vi "ControlProgram5.1.vi"() -> ()   [LabVIEW 2016]
uses:
  <vilib>/Utility/error.llb/DialogType.ctl
  <vilib>/Utility/miscctls.llb/LVPoint32TypeDef.ctl
  <vilib>/DAQmx/write.llb/DAQmx Write (Digital Bool 1Line 1Point).vi
  <vilib>/DAQmx/create/channels.llb/DAQmx Create Channel (DO-Digital Output).vi
  <vilib>/platform/TimedLoop/XDataNode/XDataNode.xnode
  <vilib>/Platform/TimedLoop/XDataNode/nitl_modes.ctl
  <vilib>/Platform/TimedLoop/XDataNode/XDNodeRunTimeDep.lvlib
  <vilib>/Platform/TimedLoop/XDataNode/wakeup.ctl
  <vilib>/Platform/TimedLoop/XDataNode/timing_clust.ctl
  <vilib>/DAQmx/create/channels.llb/DAQmx Create Channel (AI-Voltage-Basic).vi
  <vilib>/DAQmx/create/channels.llb/DAQmx Create Channel (AO-Voltage-Basic).vi
  <vilib>/DAQmx/write.llb/DAQmx Write (Analog 1D DBL NChan 1Samp).vi
  <resource>/objmgr/daqmx.rc
  <vilib>/Analysis/NI_AALBase.lvlib
  <vilib>/Analysis/baseanly.llb/Mean (DBL).vi
  <vilib>/Instr/_visa.llb/VISA Configure Serial Port (Instr).vi
  <vilib>/DAQmx/read.llb/DAQmx Read (Analog 2D DBL NChan NSamp).vi
  <vilib>/Utility/inputDevices.llb/closeMouse.vi
  <vilib>/Utility/inputDevices.llb/mouseAcquire.vi
  <vilib>/DAQmx/configure/timing.llb/DAQmx Timing (Sample Clock).vi
panel:
  out "Flush Sample Start Time":u32
  out "Sample flush time (s)":dbl=100.0
  in  "Inject Sample":bool
  out "Chart Freq (Hz)":dbl
  out "Waveform Chart 3":dbl[][](graph)
  out "Cal values":T1={"AX alpha"=672.9952101249002, "BX alpha"=822.8320399167465, "AX kappa"=0.3432739170419873, "BX kappa"=0.22087046979741862, "AX offset"=-0.002065833400375715, "BX offset"=0.010483360643544744, "AY alpha"=702.0654168010462, "BY alpha"=773.6701766674906, "AY kappa"=0.33643150106915, "BY kappa"=0.2444549177225145, "AY offset"=-0.1177594339643395, "BY offset"=0.06470506082263472}
  in  "Inject Pump 1":bool
  in  "Inject Pump 2":bool
  in  "Tab Control 2":T2(tab)
  in  "Force FB script":bool
  in  "Got ADig bead":bool
  in  "Move Cap. 2 (ADig Top)":bool
  in  "Dump beads":bool
  in  "Got DNA bead":bool
  in  "Delta after tether":dbl=3.1
  in  "TA Cancel Save?":bool
  in  "Min fish\ndelta (V)":dbl=2.8 min=0.0 max=10.0 step=0.1
  in  "Max fish\ndelta (V)":dbl=3.8 min=0.0 max=10.0 step=0.1
  in  "Fish Speed (ms)":i32=3000
  in  "Wait (ms)":i32=1500
  in  "# attempts":dbl=10.0
  in  "Cutoff force (pN)":dbl=5.0
  in  "Raster after\n tether?":bool=TRUE
  out "Tether":bool
  out "Attempt #":i32
  in  "Cal @ Delta (V)":dbl=5.0
  in  "Cal stage position":i32=3
  in  "Conv Y (nm/V)":dbl=505.0
  in  "Conv X (nm/V)":dbl=892.0
  out "Cal Final Sampling Rate":dbl
  in  "Cal Averaging":i32=1
  in  "Wait before dip (s)":dbl=3.0
  in  "Start dipping after?":bool
  in  "Start trap delta (V)":dbl=3.85
  in  "Cancel dwell":bool
  in  "Pause dwell":bool
  in  "Return position":dbl=3.0
  in  "Dip duration":dbl=15.0
  in  "Dip position":dbl=4.0
  in  "Dip":bool
  out "Dip time":i32
  in  "Stop":bool=TRUE
  in  "?":T3(tab)=enum."Mouse control"
  in  "Save N sets":bool
  in  "N sets":i32=200
  in  "Cal sets to save":i32=500
  in  "Reset data stream":bool
  out "Buffer Overflow":bool
  out "Stage moving":bool
  in  "Comment":string="wtUvrD 0.5 uM ATP"
  in  "Raster scan":bool
  out "Saving":bool
  in  "Save cal":bool
  in  "Save Data":bool
  in  "Stop saving":bool
  out "Calibrating":bool
  out "Progress":dbl(slide) scale=0.0..100.0
  in  "Read Cal":bool
  in  "Fish":bool
  in  "Averaging Number":i32=1250
  out "Final Sampling Rate":dbl=100.0
  in  "Trap position":cluster{"X":dbl, "Y":dbl}={"X"=1.6, "Y"=4.95}
  in  "Trap delta":dbl=5.1 min=0.0 max=10.0 step=0.1
  in  "Fixed X":dbl=1.6
  in  "Fixed Y":dbl=0.7
  in  "Shutter 1 (B)":bool
  in  "Shutter 2 (A)":bool
  in  "Pulling direction":bool=TRUE
  out "Raster scanning...":bool
  out "Current file name":path
  in  "AX alpha":dbl format="%#_3p"
  in  "BX alpha":dbl format="%#_3g"
  in  "AX kappa":dbl format="%#_3g"
  in  "BX kappa":dbl format="%#_3g"
  in  "AX offset":dbl format="%#_3g"
  in  "BX offset":dbl format="%#_3g"
  in  "AY alpha":dbl format="%#_3g"
  in  "BY alpha":dbl format="%#_3g"
  in  "AY kappa":dbl format="%#_3g"
  in  "BY kappa":dbl format="%#_3g"
  in  "AY offset":dbl format="%#_3g"
  in  "BY offset":dbl format="%#_3g"
  out "Buffer status":u8(slide) scale=0.0..100.0
  in  "dump spot":string="Dump beads spot"
  in  "up flow spot":string="Upper flow spot"
  in  "low flow spot":string="Lower flow spot"
  in  "up cap":string="Upper capillary (ADig beads)"
  in  "bottom cap":string="Lower capillary (DNA beads)"
  in  "Move to Position 5":bool
  in  "Set Position 5":bool
  in  "Saved stage positions":dbl[][](array[numeric])=[[1.0, 0.0, 0.0, 0.0], [2.0, 0.28481, -2.63158, -0.02256], [3.0, 1.27978, -0.73974, 0.0], [4.0, 1.27978, -2.1978, 0.0], [5.0, 0.03306, -2.63158, -0.02256]]
  in  "Set Position 2":bool
  in  "Move to Position 2":bool
  in  "Set Position 1":bool
  in  "Move to Position 1":bool
  in  "Set Position 4":bool
  in  "Move to Position 4":bool
  in  "Set Position 3":bool
  in  "Move to Position 3":bool
  out "Stage error":errorcluster
  in  "Clear Volume":bool
  out "Sample Flush Meter":u8(slide) scale=0.0..100.0
  out "Flushing Sample":bool
  in  "Flush Sample":bool
  in  "Normal \nRate (ul/hr)  3":dbl=100.0
  in  "Normal \nVolume (ul) 3":dbl=300.0
  in  "Normal \nVolume (ul) 2":dbl
  in  "Normal \nRate (ul/hr)":dbl
  in  "Normal \nVolume (ul)":dbl
  in  "Flush\nRate (ul/min)":dbl
  in  "Flush\nVolume (ul)":dbl
  in  "Flush \nRate (ul/min)  2":dbl
  in  "Flush Pump 2":bool
  in  "Flush\nVolume (ul)  2":dbl
  in  "Flush Pump 1":bool
  in  "Normal \nRate (ul/hr)  2":dbl
  in  "Write Wait":i32=1000
  in  "Flush \nRate (ul/min)  3":dbl=100.0
  in  "Flush\nVolume (ul)  3":dbl=100.0
  out "error out":errorcluster
  in  "Use Mouse to Move Trap?":bool
  in  "Pause Mouse/Mirror Connection":bool
  out "Reference Voltage":cluster{dbl, dbl}={0.0, -0.0}
  out "Saved voltage":cluster{dbl, dbl}
  out "Real Coordinates":cluster{"Horizontal":i32, "Vertical":i32}={"Horizontal"=145, "Vertical"=-1746}
  out "CoordinatesMousePressed":T4
  out "Sum error":dbl(knob) scale=-0.2..0.2
  out "Trap sep":waveform(dbl)[](graph)
  in  "Set reading to\nsetpoint":bool
  in  "Offset Y (nm)":dbl format="%0.2f"
  in  "Offset X (nm)":dbl format="%0.2f"
  in  "Remove offsets":bool
  in  "Force Feedback":bool
  out "Feedback Output Voltage 2":cluster{dbl, dbl} {"?" format="%#_4g"; "?" format="%#_4g"}
  in  "Max value X":dbl=10.0 format="%.1f"
  in  "Min value X":dbl format="%0.1f"
  in  "Max value Y":dbl=10.0 format="%.1f"
  in  "Min value Y":dbl format="%.1g"
  in  "Offset":cluster{"Off Y":dbl, "Off X":dbl}={"Off Y"=1.5, "Off X"=0.17}
  in  "Setpoint voltage":cluster{"SP Y":dbl, "SP X":dbl}={"SP Y"=0.6, "SP X"=0.0}
  in  "Feedback const":T5={"Ki_B_Y"=0.5, "Ki_B_X"=0.0, "Kp Y"=1.0, "Kp X"=0.0}
  out "Mean Trap Pos X 2 (nm)":dbl format="%0.2f"
  out "Mean Trp Pos Y 2 (nm)":dbl format="%0.2f"
  out "T2 X RMS (A)":dbl format="%0.2f"
  out "T2 Y RMS (A)":dbl format="%0.2f"
  in  "Save scans":bool=TRUE
  in  "# scans":i32=1
  in  "Speed (ms)":i32=10000
  in  "Min delta":dbl=3.2
  in  "Load param":bool
  in  "Max delta":dbl=4.1
  in  "Scan Parameters":T6(array[cluster])=[{"Label"="Offset", "Max delta 2"=3.8, "Min delta 2"=2.4, "Speed (ms) 2"=10000, "# scans 2"=1}]
  in  "Trap delta\nafter":dbl=3.6
  in  "Stop raster":bool
  out "Scan Range (nm)":dbl
  out "Scan Speed (nm/s)":dbl
  out "Continue to display?":bool
  out "Video Error":errorcluster
  in  "# Samples/channel (in)":i32=40000 format="%.2f"
  out "Buffer size\n(Samples/channel)":u32
  out "DAQ rate\n(Samples/s)":dbl format="%#_6p"
  out "# Samples/channel":i32=1250
  out "# Samples/channel/s":dbl
  out "AvailSampPerChan":u32
  out "Data update period (s/set)":dbl format="%#_6p"
  out "AvailSampPerChan 2":u32
  in  "PC samp per channel":i32=1000
  in  "Sampling Rate":dbl=125000.0 format="%0.0p"
  in  "DAQ Rate2":dbl=1000000.0 format="%#_6p"
  out "Data period (s)":dbl format="%#_6p"
  in  "Tether break\nforce (pN)":dbl=1.0
  in  "Path":path=path "D:/data"
  in  "Save file index":dbl
  out "Mirror task":refnum<k21>
  in  "HWP1":string="Half waveplate 1: differential trap power"
  in  "HWP0":string="Half waveplate 0: total trap power"
  in  "Move 1":bool
  in  "\"Degrees\" 1":dbl
  in  "Move 0":bool
  in  "\"Degrees\" 0":dbl
  out "Chamber":T7(plugin-control)
  out "Deflection":T4
  in  "Sampling Rate":dbl=125000.0 format="%0.2f"
  in  "Averaging Number":i32=12500
  in  "DAQ Rate":dbl=1000000.0
  out "Final Sampling Rate":dbl
  in  "Tab Control":T8(tab)
  in  "Downsamp\nfact":dbl=250.0
  out "Bead sep":waveform(dbl)[](graph)
  out "Force (pN)":waveform(dbl)[](graph)
  out "Mean force (pN)":dbl format="%0.2f"
  out "Force noise (pN)":dbl format="%0.2f"
  out "Mean Bead Sep\n(nm)":dbl format="%0.2f"
  out "Bead Sep Noise\n(A)":dbl format="%0.2f"
  out "PSD 2":cluster{dbl[], dbl[]}(graph)
  out "PSD 1":cluster{dbl[], dbl[]}(graph)
  out "PSD 1 Sum":dbl(slide) scale=0.0..10.0
  out "PSD 2 Sum":dbl(slide) scale=0.0..10.0
  in  "Start":bool
  out "All signals":waveform(dbl)[](graph)
  # "Bead Calibration"
  # "X"
  # "Y"
  # "Pump #1 Controls"
  # "Pump #2 Controls"
  # "Sample Pump Controls"
  # "Retract the pumps manually. Change it back to INFUSE when you're done. Suck it up, don't whine."
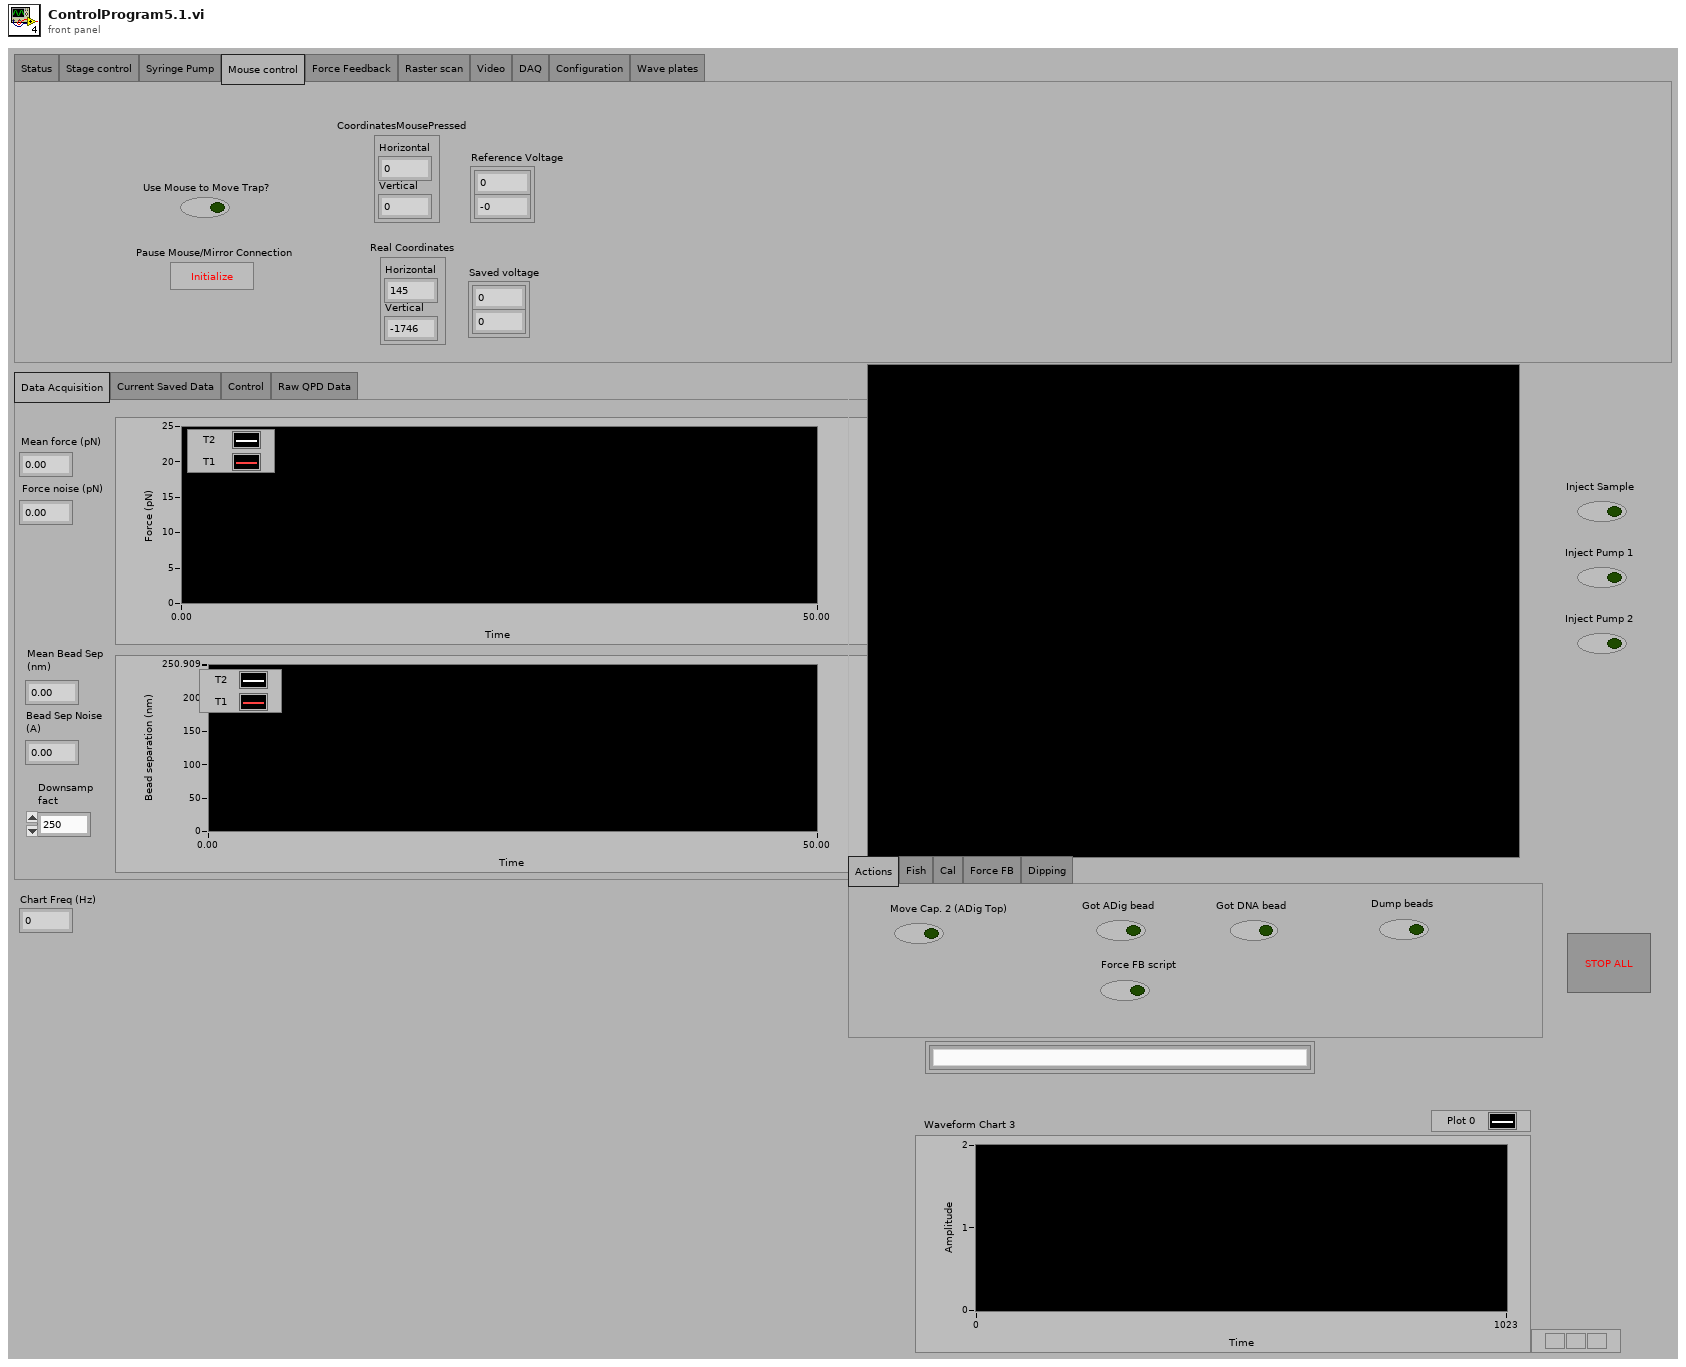
[diagram p1: front panel]
types:
  T1 = cluster{"AX alpha":dbl, "BX alpha":dbl, "AX kappa":dbl, "BX kappa":dbl, "AX offset":dbl, "BX offset":dbl, "AY alpha":dbl, "BY alpha":dbl, "AY kappa":dbl, "BY kappa":dbl, "AY offset":dbl, "BY offset":dbl}
  T2 = enum32{"Actions", "Fish", "Cal", "Force FB", "Dipping"}
  T3 = enum32{"Status", "Stage control", "Syringe Pump", "Mouse control", "Force Feedback", "Raster scan", "Video", "DAQ", "Configuration", "Wave plates"}
  T4 = typedef "LVPoint32TypeDef.ctl" = cluster{"Horizontal":i32, "Vertical":i32}
  T5 = cluster{"Ki_B_Y":dbl, "Ki_B_X":dbl, "Kp Y":dbl, "Kp X":dbl}
  T6 = cluster{"Label":string, "Max delta 2":dbl, "Min delta 2":dbl, "Speed (ms) 2":i32, "# scans 2":i32}[]
  T7 = typedef "IMAQ Image.ctl" = refnum<image>
  T8 = enum32{"Data Acquisition", "Current Saved Data", "Control", "Raw QPD Data"}
  T9 = enum16{"open", "replace", "create", "open or create", "replace or create", "replace or create with confirmation"}
  T10 = enum16{"big-endian, network order", "native, host order", "little-endian"}
  T11 = cluster{string, string, string, string, string, string, string, string}
  T12 = typedef "XDNodeRunTimeDep.lvlib/timing_clust.ctl" = cluster{"Expected End [f-1]":u64, "Actual End [f-1]":u64, "Finished Late? [f-1]":bool, "Expected End [i-1]":u64, "Actual End [i-1]":u64, "Finished Late? [i-1]":bool, "Expected Start [i]":u64, "Actual Start [i]":u64, "Expected Start [f]":u64, "Actual Start [f]":u64, "Source Name":string, "Structure Name":string, "Period":i64, "Deadline":i64, "Offset":i64, "Start":i64, "Priority":i32, "Timeout":i32, "Mode":T13, "Wakeup Reason":T14, "Error":errorcluster, "Source Type":string, "Secondary Source Type":string, "Global End Time":u64, "Global Start Time":u64, "Frame Duration":u64, "Iteration Duration":u64, "Assigned CPU":i32, "I/O Scan Engine Mode":u32}
  T13 = typedef "XDNodeRunTimeDep.lvlib/nitl_modes.ctl" = enum32{"No Change", "Process missed periods, maintain original phase", "Discard missed periods, maintain original phase", "Process missed periods, ignore original phase", "Discard missed periods, ignore original phase"}
  T14 = typedef "XDNodeRunTimeDep.lvlib/wakeup.ctl" = enum32{"Normal", "Aborted", "Asynchronous wakeup", "Timing source error", "Timed loop error", "Timeout"}
  T15 = typedef "DialogType.ctl" = u16
  T16 = cluster{"button 1":bool, "button 2":bool, "button 3":bool, "button 4":bool}
  T17 = cluster{"[0]":dbl, "[1]":dbl, "[2]":dbl, "[3]":dbl, "[4]":dbl, "[5]":dbl, "[6]":dbl, "[7]":dbl, "[8]":dbl, "[9]":dbl, "[10]":dbl, "[11]":dbl}
  T18 = cluster{"Label":string, "Max delta 2":dbl, "Min delta 2":dbl, "Speed (ms) 2":i32, "# scans 2":i32}
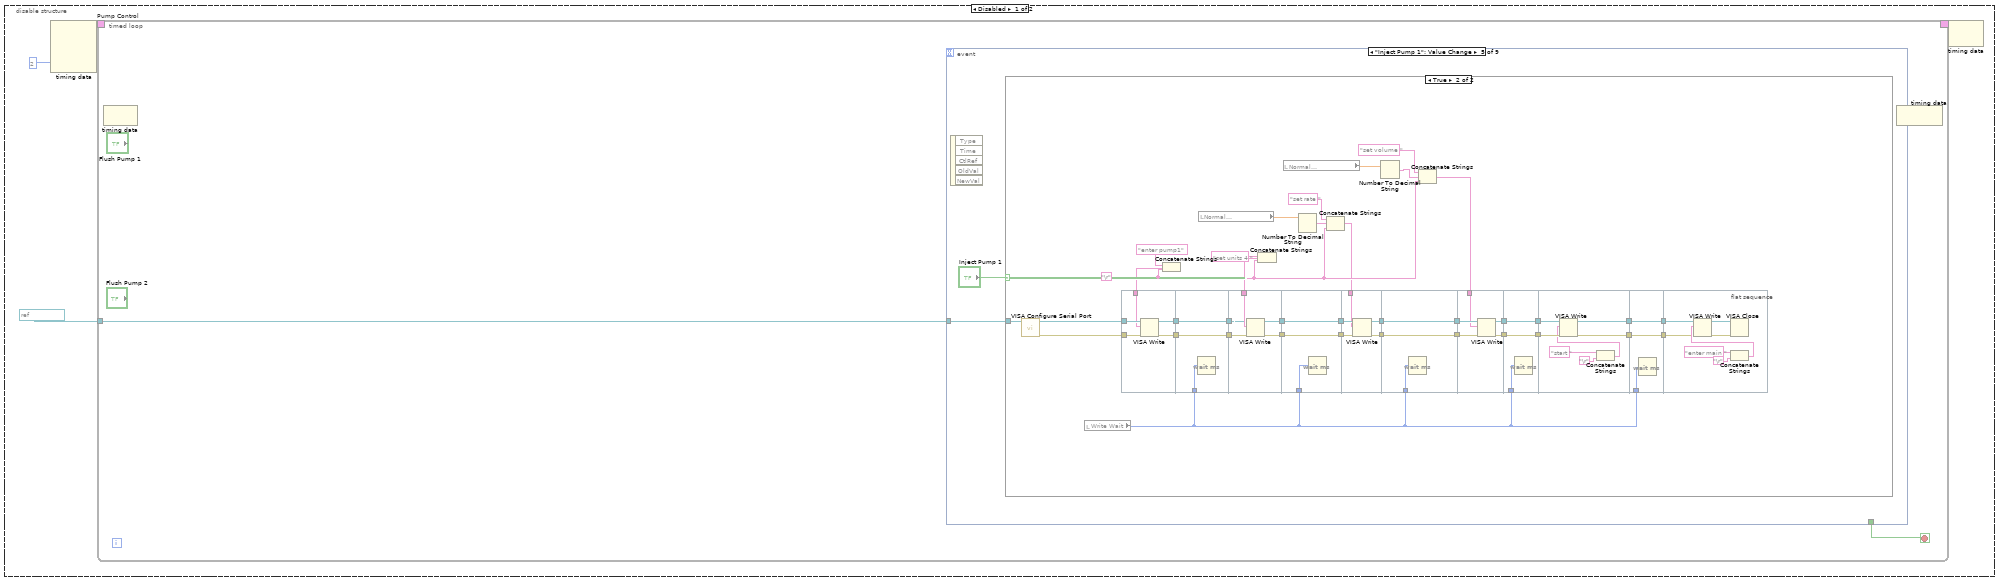
[diagram p2: hidden frame]
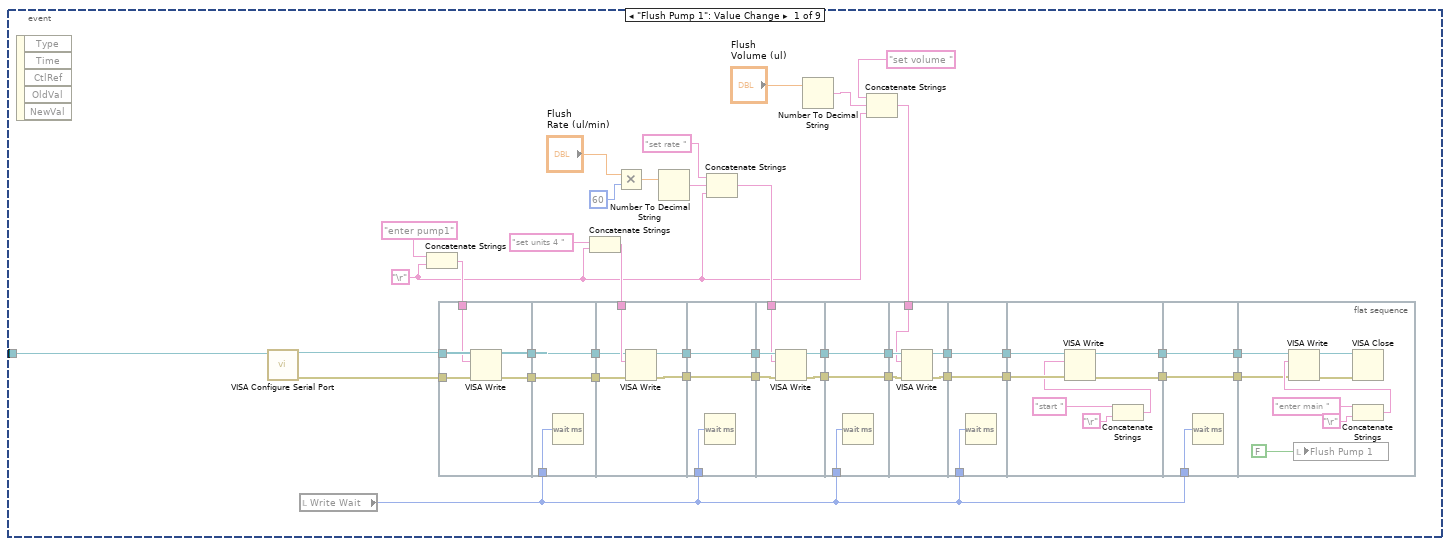
[diagram p3: hidden frame]
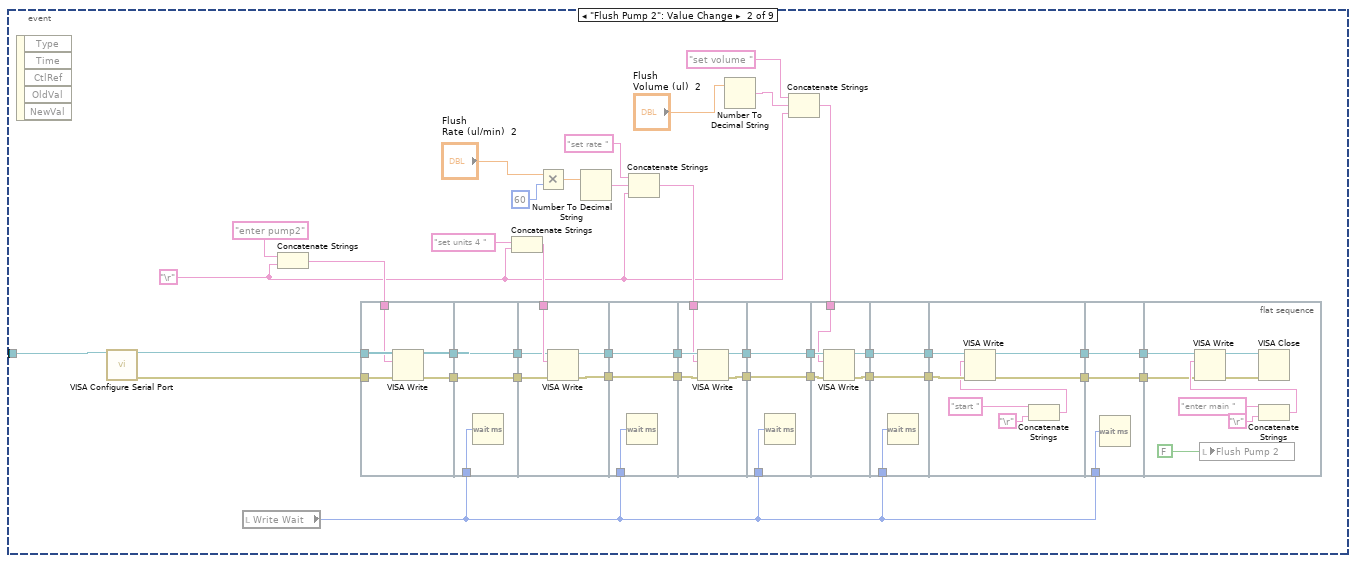
[diagram p4: hidden frame]
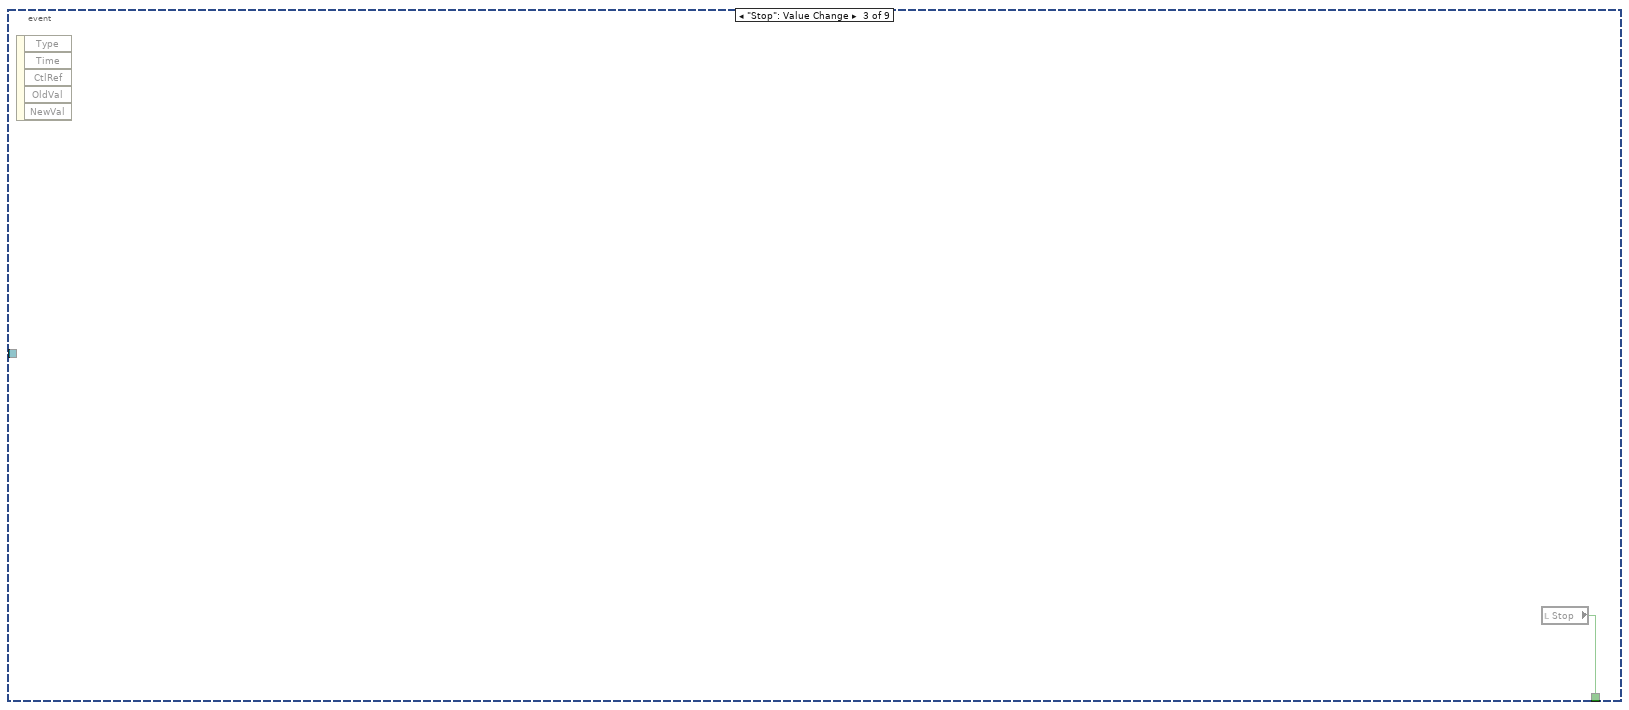
[diagram p5: hidden frame]
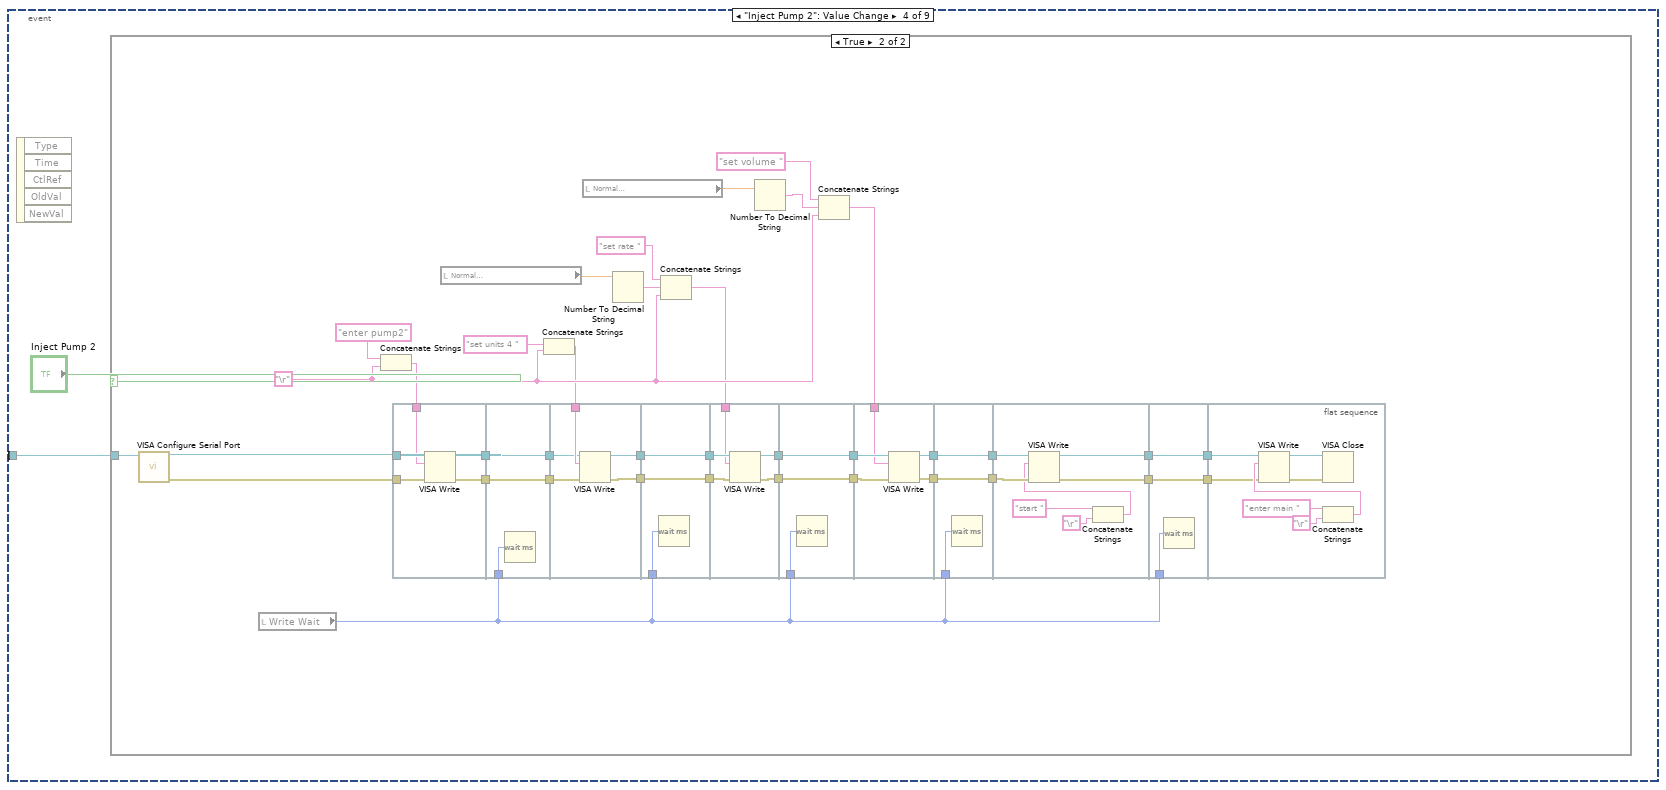
[diagram p6: hidden frame]
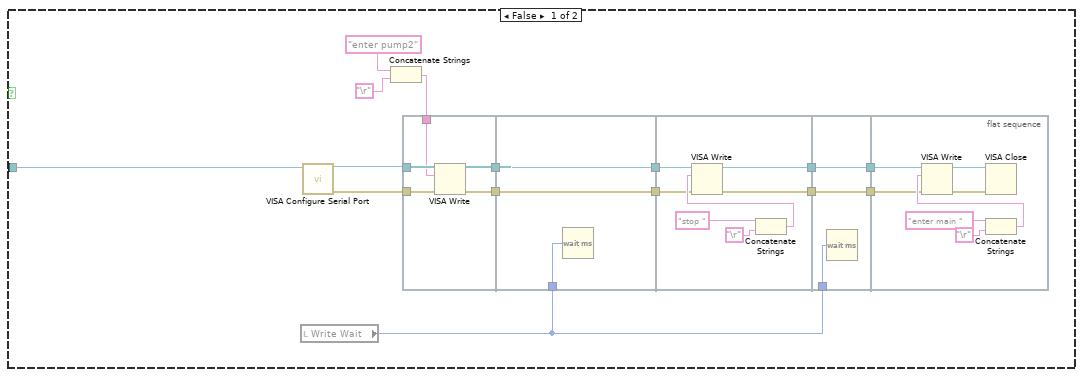
[diagram p7: hidden frame]
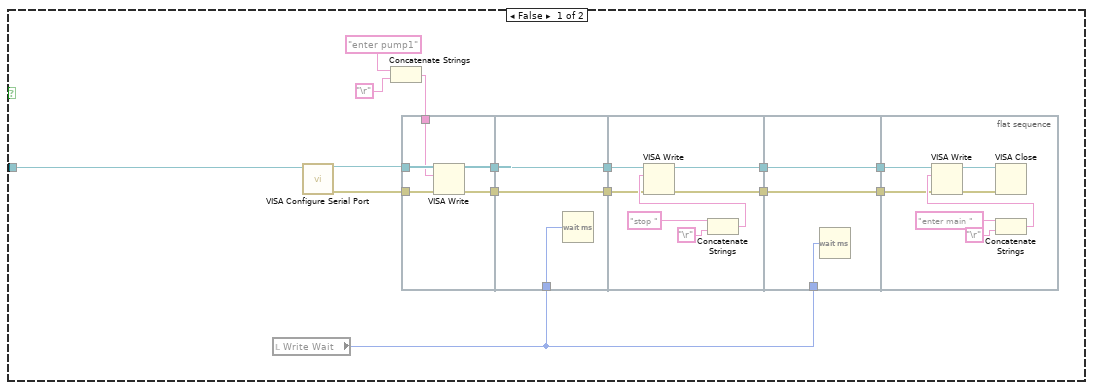
[diagram p8: hidden frame]
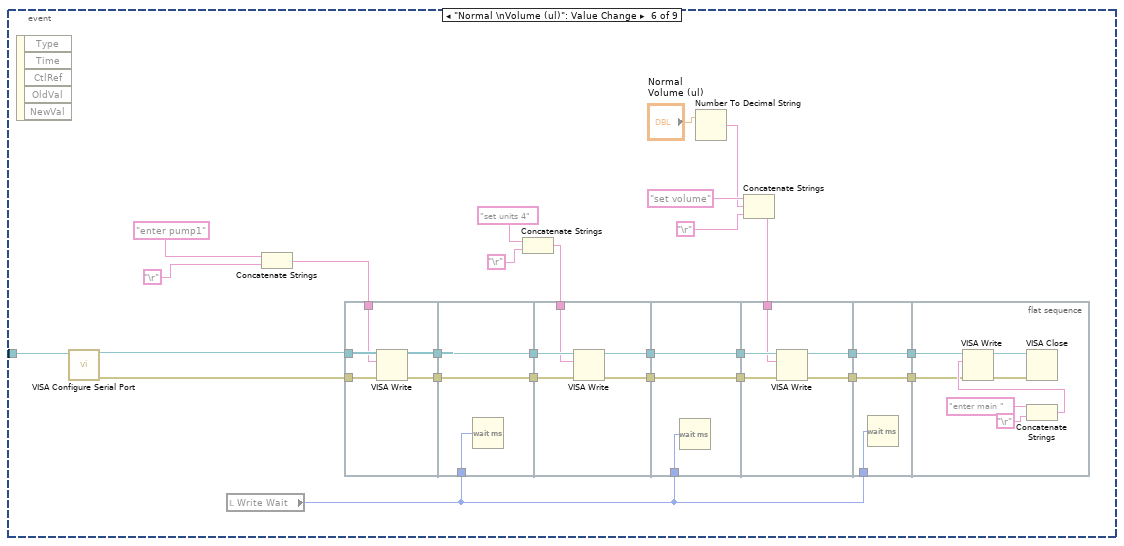
[diagram p9: hidden frame]
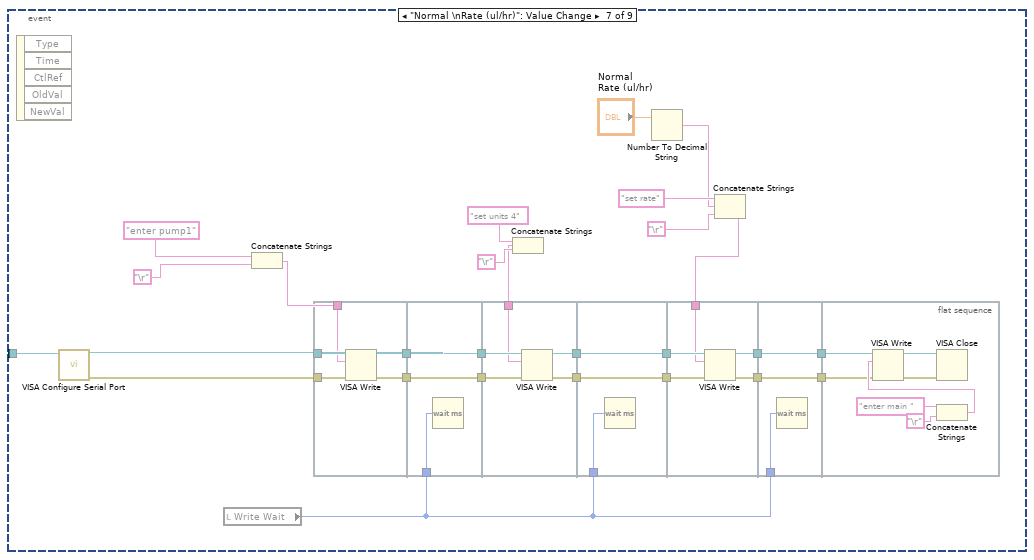
[diagram p10: hidden frame]
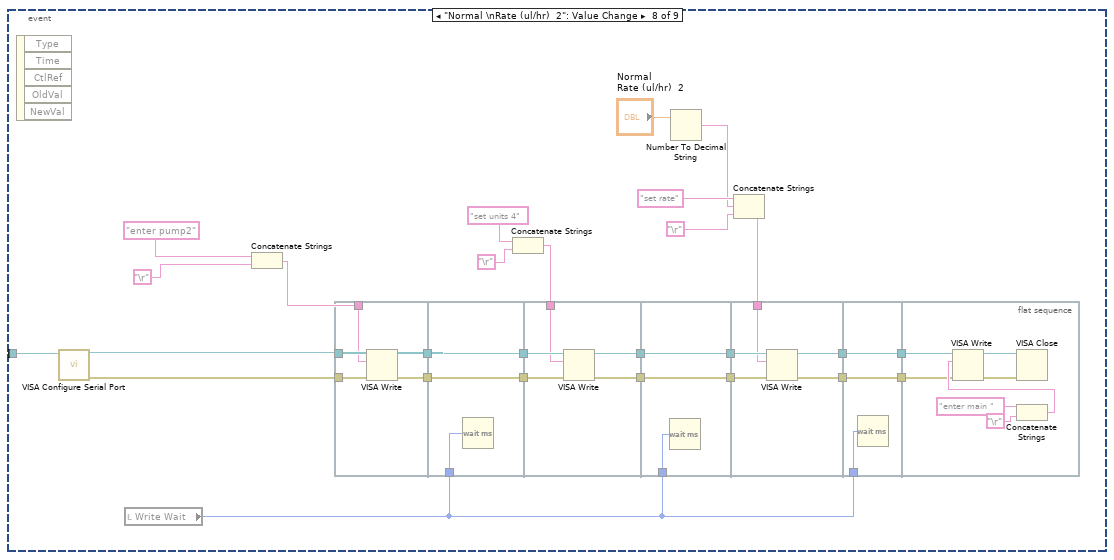
[diagram p11: hidden frame]
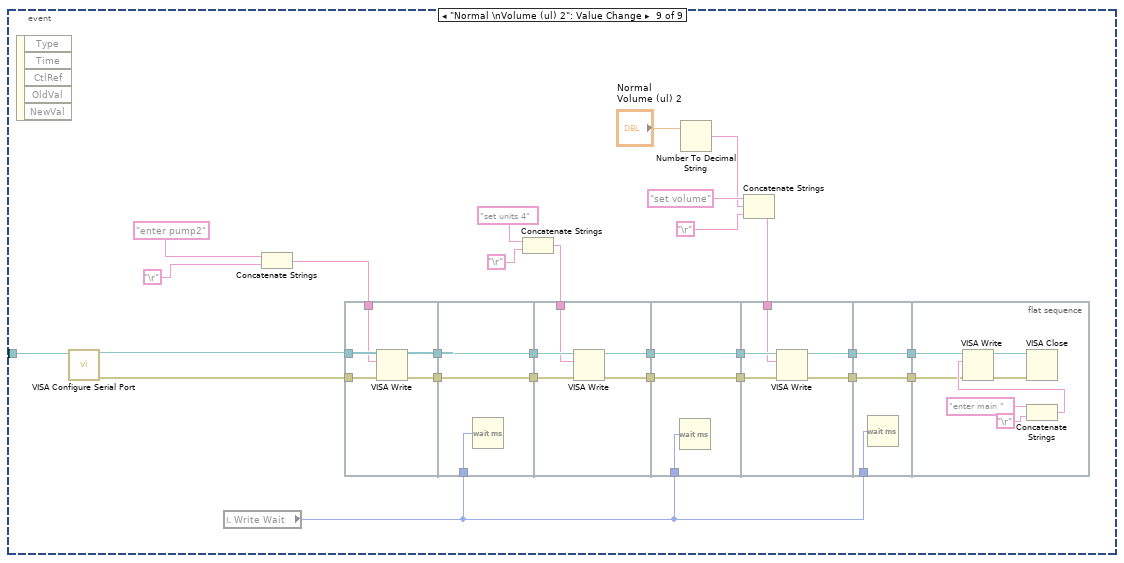
[diagram p12: hidden frame]
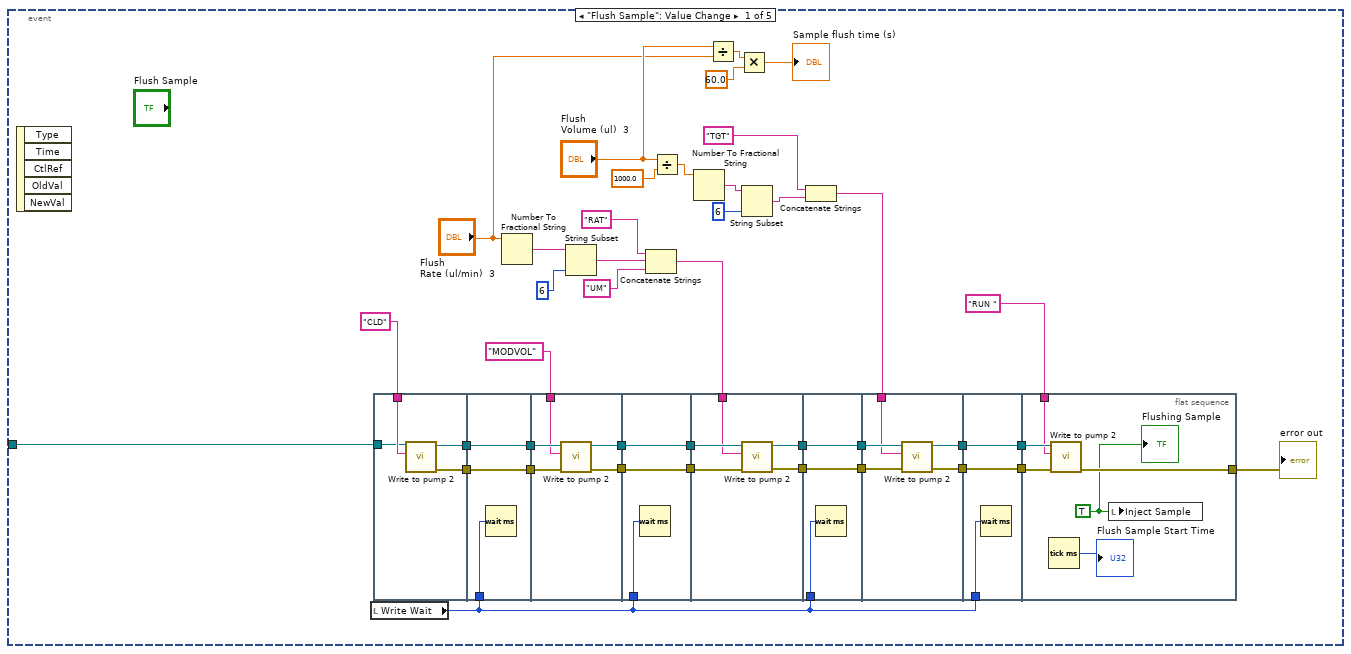
[diagram p13: hidden frame]
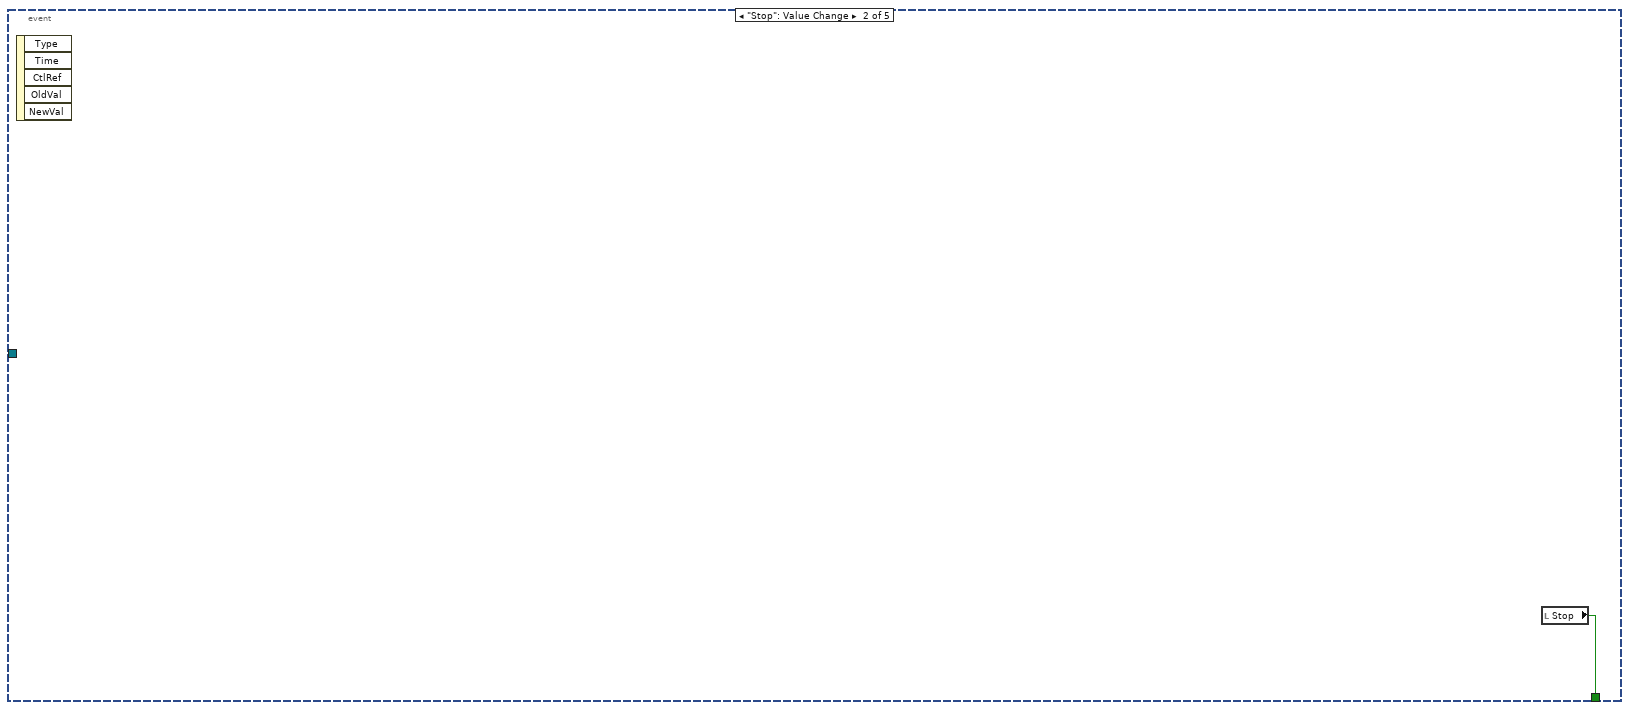
[diagram p14: hidden frame]
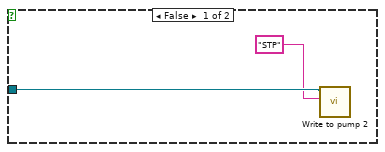
[diagram p15: hidden frame]
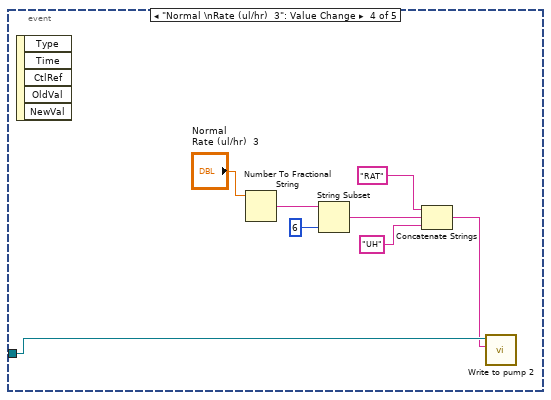
[diagram p16: hidden frame]
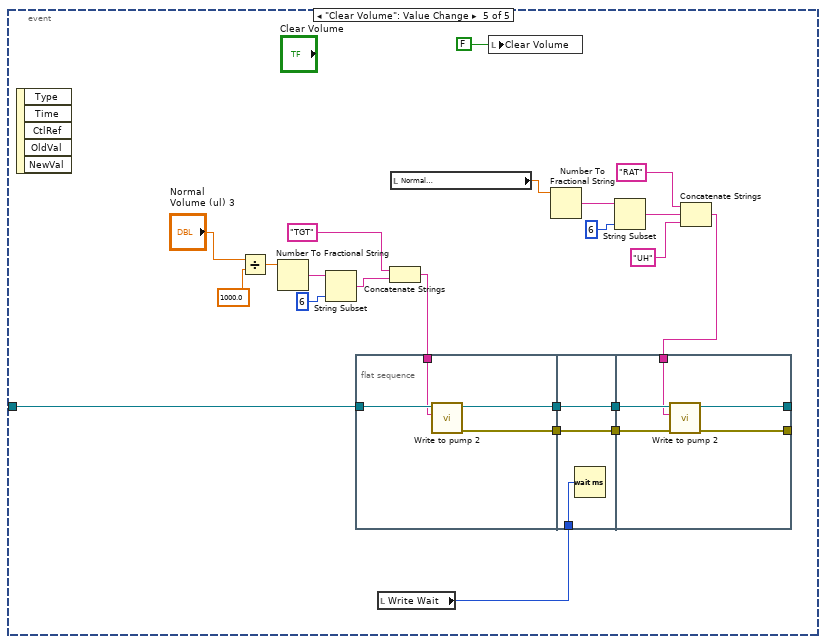
[diagram p17: hidden frame]
diagram:
  w42 = 10.0 ("Minimum Value")
  w43 = -10.0 ("Minimum Value")
  w45 = -2.0 ("Minimum Value")
  w46 = 2.0 ("Maximum Value")
  w71 = 10123 items=["Finite Samples"=10178, "Continuous Samples"=10123] ("sample mode")
  w92 = tag "Dev1/port2/line1"  # Shutter 2
  w95 = tag "Dev1/port1/line4"  # Shutter 1
  # "Create channels for movable mirror"
  # "Create channels for detectors"
  n1 = call-poly <vilib>:"DAQmx Create Virtual Channel.vi"("maximum value"=w46, "minimum value"=w45, "physical channels"=tag "Dev1/ai0" ("Physical Channel")) -> ("task out"=w47:refnum<k21>, "error out"=w70:errorcluster)  [unwired: 11 in]
  n2 = call-poly <vilib>:"DAQmx Create Virtual Channel.vi"("task in"=w47, "maximum value"=w46, "minimum value"=w45, "physical channels"=tag "Dev1/ai1", "error in"=w70) -> ("task out"=w68:refnum<k21>, "error out"=w67:errorcluster)  [unwired: 9 in]
  n3 = call-poly <vilib>:"DAQmx Create Virtual Channel.vi"("task in"=w68, "maximum value"=w46, "minimum value"=w45, "physical channels"=tag "Dev1/ai2", "error in"=w67) -> ("task out"=w59:refnum<k21>, "error out"=w58:errorcluster)  [unwired: 9 in]
  n4 = call-poly <vilib>:"DAQmx Create Virtual Channel.vi"("task in"=w59, "maximum value"=w46, "minimum value"=w45, "physical channels"=tag "Dev1/ai3" ("Physical Channel"), "error in"=w58) -> ("task out"=w44:refnum<k21>, "error out"=w64:errorcluster)  [unwired: 9 in]
  n5 = call-poly <vilib>:"DAQmx Create Virtual Channel.vi"("task in"=w44, "maximum value"=w42, "minimum value"=w43, "physical channels"=tag "Dev1/ai4", "error in"=w64) -> ("task out"=w62:refnum<k21>, "error out"=w61:errorcluster)  [unwired: 9 in]
  n6 = call-poly <vilib>:"DAQmx Create Virtual Channel.vi"("task in"=w62, "maximum value"=w42, "minimum value"=w43, "physical channels"=tag "Dev1/ai5", "error in"=w61) -> ("task out"=w57:refnum<k21>, "error out"=w56:errorcluster)  [unwired: 9 in]
  n7 = call-poly <vilib>:"DAQmx Create Virtual Channel.vi"("task in"=w57, "maximum value"=w42, "minimum value"=w43, "physical channels"=tag "Dev1/ai6", "error in"=w56) -> ("task out"=w51:refnum<k21>, "error out"=w49:errorcluster)  [unwired: 9 in]
  n8 = call-poly <vilib>:"DAQmx Create Virtual Channel.vi"("task in"=w51, "maximum value"=w42, "minimum value"=w43, "physical channels"=tag "Dev1/ai7", "error in"=w49) -> ("task out"=w50:refnum<k21>, "error out"=w48:errorcluster)  [unwired: 9 in]
  n9 = call-poly <vilib>:"DAQmx Timing.vi"("task/channels in"=w50, "sample mode"=w71, "samples per channel"="PC samp per channel", "rate"="Sampling Rate", "error in"=w48) -> ("task out"=w54:refnum<k21>, "error out"=w53:errorcluster)  [unwired: 9 in]
  n10 = call-poly <vilib>:"DAQmx Create Virtual Channel.vi"("maximum value"="Max value Y", "minimum value"="Min value Y", "physical channels"=tag "Dev1/ao1" ("Trap X Axis")) -> ("task out"=w39:refnum<k21>, "error out"=w41:errorcluster)  [unwired: 11 in]
  n11 = property class="DAQmx Timing"(reference=w54, error in=w53, "More:AI Convert:Rate"="DAQ Rate2") -> (reference out=w6:refnum<k21>, error out=w5:errorcluster, "SampClk.Rate"=→"DAQ rate\n(Samples/s)":dbl)
  n12 = call-poly <vilib>:"DAQmx Create Virtual Channel.vi"("task in"=w39, "maximum value"="Max value X", "minimum value"="Min value X", "physical channels"=tag "Dev1/ao0" ("Trap Y Axis"), "error in"=w41) -> ("task out"=w30:refnum<k21>, "error out"=w29:errorcluster)  [unwired: 9 in]
  "Mirror task" <- w30
  n13 = property class="DAQmx Buffer"(reference=w6, error in=w5) -> (reference out=w3:refnum<k21>, error out=w2:errorcluster, "Input.OnbrdBufSize"=→"Buffer size\n(Samples/channel)":u32)
  n14 = call <vilib>:"DAQmx Start Task.vi"("task/channels in"=w3, "error in"=w2) -> ("task out"=w31:refnum<k21>)  [unwired: 12 in, 1 out]
  n15 = while {
    tunnel: [w414] -> w77
    tunnel: [w306] -> w78
    tunnel: [w422] -> w76
    tunnel: [w419] -> w73
    tunnel: w31 -> [w118]
    tunnel: w30 -> [w415]
    tunnel: w29 -> [w420]
    stop <- w419 stop-if-true
    w149 = "NI_ChannelName" ("name")
    w226 = -1
    # "Rewire everything"
    # "Invert these because changed\nfrom PSD to QPD"
    # "Trap Y"
    # "Trap X"
    # "Convert to\npN"
    # "Convert to\nnm"
    # "Subtract\noffset"
    # "Normalize by\nsum"
    # "B sum"
    # "BX"
    # "BY"
    # "AX"
    # "AY"
    # "A sum"
    # "Close files when done saving"
    n16 = property class="DAQmx Read"(reference=w118) -> (reference out=w117:refnum<k21>, "AvailSampPerChan"=→"AvailSampPerChan 2":u32)  [unwired: 1 in, 1 out]
    n17 = local read "Averaging Number"() -> (w113:i32)
    n18 = local read "Averaging Number"() -> (w119:i32)
    "# Samples/channel" <- w119
    n19 = local read "Sampling Rate"() -> (w418:dbl)
    n20 = call-poly <vilib>:"DAQmx Read.vi"("task/channels in"=w117, "number of samples per channel"=w113, "timeout"=10.0) -> ("task out"=w305:refnum<k21>, "data"=w114:dbl[][], "error out"=w229:errorcluster)  [unwired: 10 in]
    n21 = Unbundle By Name(w229) -> ("status"=w354:bool)
    n22 = Divide(x=w418, y="Cal Averaging") -> (x/y=→"Cal Final Sampling Rate":dbl)
    n23 = Divide(x=w418, y=w119) -> (x/y=→"Final Sampling Rate" →"# Samples/channel/s":dbl)
    n24 = case shown="True" w354 {
      frame False {
      }
      frame True {
        n25 = call <vilib>:"Beep.vi"() -> ()  [unwired: 12 in]
        "Buffer Overflow" <- TRUE
      }
    }
    n26 = local read "Buffer size\n(Samples/channel)"() -> (w301:u32)
    n27 = property class="DAQmx Read"(reference=w305) -> (reference out=w304:refnum<k21>, "AvailSampPerChan"=w302:u32)  [unwired: 1 in, 1 out]
    "AvailSampPerChan" <- w302
    n28 = local read "Cal values"() -> (w346:T1)
    n29 = Index Array(array=w114, index (row)=4) -> (element=w218:dbl[])  [unwired: 1 in]
    n30 = Index Array(array=w114, index (row)=0) -> (element=w228:dbl[])  [unwired: 1 in]
    n31 = Index Array(array=w114, index (row)=2) -> (element=w223:dbl[])  [unwired: 1 in]
    n32 = Index Array(array=w114, index (row)=1) -> (element=w227:dbl[])  [unwired: 1 in]
    n33 = Index Array(array=w114, index (row)=3) -> (element=w221:dbl[])  [unwired: 1 in]
    n34 = Index Array(array=w114, index (row)=6) -> (element=w220:dbl[])  [unwired: 1 in]
    n35 = Index Array(array=w114, index (row)=7) -> (element=w219:dbl[])  [unwired: 1 in]
    n36 = Index Array(array=w114, index (row)=5) -> (element=w217:dbl[])  [unwired: 1 in]
    n37 = Divide(x=w302, y=w301) -> (x/y=→"Buffer status":dbl)
    n38 = Unbundle(w346) -> ("AX alpha"=w334:dbl, "BX alpha"=w330:dbl, "AX kappa"=w326:dbl, "BX kappa"=w322:dbl, "AX offset"=w340:dbl, "BX offset"=w338:dbl, "AY alpha"=w337:dbl, "BY alpha"=w332:dbl, "AY kappa"=w328:dbl, "BY kappa"=w324:dbl, "AY offset"=w344:dbl, "BY offset"=w342:dbl)
    n39 = Multiply(x=w227, y=w226) -> (x*y=w222:dbl[])
    n40 = Multiply(x=w228, y=w226) -> (x*y=w224:dbl[])
    n41 = local write "AX alpha"(w334) -> ()
    n42 = local write "BY offset"(w342) -> ()
    n43 = Build Array(w224, w223, w222, w221, w220, w219, w218, w217) -> (w146:dbl[][])
    n44 = local write "BX alpha"(w330) -> ()
    n45 = case shown="True" "Reset data stream" {
      selector: "Reset data stream" -> [_ w465]
      tunnel: w304 -> [w457 w463]
      tunnel: [w457 w461] -> w306
      tunnel: w229 -> [w456 w460]
      tunnel: [w456 w458] -> _
      frame False {
      }
      frame True {
        n46 = Not(x=w465) -> (.not. x?=w464:bool)
        n47 = call <vilib>:"DAQmx Stop Task.vi"("task/channels in"=w463, "error in"=w460) -> ("task out"=w462:refnum<k21>, "error out"=w459:errorcluster)  [unwired: 12 in]
        n48 = local write "Reset data stream"(w464) -> ()
        n49 = local write "Buffer Overflow"(w464) -> ()
        n50 = call <vilib>:"DAQmx Start Task.vi"("task/channels in"=w462, "error in"=w459) -> ("task out"=w461:refnum<k21>, "error out"=w458:errorcluster)  [unwired: 12 in]
      }
    }
    n51 = call-poly <vilib>:"Mean.vi"("X"=w217) -> ("mean"=w360:dbl)  [unwired: 1 out]
    n52 = local write "AY offset"(w344) -> ()
    n53 = call-poly <vilib>:"Mean.vi"("X"=w218) -> ("mean"=w361:dbl)  [unwired: 1 out]
    n54 = call-poly <vilib>:"Mean.vi"("X"=w223) -> ("mean"=w367:dbl)  [unwired: 1 out]
    n55 = call-poly <vilib>:"Mean.vi"("X"=w221) -> ("mean"=w365:dbl)  [unwired: 1 out]
    n56 = call-poly <vilib>:"Mean.vi"("X"=w220) -> ("mean"=w364:dbl)  [unwired: 1 out]
    n57 = call-poly <vilib>:"Mean.vi"("X"=w219) -> ("mean"=w363:dbl)  [unwired: 1 out]
    n58 = local read "Averaging Number"() -> (w112:i32)
    n59 = local write "BY kappa"(w324) -> ()
    n60 = local write "AX kappa"(w326) -> ()
    n61 = call-poly <vilib>:"Mean.vi"("X"=w222) -> ("mean"=w366:dbl)  [unwired: 1 out]
    n62 = local write "AY kappa"(w328) -> ()
    n63 = call-poly <vilib>:"Mean.vi"("X"=w224) -> ("mean"=w368:dbl)  [unwired: 1 out]
    n64 = local read "DAQ rate\n(Samples/s)"() -> (w124:dbl)
    n65 = Build Array(w361, w360) -> (w359:dbl[])
    n66 = local write "BX kappa"(w322) -> ()
    n67 = local write "BY alpha"(w332) -> ()
    n68 = local write "AX offset"(w340) -> ()
    n69 = local write "BX offset"(w338) -> ()
    n70 = local write "AY alpha"(w337) -> ()
    n71 = Build Array(w368, w367, w366, w365, w364, w363) -> (w357:dbl[])
    n72 = Divide(x=w112, y=w124) -> (x/y=w121:dbl)
    "Data update period (s/set)" <- w121
    n73 = Reciprocal(x=w124) -> (1/x=w125:dbl)
    "Data period (s)" <- w125
    n74 = Divide(x=w368, y=w364) -> (x/y=w398:dbl)
    n75 = Divide(x=w367, y=w364) -> (x/y=w399:dbl)
    n76 = Divide(x=w366, y=w363) -> (x/y=w406:dbl)
    n77 = Divide(x=w365, y=w363) -> (x/y=w407:dbl)
    n78 = Subtract(x=w398, y="AY offset") -> (x-y=w380:dbl)
    n79 = Subtract(x=w399, y="AX offset") -> (x-y=w381:dbl)
    n80 = Subtract(x=w406, y="BY offset") -> (x-y=w379:dbl)
    n81 = Subtract(x=w407, y="BX offset") -> (x-y=w382:dbl)
    n82 = Subtract(x=w406, y=w398) -> (x-y=w396:dbl)
    n83 = Subtract(x=w407, y=w399) -> (x-y=w397:dbl)
    n84 = feedback #1(0.0) -> (w300:dbl)
    n85 = Multiply(x="Downsamp\nfact", y=w125) -> (x*y=w126:dbl)
    n86 = Multiply(x=w380, y="AY alpha") -> (x*y=w314:dbl)
    n87 = Multiply(x=w381, y="AX alpha") -> (x*y=w312:dbl)
    n88 = Multiply(x=w382, y="BX alpha") -> (x*y=w313:dbl)
    n89 = Multiply(x=w379, y="BY alpha") -> (x*y=w315:dbl)
    n90 = Add(x=w121, y=w300) -> (x+y=w298:dbl)
    n91 = feedback-in #1(w298) -> ()
    n92 = Square(x=w314) -> (x^2=w390:dbl)
    n93 = Square(x=w312) -> (x^2=w391:dbl)
    n94 = Square(x=w315) -> (x^2=w392:dbl)
    n95 = Square(x=w313) -> (x^2=w393:dbl)
    n96 = Bundle(w396, w397) -> (w115:cluster{dbl, dbl})  [unwired: 1 in]
    n97 = case shown="True" "Set reading to\nsetpoint" {
      tunnel: w115 -> [_ w454]
      frame False {
      }
      frame True {
        n98 = local write "Set reading to\nsetpoint"(FALSE ("Set reading to\nsetpoint")) -> ()
        n99 = local read "Trap position"() -> (w453:cluster{"X":dbl, "Y":dbl})
        n100 = property on="Setpoint voltage" class="Clust (strict)"("Val(Sgnl)"=w454) -> ()  [unwired: 2 in, 2 out]
        n101 = Unbundle(w453) -> ("X"=w452:dbl, "Y"=w451:dbl)
        n102 = Bundle("Y"=w451, "X"=w452) -> (w450:cluster{"Y":dbl, "X":dbl})  [unwired: 1 in]
        n103 = property on="Offset" class="Clust (strict)"("Val(Sgnl)"=w450) -> ()  [unwired: 2 in, 2 out]
      }
    }
    n104 = Reciprocal(x=w126) -> (1/x=→"Chart Freq (Hz)":dbl)
    n105 = To Time Stamp(1:w298) -> (0:w297:timestamp)
    n106 = Add(x=w390, y=w391) -> (x+y=w394:dbl)
    n107 = Add(x=w392, y=w393) -> (x+y=w405:dbl)
    n108 = Multiply(x=w312, y="AX kappa") -> (x*y=w308:dbl)
    n109 = Bundle("A y", "A x", "B y", "B x", "A sum", "B sum", "Trap x", "Trap y") -> (w288:T11)  [unwired: 1 in]
    n110 = Multiply(x=w313, y="BX kappa") -> (x*y=w309:dbl)
    n111 = Square Root(x=w394) -> (sqrt(x)=w410:dbl)
    n112 = Square Root(x=w405) -> (sqrt(x)=w409:dbl)
    n113 = Multiply(x=w314, y="AY kappa") -> (x*y=w310:dbl)
    n114 = Multiply(x=w315, y="BY kappa") -> (x*y=w311:dbl)
    n115 = Subtract(x=w360, y="Fixed Y") -> (x-y=w395:dbl)
    n116 = Subtract(x=w361, y="Fixed X") -> (x-y=w400:dbl)
    n117 = Cluster To Array(cluster=w288) -> (array=w287:string[])
    n118 = for {
      tunnel: w146 -> [w442] mode=indexing
      tunnel: w126 -> [w441]
      tunnel: "Downsamp\nfact" -> [w447]
      tunnel: [w445] -> w203 mode=indexing
      tunnel: w297 -> [w449]
      tunnel: w287 -> [w444] mode=indexing
      tunnel: "NI_ChannelName" ("name") -> [w443]
      n119 = call "Downsample 1D array.vi"("Ave N"=w447, "Arrray In"=w442) -> ("Array Out"=w448:dbl[])  [unwired: 9 in]
      n120 = Bundle By Name("Y"=w448, "dt"=w441, "t0"=w449) -> (w446:waveform(dbl))  [unwired: 1 in]
      n121 = Set Waveform Attribute(5:w444, 6:w443, 7:w446) -> (3:w445:waveform(dbl))  [unwired: 1 in, 2 out]
    }
    "All signals" <- w203
    n122 = Square(x=w310) -> (x^2=w383:dbl)
    n123 = Square(x=w308) -> (x^2=w384:dbl)
    n124 = Square(x=w311) -> (x^2=w385:dbl)
    n125 = Square(x=w309) -> (x^2=w386:dbl)
    n126 = Add(x=w383, y=w384) -> (x+y=w387:dbl)
    n127 = Add(x=w385, y=w386) -> (x+y=w388:dbl)
    n128 = Multiply(x=w395, y="Conv Y (nm/V)") -> (x*y=w317:dbl)
    n129 = Multiply(x=w400, y="Conv X (nm/V)") -> (x*y=w318:dbl)
    n130 = feedback #2() -> (w355:cluster{"B_Y":dbl, "B_X":dbl})  [unwired: 1 in]
    n131 = case shown="True" "Force Feedback" {
      tunnel: [w724 w740] -> w414
      tunnel: [w723 w739] -> w422
      tunnel: w115 -> [_ w738]
      tunnel: [cluster{"B_Y":dbl, "B_X":dbl} {"B_Y"=0.0, "B_X"=0.0} ("Sum error past") w730] -> w356
      tunnel: w355 -> [_ w737]
      tunnel: w415 -> [w724 w733]
      tunnel: w420 -> [w723 w732]
      frame False {
        # "Force feedback"
      }
      frame True {
        n132 = call "ForceFeedback2.vi"("PSD/Mirror Voltages"=w738, "Sum error"=w737, "task/channels in"=w733, "error in"=w732, "Desired voltage"="Setpoint voltage", "Feedback const"="Feedback const", "offset"="Offset") -> ("task out"=w740:refnum<k21>, "Sum error past"=w730:cluster{"B_Y":dbl, "B_X":dbl}, "Output Voltage"=→"Feedback Output Voltage 2":cluster{dbl, dbl}, "error out"=w739:errorcluster)  [unwired: 8 in, 1 out]
        n133 = local read "Pulling direction"() -> (w729:bool)
        n134 = Unbundle(w730) -> ("B_Y"=w727:dbl, "B_X"=w726:dbl)
        n135 = Select(t=w727, s=w729, f=w726) -> (s? t:f=→"Sum error":dbl)
      }
    }
    n136 = feedback-in #2(w356) -> ()
    n137 = Square Root(x=w387) -> (sqrt(x)=w316:dbl)
    n138 = Square Root(x=w388) -> (sqrt(x)=w411:dbl)
    n139 = Add(x=w316, y=w411) -> (x+y=w389:dbl)
    n140 = Build Array(w398, w399, w406, w407, w364, w363, w316, w411, w410, w409, w318, w317) -> ()  [unwired: 1 out]
    n141 = Divide(x=w389, y=2.0) -> (x/y=w353:dbl)
    n142 = Index Array(array=w203, index=6) -> (element=w151:waveform(dbl))
    n143 = Index Array(array=w203, index=7) -> (element=w153:waveform(dbl))
    n144 = local read "Fixed X"() -> (w207:dbl)
    n145 = local read "Fixed Y"() -> (w209:dbl)
    n146 = Unbundle By Name(w151) -> ("Y"=w211:dbl[])
    n147 = Unbundle By Name(w153) -> ("Y"=w210:dbl[])
    n148 = Index Array(array=w203, index=0) -> (element=w159:waveform(dbl))
    n149 = Index Array(array=w203, index=1) -> (element=w284:waveform(dbl))
    n150 = Index Array(array=w203, index=4) -> (element=w278:waveform(dbl))
    n151 = Subtract(x=w211, y=w207) -> (x-y=w208:dbl[])
    n152 = Subtract(x=w210, y=w209) -> (x-y=w205:dbl[])
    n153 = Unbundle By Name(w159) -> ("Y"=w276:dbl[])
    n154 = Unbundle By Name(w284) -> ("Y"=w275:dbl[])
    n155 = Unbundle By Name(w278) -> ("Y"=w274:dbl[])
    n156 = Index Array(array=w203, index=5) -> (element=w277:waveform(dbl))
    n157 = local read "Conv X (nm/V)"() -> (w206:dbl)
    n158 = local read "Conv Y (nm/V)"() -> (w204:dbl)
    n159 = Index Array(array=w203, index=2) -> (element=w156:waveform(dbl))
    n160 = Index Array(array=w203, index=3) -> (element=w281:waveform(dbl))
    n161 = Set Waveform Attribute(5:"T2 X", 6:w149, 7:w151) -> (3:w150:waveform(dbl))  [unwired: 1 in, 2 out]
    n162 = Set Waveform Attribute(5:"T2 Y", 6:w149, 7:w153) -> (3:w152:waveform(dbl))  [unwired: 1 in, 2 out]
    n163 = Unbundle By Name(w277) -> ("Y"=w271:dbl[])
    n164 = Unbundle By Name(w156) -> ("Y"=w273:dbl[])
    n165 = Unbundle By Name(w281) -> ("Y"=w272:dbl[])
    n166 = local read "Saving"() -> (w319:bool)
    n167 = local read "Tether"() -> (w320:bool)
    n168 = Divide(x=w276, y=w274) -> (x/y=w174:dbl[])
    n169 = Divide(x=w275, y=w274) -> (x/y=w172:dbl[])
    n170 = local read "AY offset"() -> (w262:dbl)
    n171 = local read "AX offset"() -> (w260:dbl)
    n172 = Multiply(x=w208, y=w206) -> (x*y=w143:dbl[])
    n173 = Multiply(x=w205, y=w204) -> (x*y=w145:dbl[])
    n174 = Less?(x=w353, y="Tether break\nforce (pN)") -> (x < y?=w351:bool)
    n175 = Divide(x=w272, y=w271) -> (x/y=w173:dbl[])
    n176 = Subtract(x=w172, y=w260) -> (x-y=w263:dbl[])
    n177 = local read "BY offset"() -> (w267:dbl)
    n178 = local read "BX offset"() -> (w270:dbl)
    n179 = Subtract(x=w174, y=w262) -> (x-y=w264:dbl[])
    n180 = Divide(x=w273, y=w271) -> (x/y=w175:dbl[])
    n181 = local read "AY alpha"() -> (w261:dbl)
    n182 = local read "AX alpha"() -> (w259:dbl)
    n183 = Compound Arithmetic op=AND(w319, w320, w351) -> (w350:bool)
    n184 = call-poly <vilib>:"Mean.vi"("X"=w145) -> ("mean"=w185:dbl)  [unwired: 1 out]
    "Mean Trp Pos Y 2 (nm)" <- w185
    n185 = Subtract(x=w175, y=w174) -> (x-y=w171:dbl[])
    n186 = Subtract(x=w173, y=w172) -> (x-y=w170:dbl[])
    n187 = Subtract(x=w143, y="Offset X (nm)") -> (x-y=w142:dbl[])
    n188 = Subtract(x=w145, y="Offset Y (nm)") -> (x-y=w144:dbl[])
    n189 = Subtract(x=w175, y=w267) -> (x-y=w269:dbl[])
    n190 = Subtract(x=w173, y=w270) -> (x-y=w268:dbl[])
    n191 = Subtract(x=w185, y=w145) -> (x-y=w184:dbl[])
    n192 = call-poly <vilib>:"Mean.vi"("X"=w143) -> ("mean"=w189:dbl)  [unwired: 1 out]
    "Mean Trap Pos X 2 (nm)" <- w189
    n193 = Build Array(w171, w170) -> (w168:dbl[][])
    n194 = Index Array(array=w168, index (row)=0) -> (element=w166:dbl[])  [unwired: 1 in]
    n195 = Index Array(array=w168, index (row)=1) -> (element=w165:dbl[])  [unwired: 1 in]
    n196 = call-poly <vilib>:"Mean.vi"("X"=w166) -> ("mean"=w164:dbl)  [unwired: 1 out]
    n197 = call-poly <vilib>:"Mean.vi"("X"=w165) -> ("mean"=w163:dbl)  [unwired: 1 out]
    n198 = Bundle("mean"=w164, "mean"=w163) -> ()  [unwired: 1 in, 1 out]
    n199 = local read "BY alpha"() -> (w266:dbl)
    n200 = local read "BX alpha"() -> (w265:dbl)
    n201 = Multiply(x=w264, y=w261) -> (x*y=w252:dbl[])
    n202 = Multiply(x=w263, y=w259) -> (x*y=w251:dbl[])
    n203 = Square(x=w184) -> (x^2=w183:dbl[])
    n204 = Subtract(x=w189, y=w143) -> (x-y=w188:dbl[])
    n205 = Bundle By Name(cluster=w152, "Y"=w144) -> (w201:waveform(dbl))
    n206 = case shown="True" w350 {
      selector: w350 -> [_ w468]
      frame False {
      }
      frame True {
        n207 = call <vilib>:"Beep.vi"() -> ()  [unwired: 12 in]
        n208 = Not(x=w468) -> (.not. x?=w466:bool)
        n209 = local write "Tether"(w466) -> ()
        n210 = local write "Force Feedback"(w466) -> ()
        n211 = property on="Stop saving" class="Bool (strict)"("Val(Sgnl)"="TA Cancel Save?") -> ()  [unwired: 2 in, 2 out]
      }
    }
    n212 = Bundle By Name(cluster=w150, "Y"=w142) -> (w202:waveform(dbl))
    n213 = Square(x=w188) -> (x^2=w187:dbl[])
    n214 = call-poly <vilib>:"Mean.vi"("X"=w183) -> ("mean"=w182:dbl)  [unwired: 1 out]
    n215 = Square(x=w252) -> (x^2=w258:dbl[])
    n216 = Multiply(x=w269, y=w266) -> (x*y=w250:dbl[])
    n217 = Square(x=w251) -> (x^2=w257:dbl[])
    n218 = Multiply(x=w268, y=w265) -> (x*y=w249:dbl[])
    n219 = call-poly <vilib>:"Mean.vi"("X"=w187) -> ("mean"=w186:dbl)  [unwired: 1 out]
    n220 = Build Array(w202, w201) -> (→"Trap sep":waveform(dbl)[])
    n221 = local read "Flushing Sample"() -> (w111:bool)
    n222 = Square Root(x=w182) -> (sqrt(x)=w181:dbl)
    n223 = Square(x=w250) -> (x^2=w256:dbl[])
    n224 = Square(x=w249) -> (x^2=w255:dbl[])
    n225 = Add(x=w258, y=w257) -> (x+y=w254:dbl[])
    n226 = Square Root(x=w186) -> (sqrt(x)=w179:dbl)
    n227 = Multiply(x=w181, y=10) -> (x*y=→"T2 Y RMS (A)":dbl)
    n228 = Square Root(x=w254) -> (sqrt(x)=w138:dbl[])
    n229 = Add(x=w256, y=w255) -> (x+y=w253:dbl[])
    n230 = Set Waveform Attribute(5:"T2", 6:"NI_ChannelName" ("name"), 7:w159) -> (3:w158:waveform(dbl))  [unwired: 1 in, 2 out]
    n231 = Set Waveform Attribute(5:"T1", 6:"NI_ChannelName" ("name"), 7:w156) -> (3:w155:waveform(dbl))  [unwired: 1 in, 2 out]
    n232 = Square Root(x=w253) -> (sqrt(x)=w137:dbl[])
    n233 = Multiply(x=w179, y=10) -> (x*y=→"T2 X RMS (A)":dbl)
    n234 = Bundle By Name(cluster=w158, "Y"=w138) -> (w162:waveform(dbl))
    n235 = case shown="True" w111 {
      frame False {
      }
      frame True {
        n236 = local read "Flush Sample Start Time"() -> (w433:u32)
        n237 = local read "Sample flush time (s)"() -> (w426:dbl)
        n238 = Tick Count (ms)() -> (millisecond timer value=w434:u32)
        n239 = Subtract(x=w434, y=w433) -> (x-y=w424:u32)
        n240 = Multiply(x=u32 1000, y=w426) -> (x*y=w425:dbl)
        n241 = Divide(x=w424, y=w425) -> (x/y=w429:dbl)
        n242 = Greater?(x=w424, y=w425) -> (0:w432:bool)
        n243 = Not(x=w432) -> (.not. x?=w431:bool)
        n244 = Boolean To (0,1)(Boolean=w431) -> (0, 1=w430:i16)
        n245 = Compound Arithmetic op=MULTIPLY(w430, w429, 100.0 ("value")) -> (→"Sample Flush Meter":dbl)
        n246 = case shown="True" w432 {
          frame False {
          }
          frame True {
            w436 = FALSE ("Inject Sample")
            n247 = property on="Clear Volume" class="Bool (strict)"("Val(Sgnl)"=TRUE ("Value (Signaling)")) -> ()  [unwired: 2 in, 2 out]
            n248 = local write "Inject Sample"(w436) -> ()
            n249 = local write "Flushing Sample"(w436) -> ()
          }
        }
      }
    }
    n250 = Bundle By Name(cluster=w155, "Y"=w137) -> (w231:waveform(dbl))
    n251 = Add(x=w138, y=w137) -> (x+y=w136:dbl[])
    n252 = case shown="True" "Remove offsets" {
      selector: "Remove offsets" -> [_ w439]
      frame False {
      }
      frame True {
        n253 = local read "Mean Trp Pos Y 2 (nm)"() -> (w437:dbl)
        n254 = Not(x=w439) -> (.not. x?=w440:bool)
        n255 = local read "Mean Trap Pos X 2 (nm)"() -> (w438:dbl)
        n256 = local write "Remove offsets"(w440) -> ()
        n257 = local write "Offset Y (nm)"(w437) -> ()
        n258 = local write "Offset X (nm)"(w438) -> ()
      }
    }
    n259 = Build Array(w162, w231) -> (→"Bead sep":waveform(dbl)[])
    n260 = local read "AY kappa"() -> (w248:dbl)
    n261 = local read "AX kappa"() -> (w247:dbl)
    n262 = Divide(x=w136, y=2) -> (x/y=w134:dbl[])
    n263 = local read "BX kappa"() -> (w245:dbl)
    n264 = local read "BY kappa"() -> (w246:dbl)
    n265 = call-poly <vilib>:"Mean.vi"("X"=w134) -> ("mean"=w133:dbl)  [unwired: 1 out]
    "Mean Bead Sep\n(nm)" <- w133
    n266 = local read "Calibrating"() -> (w412:bool)
    n267 = Multiply(x=w252, y=w248) -> (x*y=w241:dbl[])
    n268 = Multiply(x=w251, y=w247) -> (x*y=w242:dbl[])
    n269 = Square(x=w241) -> (x^2=w240:dbl[])
    n270 = Square(x=w242) -> (x^2=w239:dbl[])
    n271 = Subtract(x=w134, y=w133) -> (x-y=w132:dbl[])
    n272 = Multiply(x=w250, y=w246) -> (x*y=w243:dbl[])
    n273 = Multiply(x=w249, y=w245) -> (x*y=w244:dbl[])
    n274 = Add(x=w240, y=w239) -> (x+y=w236:dbl[])
    n275 = Square(x=w132) -> (x^2=w131:dbl[])
    n276 = Square Root(x=w236) -> (sqrt(x)=w199:dbl[])
    n277 = Square(x=w243) -> (x^2=w238:dbl[])
    n278 = Square(x=w244) -> (x^2=w237:dbl[])
    n279 = call-poly <vilib>:"Mean.vi"("X"=w131) -> ("mean"=w130:dbl)  [unwired: 1 out]
    n280 = Add(x=w238, y=w237) -> (x+y=w235:dbl[])
    n281 = Bundle By Name(cluster=w158, "Y"=w199) -> (w234:waveform(dbl))
    n282 = local read "Saving"() -> (w349:bool)
    n283 = Or(x=w412, y=w349) -> ()  [unwired: 1 out]
    n284 = Square Root(x=w130) -> (sqrt(x)=w129:dbl)
    n285 = Square Root(x=w235) -> (sqrt(x)=w198:dbl[])
    n286 = And(x="Save scans", y="Raster scan") -> (x .and. y?=w109:bool)
    n287 = Multiply(x=10, y=w129) -> (x*y=→"Bead Sep Noise\n(A)":dbl)
    n288 = Bundle By Name(cluster=w155, "Y"=w198) -> (w233:waveform(dbl))
    n289 = Add(x=w199, y=w198) -> (x+y=w197:dbl[])
    n290 = Build Array(w234, w233) -> (→"Force (pN)":waveform(dbl)[])
    n291 = flat-sequence {
      tunnel: w412 -> [w506]
      tunnel: w349 -> [_]
      tunnel: w412 -> [_]
      tunnel: w349 -> [_]
      tunnel: w146 -> [w490]
      tunnel: [w490] -> w370
      tunnel: w229 -> [w489]
      tunnel: [w489] -> w369
      tunnel: w357 -> [w488]
      tunnel: [w488] -> w362
      tunnel: w359 -> [w487]
      tunnel: [w487] -> w358
      tunnel: [w484] -> w348
      tunnel: [w481] -> w347
      tunnel: [w478] -> w216
      tunnel: [w477] -> w215
      tunnel: [w474] -> w214
      tunnel: w109 -> [w470]
      tunnel: w370 -> [w655]
      tunnel: w369 -> [w654]
      tunnel: w362 -> [_]
      tunnel: w358 -> [_]
      tunnel: w348 -> [w653]
      tunnel: w347 -> [w652]
      tunnel: w216 -> [w651]
      tunnel: w215 -> [w650]
      tunnel: w214 -> [w649]
      frame #0 {
        w501 = 0.0
        # "1: old trap\n0: fleezers"
        # "Create files if saving data"
        n292 = local read "Save N sets"() -> (w473:bool)
        n293 = local read "Sampling Rate"() -> (w504:dbl)
        n294 = Or(x=w473, y="Save Data") -> (x .or. y?=w471:bool)
        n295 = Build Array(w471, "Save cal", w470) -> (w492:bool[])
        n296 = Compound Arithmetic op=OR("Save Data", "Save cal", w470) -> (w494:bool)
        n297 = Boolean Array To Number(Boolean array=w492) -> (number=w491:u32)
        n298 = local read "Trap position"() -> (w500:cluster{"X":dbl, "Y":dbl})
        n299 = Unbundle(w500) -> ("X"=w498:dbl, "Y"=w499:dbl)
        n300 = Build Array(w501, w501, w499, w498, w501, w501) -> (w497:dbl[])
        n301 = feedback #3(refnum<k0> refnum) -> (w482:refnum<file>)
        n302 = feedback #4() -> (w479:dbl)  [unwired: 1 in]
        n303 = feedback #5(FALSE) -> (w475:bool)
        n304 = feedback #6(0) -> (w495:i32)
        n305 = feedback #7(refnum<k0> refnum) -> (w485:refnum<file>)
        n306 = case shown="True" w494 {
          tunnel: w506 -> [_ _]
          tunnel: 9 -> [_ w548]
          tunnel: w504 -> [_ w547]
          tunnel: 6 -> [_ w546]
          tunnel: 5 -> [_ w545]
          tunnel: w497 -> [_ w544]
          tunnel: [w511 1] -> w478
          tunnel: w495 -> [w512 _]
          tunnel: w491 -> [_ w519]
          tunnel: [w510 w517] -> w484
          tunnel: w485 -> [w510 _]
          tunnel: [w509 w516] -> w481
          tunnel: w482 -> [w509 _]
          tunnel: 1.0 -> [_ w515]
          tunnel: [w508 w514] -> w477
          tunnel: w479 -> [w508 _]
          tunnel: [w507 w513] -> w474
          tunnel: w475 -> [w507 _]
          frame False {
            n307 = Increment(x=w512) -> (x+1=w511:i32)
          }
          frame True {
            w520 = FALSE ("Save Data")
            w526 = FALSE
            w527 = T10."big-endian, network order" ("byte order (0:big-endian, network order)")
            n308 = local write "Save cal"(w520) -> ()
            n309 = local write "Save Data"(w520) -> ()
            n310 = case shown="4" w519 {
              tunnel: w548 -> [w594 w612 w647]
              tunnel: w547 -> [w593 w611 w646]
              tunnel: w546 -> [w592 w609 w642]
              tunnel: w545 -> [w591 w608 w641]
              tunnel: w544 -> [w589 w605 w638]
              tunnel: [w588 w604 w624] -> w541
              tunnel: [w590 w601 w623] -> w513
              tunnel: ["Averaging Number" 200 w621] -> _
              tunnel: w515 -> [w576 w596 w620]
              tunnel: [w572 "Cal sets to save" w615] -> w514
              frame 1, Default {
                w590 = TRUE
                w577 = 0.0
                # "Time trace"
                n311 = local read "Averaging Number"() -> (w587:i32)
                n312 = Boolean To (0,1)(Boolean=w590) -> (0, 1=w582:i16)
                n313 = Increment(x=w582) -> (x+1=w581:i16)
                n314 = Divide(x=w593, y=w587) -> (x/y=w586:dbl)
                n315 = To Double Precision Float(number=w581) -> (double precision float=w580:dbl)
                n316 = Reciprocal(x=w586) -> (1/x=w585:dbl)
                n317 = Build Array(w594, w593, w585, w592, w591, 0 ("f")) -> (w584:dbl[])
                n318 = Build Array(w580, w576, w577, w577, w577) -> (w583:dbl[])
                n319 = Build Array (concatenate)(w584, w589, w583) -> (w588:dbl[])
                n320 = Select(t="N sets", s="Save N sets", f=2147483647) -> (s? t:f=w572:i32)
              }
              frame 2 {
                w601 = FALSE
                w599 = 0.0
                # "Calibration file"
                n321 = Reciprocal(x=w611) -> (1/x=w610:dbl)
                n322 = Boolean To (0,1)(Boolean=w601) -> (0, 1=w603:i16)
                n323 = To Double Precision Float(number=w603) -> (double precision float=w602:dbl)
                n324 = Build Array(w612, w610, w610, w609, w608, 1) -> (w606:dbl[])
                n325 = Build Array(w602, w596, w599, w599, w599) -> (w600:dbl[])
                n326 = Build Array (concatenate)(w606, w605, w600) -> (w604:dbl[])
                "Calibrating" <- TRUE ("Calibrating")
              }
              frame 4 {
                w622 = 0
                w634 = 0.0
                w623 = TRUE
                # "Not using nsteps yet"
                # "FX curve"
                n327 = local read "Averaging Number"() -> (w645:i32)
                n328 = Boolean To (0,1)(Boolean=w623) -> (0, 1=w637:i16)
                n329 = Increment(x=w637) -> (x+1=w636:i16)
                n330 = local write "Raster scan"(FALSE ("Raster scan")) -> ()
                n331 = To Double Precision Float(number=w636) -> (double precision float=w635:dbl)
                n332 = Divide(x=w646, y=w645) -> (x/y=w644:dbl)
                n333 = Reciprocal(x=w644) -> (1/x=w643:dbl)
                n334 = Build Array(w635, w620, w634, w634, w634) -> (w633:dbl[])
                n335 = Build Array(w647, w646, w643, w642, w641, 2) -> (w639:dbl[])
                n336 = local read "Data update period (s/set)"() -> (w618:dbl)
                n337 = local read "Pulling direction"() -> (w631:bool)
                n338 = local read "Max delta"() -> (w629:dbl)
                n339 = local read "Min delta"() -> (w628:dbl)
                n340 = local read "# scans"() -> (w626:i32)
                n341 = local read "Speed (ms)"() -> (w619:i32)
                n342 = Subtract(x=w629, y=w628) -> (x-y=w627:dbl)
                n343 = Not(x=w631) -> (.not. x?=w630:bool)
                n344 = local read "Averaging Number"() -> (w621:i32)
                n345 = Boolean To (0,1)(Boolean=w630) -> (0, 1=w632:i16)
                n346 = Multiply(x=750.0, y=w618) -> (x*y=w616:dbl)
                n347 = Build Array(w632, w627, w622, w622, w626) -> (w625:dbl[])
                n348 = Divide(x=w619, y=w616) -> (x/y=w614:dbl)
                n349 = Build Array (concatenate)(w639, w638, w633, w625) -> (w624:dbl[])
                n350 = Round Toward +Infinity(x=w614) -> (ceil(x): smallest int >= x=w615:dbl)
              }
            }
            n351 = call "CreateSaveFile.vi"("Index In"="Save file index", "Ext"=".dat", "Insert"="", "Directory"="Path") -> ("Path Out"=w525:path)  [unwired: 6 in, 1 out]
            "Current file name" <- w525
            n352 = Open/Create/Replace File(file path (use dialog)=w525, operation (0:open)=T9."create", access (0:read/write)=enum16{"read/write", "read-only", "write-only"}."write-only") -> (refnum out=w534:refnum<file>, error out=w535:errorcluster)  [unwired: 3 in, 1 out]
            n353 = Array Size(array=w541) -> (size(s)=w543:i32)
            n354 = case shown="True" w513 {
              tunnel: w525 -> [_ w571]
              tunnel: [refnum<k0> refnum w550] -> w516
              frame False {
              }
              frame True {
                w557 = 0.0
                n355 = Path To String(path=w571) -> (string=w567:string)
                n356 = Build Array(w557, w557, w557, w557, w557, w557, w557, w557) -> (w554:dbl[])
                n357 = String Length(string=w567) -> (length=w570:i32)
                n358 = Array Size(array=w554) -> (size(s)=w556:i32)
                n359 = Subtract(x=w570, y=4) -> (x-y=w568:i32)
                n360 = To Double Precision Float(number=w556) -> (double precision float=w555:dbl)
                n361 = String Subset(string=w567, length (rest)=w568) -> (substring=w566:string)  [unwired: 1 in]
                n362 = Build Array (concatenate)(w555, w554) -> (w553:dbl[])
                n363 = Concatenate Strings(w566, "_pos.dat" ("string")) -> (w564:string)
                n364 = String To Path(string=w564) -> (path=w563:path)
                n365 = Open/Create/Replace File(file path (use dialog)=w563, operation (0:open)=T9."create", access (0:read/write)=enum16{"read/write", "read-only", "write-only"}."write-only") -> (refnum out=w559:refnum<file>, error out=w560:errorcluster)  [unwired: 3 in, 1 out]
                n366 = Deny Access(4:w560, 7:w559) -> (3:w558:refnum<file>)  [unwired: 1 in, 1 out]
                n367 = Write to Binary File(file (use dialog)=w558, data=w553, 5:FALSE ("prepend array or string size? (T)"), 9:T10."big-endian, network order" ("byte order (0:big-endian, network order)")) -> (refnum out=w550:refnum<file>)  [unwired: 2 in, 2 out]
              }
            }
            n368 = Deny Access(4:w535, 7:w534) -> (0:w524:errorcluster, 3:w533:refnum<file>)  [unwired: 1 in]
            n369 = String Length(string="Comment") -> (length=w540:i32)
            n370 = To Double Precision Float(number=w543) -> (double precision float=w542:dbl)
            n371 = To Double Precision Float(number=w540) -> (double precision float=w539:dbl)
            n372 = Build Array (concatenate)(w542, w541, w539) -> (w530:dbl[])
            n373 = Write to Binary File(file (use dialog)=w533, data=w530, error in=w524, 5:w526, 9:w527) -> (refnum out=w529:refnum<file>, error out=w523:errorcluster)  [unwired: 1 in, 1 out]
            n374 = Write to Binary File(file (use dialog)=w529, data="Comment", error in=w523, 5:w526, 9:w527) -> (refnum out=w517:refnum<file>)  [unwired: 1 in, 2 out]
            "Saving" <- TRUE
          }
        }
        n375 = feedback-in #3(w481) -> ()
        n376 = feedback-in #4(w477) -> ()
        n377 = feedback-in #5(w474) -> ()
        n378 = feedback-in #6(w478) -> ()
        n379 = feedback-in #7(w484) -> ()
      }
      frame #1 {
        n380 = local read "Saving"() -> (w648:bool)
        n381 = case shown="True" w648 {
          tunnel: w655 -> [_ w672]
          tunnel: w654 -> [_ w671]
          tunnel: w653 -> [_ w670]
          tunnel: w652 -> [_ w669]
          tunnel: w651 -> [_ w659]
          tunnel: w650 -> [_ w660]
          tunnel: w649 -> [_ w663]
          frame False {
            (unwired) FALSE ("Calibrating")
          }
          frame True {
            n382 = local read "Stop"() -> (w667:bool)
            n383 = Less Or Equal?(x=w659, y=w660) -> (x <= y?=w668:bool)
            n384 = Divide(x=w659, y=w660) -> (x/y=w658:dbl)
            n385 = Or(x=w667, y="Stop saving") -> (x .or. y?=w666:bool)
            n386 = Not(x=w666) -> (.not. x?=w665:bool)
            n387 = Multiply(x=100.0, y=w658) -> (x*y=w657:dbl)
            n388 = And(x=w668, y=w665) -> (x .and. y?=w664:bool)
            n389 = case shown="True" w664 {
              tunnel: w670 -> [w677 w684]
              tunnel: w671 -> [_ w683]
              tunnel: w672 -> [_ w682]
              tunnel: w669 -> [w676 w681]
              tunnel: w663 -> [w674 _]
              tunnel: [0.0 ("Progress") w680] -> w662
              tunnel: w657 -> [_ w680]
              frame False {
                w675 = FALSE
                n390 = Close File(refnum=w677) -> ()  [unwired: 1 in, 2 out]
                n391 = case shown="True" w674 {
                  tunnel: w676 -> [_ w678]
                  frame False {
                  }
                  frame True {
                    n392 = Close File(refnum=w678) -> ()  [unwired: 1 in, 2 out]
                  }
                }
                n393 = call <vilib>:"Beep.vi"() -> ()  [unwired: 12 in]
                n394 = local write "Saving"(w675) -> ()
                n395 = local write "Stop saving"(w675) -> ()
                n396 = local write "Calibrating"(w675) -> ()
              }
              frame True {
                n397 = local read "Calibrating"() -> (w679:bool)
                n398 = case shown="False" w679 {
                  tunnel: w684 -> [w706 w722]
                  tunnel: w683 -> [_ w721]
                  tunnel: w682 -> [w693 w715]
                  tunnel: w681 -> [w692 _]
                  frame False {
                    n399 = local read "Averaging Number"() -> (w700:i32)
                    n400 = Array Subset(array=w693, index (row)=0 ("index"), length (row)=6 ("length")) -> (w689:dbl[][])  [unwired: 2 in]
                    n401 = Array Subset(array=w693, index (row)=6 ("index"), length (row)=2 ("length")) -> (w688:dbl[][])  [unwired: 2 in]
                    n402 = Array Size(array=w688) -> (size(s)=w699:i32[])
                    n403 = Array Size(array=w689) -> (size(s)=w696:i32[])
                    n404 = for {
                      tunnel: w689 -> [w710] mode=indexing
                      tunnel: w700 -> [w712]
                      tunnel: [w711] -> w687 mode=indexing
                      n405 = call "Downsample 1D array.vi"("Ave N"=w712, "Arrray In"=w710) -> ("Array Out"=w711:dbl[])  [unwired: 9 in]
                    }
                    n406 = Multiply Array Elements(1:w696) -> (0:w695:i32)
                    n407 = for {
                      tunnel: w688 -> [w709] mode=indexing
                      tunnel: w700 -> [w708]
                      tunnel: [w707] -> w691 mode=indexing
                      n408 = call "Downsample 1D array.vi"("Ave N"=w708, "Arrray In"=w709) -> ("Array Out"=w707:dbl[])  [unwired: 9 in]
                    }
                    n409 = Multiply Array Elements(1:w699) -> (0:w698:i32)
                    n410 = Divide(x=w695, y=w700) -> (x/y=w701:dbl)
                    n411 = Divide(x=w698, y=w700) -> (x/y=w697:dbl)
                    n412 = Transpose 2D Array(2D array=w687) -> (transposed array=w686:dbl[][])
                    n413 = Transpose 2D Array(2D array=w691) -> (transposed array=w685:dbl[][])
                    "Waveform Chart 3" <- w685
                    n414 = Reshape Array(w686, w701) -> (w690:dbl[])
                    n415 = Reshape Array(w685, w697) -> (w694:dbl[])
                    n416 = call <vilib>:"Write File+ [SGL].vi"("1D array"=w694, "refnum"=w692) -> ()  [unwired: 7 in, 3 out]
                    n417 = call <vilib>:"Write File+ [SGL].vi"("1D array"=w690, "refnum"=w706) -> ()  [unwired: 7 in, 3 out]
                  }
                  frame True {
                    n418 = Array Subset(array=w715, index (row)=0 ("index"), length (row)=6 ("length")) -> (w713:dbl[][])  [unwired: 2 in]
                    n419 = Transpose 2D Array(2D array=w713) -> (transposed array=w719:dbl[][])
                    n420 = Array Size(array=w713) -> (size(s)=w714:i32[])
                    n421 = Multiply Array Elements(1:w714) -> (0:w720:i32)
                    n422 = Reshape Array(w719, w720) -> (w718:dbl[])
                    n423 = call <vilib>:"Write File+ [SGL].vi"("1D array"=w718, "error in (no error)"=w721, "refnum"=w722) -> ()  [unwired: 6 in, 3 out]
                  }
                }
              }
            }
            "Progress" <- w662
          }
        }
      }
    }
    n424 = Divide(x=w197, y=2) -> (x/y=w194:dbl[])
    n425 = call-poly <vilib>:"Mean.vi"("X"=w194) -> ("mean"=w195:dbl)  [unwired: 1 out]
    "Mean force (pN)" <- w195
    n426 = Subtract(x=w195, y=w194) -> (x-y=w193:dbl[])
    n427 = Square(x=w193) -> (x^2=w192:dbl[])
    n428 = call-poly <vilib>:"Mean.vi"("X"=w192) -> ("mean"=w191:dbl)  [unwired: 1 out]
    n429 = Square Root(x=w191) -> (sqrt(x)=→"Force noise (pN)":dbl)
    n430 = local read "Stop"() -> (w419:bool)
  }
  n431 = local write "Progress"(u8 0 ("Progress")) -> ()
  n432 = local write "Calibrating"(FALSE ("Calibrating")) -> ()
  n433 = call "InitializeChamberImage.vi"() -> ("error out"=w101:errorcluster, "IMAQ Session Out"=w102:refnum<k11>, "Display Out"=w103:T7, "Acquired Image"=w9:T7)  [unwired: 8 in]
  n434 = node-c288(i64 10 ("Period"), 2 ("Processor")) -> (w15:T12)  [unwired: 2 in]
  n435 = timed-loop {
    tunnel: w103 -> [w750]
    tunnel: w102 -> [w749]
    tunnel: w101 -> [w748]
    tunnel: [w746] -> w100
    tunnel: [w745] -> w99
    timing: w15 -> [_]
    timing-out: [_] -> w14
    i -> [w747]
    stop <- w741 continue-if-true
    n436 = node-c288() -> ()  [unwired: 1 in, 1 out]
    n437 = call <vilib>:"IMAQ Copy Acquired Buffer.vi"("IMAQ Session In"=w749, "Image In"=w750, "Buffer Number"=w747, "error in (no error)"=w748) -> ("IMAQ Session Out"=w746:refnum<k11>, "Image Out"=→"Chamber":T7, "error out"=w745:errorcluster)  [unwired: 7 in, 2 out]
    "Video Error" <- w745
    n438 = local read "Stop"() -> (w743:bool)
    n439 = Unbundle By Name(w745) -> ("status"=w744:bool)
    n440 = Not Or(1:w743, 2:w744) -> (0:w741:bool)
    "Continue to display?" <- w741
    n441 = node-c288() -> ()  [unwired: 1 in, 1 out]
  }
  n442 = node-c288(w14) -> ()  [unwired: 1 out]
  n443 = call <vilib>:"IMAQ Close.vi"("error in (no error)"=w99, "IMAQ Session In"=w100) -> ("error out"=w107:errorcluster)  [unwired: 9 in]
  n444 = call "IMAQ Dispose"("error in (no error)"=w107) -> ("error out"=w106:errorcluster)  [unwired: 5 in]
  n445 = call-poly "VISA Configure Serial Port"("VISA resource name"=refnum<visa-resource-name> "COM3") -> ("VISA resource name out"=w21:refnum<visa-resource-name>, "error out"=w20:errorcluster)  [unwired: 13 in]
  n446 = node-c288(i64 100 ("Period"), 2 ("Processor")) -> (w23:T12)  [unwired: 2 in]
  n447 = call "IMAQ Dispose"("Image"=w9, "error in (no error)"=w106) -> ("error out"=w105:errorcluster)  [unwired: 4 in]
  n448 = timed-loop {
    timing: w23 -> [_]
    timing-out: [_] -> w22
    tunnel: w21 -> [w753]
    tunnel: w20 -> [w755]
    tunnel: [w753] -> w19
    stop <- w754 stop-if-true
    n449 = node-c288() -> ()  [unwired: 1 in, 1 out]
    n450 = event shown="[7] \"Force FB script\": Value Change" {
      selector: _ -> [_ _ _ _ _ _ _ _ _ _ _]
      dyn-events: _ -> [_ _ _ _ _ _ _ _ _ _ _]
      timeout: _ -> [_ _ _ _ _ _ _ _ _ _ _]
      tunnel: w753 -> [w762 w798 w816 w830 w844 w863 w883 _ _ _ _]
      tunnel: w755 -> [w761 w797 w815 w829 w843 w862 w882 _ _ _ _]
      tunnel: [_ _ _ _ _ _ _ _ _ _ w934] -> w754
      event "Got DNA bead": Value Change {
        n451 = event-data() -> ()  [unwired: 1 in, 5 out]
        n452 = flat-sequence {
          tunnel: w762 -> [w765]
          tunnel: w761 -> [w763]
          tunnel: [w779] -> w760
          tunnel: w760 -> [w782]
          tunnel: [w782] -> w759
          tunnel: w759 -> [w784]
          tunnel: [w784] -> w758
          tunnel: w758 -> [w788]
          tunnel: [w788] -> w757
          tunnel: w757 -> [w790]
          tunnel: [w790] -> w756
          tunnel: w756 -> [w792]
          frame #0 {
            n453 = local read "Saved stage positions"() -> (w766:dbl[][])
            n454 = disable-structure shown="Disabled" {
              frame Disabled {
                n455 = property on="Inject Pump 2" class="Bool (strict)"("Val(Sgnl)"=FALSE ("Inject Pump 2")) -> ()  [unwired: 2 in, 2 out]
              }
              frame Enabled {
              }
            }
            n456 = local write "Stage moving"(TRUE ("Stage moving")) -> ()
            n457 = property on="Trap delta" class="DigNum (strict)"("Val(Sgnl)"="Cal @ Delta (V)") -> ()  [unwired: 2 in, 2 out]
            n458 = call "move to saved stage position.vi"("error in"=w763, "Stage VISA resource name in"=w765, "Position"="Cal stage position", "Saved Stage Positions"=w766) -> ()  [unwired: 2 out]
          }
          frame #1 {
            n459 = local write "Stage moving"(FALSE ("Stage moving")) -> ()
            n460 = property on="Inject Sample" class="Bool (strict)"("Val(Sgnl)"=FALSE ("Value (Signaling)")) -> ()  [unwired: 2 in, 2 out]
            n461 = call <vilib>:"Beep.vi"() -> ()  [unwired: 12 in]
          }
          frame #2 {
            n462 = Wait (ms)(milliseconds to wait=u32 1000) -> ()  [unwired: 1 out]
          }
          frame #3 {
            n463 = property on="Save cal" class="Bool (strict)"("Val(Sgnl)"=TRUE ("Value (Signaling)")) -> ()  [unwired: 2 in, 2 out]
          }
          frame #4 {
            n464 = Wait (ms)(milliseconds to wait=u32 2000) -> ()  [unwired: 1 out]
          }
          frame #5 {
            n465 = while {
              stop <- w776 stop-if-true
              n466 = local read "Saving"() -> (w777:bool)
              n467 = Not(x=w777) -> (.not. x?=w776:bool)
              n468 = Wait (ms)(milliseconds to wait=u32 100) -> ()  [unwired: 1 out]
            }
          }
          frame #6 {
            n469 = Wait (ms)(milliseconds to wait=u32 2000) -> ()  [unwired: 1 out]
          }
          frame #7 {
            # "Only continue if there is no buffer\noverflow error"
            n470 = local read "Buffer Overflow"() -> (w780:bool)
            n471 = Not(x=w780) -> (.not. x?=w779:bool)
            n472 = case shown="True" w779 {
              frame False {
              }
              frame True {
                n473 = property on="Raster scan" class="Bool (strict)"("Val(Sgnl)"=TRUE ("Value (Signaling)")) -> ()  [unwired: 2 in, 2 out]
              }
            }
          }
          frame #8 {
            n474 = case shown="True" w782 {
              frame False {
              }
              frame True {
                n475 = Wait (ms)(milliseconds to wait=u32 2000) -> ()  [unwired: 1 out]
              }
            }
          }
          frame #9 {
            n476 = case shown="True" w784 {
              frame False {
              }
              frame True {
                n477 = while {
                  stop <- w786 stop-if-true
                  n478 = local read "Saving"() -> (w787:bool)
                  n479 = Not(x=w787) -> (.not. x?=w786:bool)
                  n480 = Wait (ms)(milliseconds to wait=u32 100) -> ()  [unwired: 1 out]
                }
              }
            }
          }
          frame #10 {
            n481 = case shown="True" w788 {
              frame False {
              }
              frame True {
                n482 = property on="Read Cal" class="Bool (strict)"("Val(Sgnl)"=TRUE ("Value (Signaling)")) -> ()  [unwired: 2 in, 2 out]
              }
            }
          }
          frame #11 {
            n483 = case shown="True" w790 {
              frame False {
              }
              frame True {
                n484 = Wait (ms)(milliseconds to wait=u32 1000) -> ()  [unwired: 1 out]
              }
            }
          }
          frame #12 {
            n485 = case shown="True" w792 {
              frame False {
              }
              frame True {
                n486 = property on="Inject Sample" class="Bool (strict)"("Val(Sgnl)"=TRUE ("Value (Signaling)")) -> ()  [unwired: 2 in, 2 out]
                n487 = property on="Fish" class="Bool (strict)"("Val(Sgnl)"=TRUE ("Value (Signaling)")) -> ()  [unwired: 2 in, 2 out]
              }
            }
          }
        }
      }
      event "Dump beads": Value Change {
        n488 = event-data() -> ()  [unwired: 1 in, 5 out]
        n489 = flat-sequence {
          tunnel: w797 -> [w801]
          tunnel: w798 -> [w802]
          tunnel: [w802] -> w796
          tunnel: [w801] -> w795
          tunnel: w796 -> [w804]
          tunnel: w795 -> [w803]
          frame #0 {
            w800 = FALSE ("Fish")
            n490 = local read "Saving"() -> (w799:bool)
            n491 = local write "Force Feedback"(w800) -> ()
            n492 = local write "Dump beads"(w800) -> ()
            n493 = property on="Stop saving" class="Bool (strict)"("Val(Sgnl)"=w799) -> ()  [unwired: 2 in, 2 out]
            n494 = local write "Fish"(w800) -> ()
          }
          frame #1 {
            n495 = local read "Saved stage positions"() -> (w806:dbl[][])
            n496 = local write "Stage moving"(TRUE ("Stage moving")) -> ()
            n497 = call "move to saved stage position.vi"("error in"=w803, "Stage VISA resource name in"=w804, "Position"=5, "Saved Stage Positions"=w806) -> ()  [unwired: 2 out]
          }
          frame #2 {
            n498 = local read "Shutter 1 (B)"() -> (w810:bool)
            n499 = local read "Shutter 2 (A)"() -> (w809:bool)
            n500 = call <vilib>:"Beep.vi"() -> ()  [unwired: 12 in]
            n501 = case shown="True" w810 {
              frame False {
              }
              frame True {
                n502 = property on="Shutter 1 (B)" class="Bool (strict)"("Val(Sgnl)"=FALSE ("Value (Signaling)")) -> ()  [unwired: 2 in, 2 out]
              }
            }
            n503 = case shown="True" w809 {
              frame False {
              }
              frame True {
                n504 = property on="Shutter 2 (A)" class="Bool (strict)"("Val(Sgnl)"=FALSE) -> ()  [unwired: 2 in, 2 out]
              }
            }
            n505 = local write "Stage moving"(FALSE ("Stage moving")) -> ()
            n506 = local write "Tether"(FALSE ("Tether")) -> ()
          }
          frame #3 {
            n507 = property on="Move Cap. 2 (ADig Top)" class="Bool (strict)"("Val(Sgnl)"=TRUE ("Value (Signaling)")) -> ()  [unwired: 2 in, 2 out]
          }
        }
      }
      event "Move Cap. 2 (ADig Top)": Value Change {
        n508 = event-data() -> ()  [unwired: 1 in, 5 out]
        n509 = flat-sequence {
          tunnel: w816 -> [w818]
          tunnel: w815 -> [w817]
          frame #0 {
            n510 = local read "Saved stage positions"() -> (w820:dbl[][])
            n511 = local write "Move Cap. 2 (ADig Top)"(FALSE ("Move Cap. 2 (ADig Top)")) -> ()
            n512 = local write "Stage moving"(TRUE ("Stage moving")) -> ()
            n513 = call "move to saved stage position.vi"("error in"=w817, "Stage VISA resource name in"=w818, "Position"=2, "Saved Stage Positions"=w820) -> ()  [unwired: 2 out]
          }
          frame #1 {
            # "Make sure you don't reverse\nwhich is ON and OFF"
            n514 = local read "Cal @ Delta (V)"() -> (w824:dbl)
            n515 = local write "Stage moving"(FALSE ("Stage moving")) -> ()
            n516 = call <vilib>:"Beep.vi"() -> ()  [unwired: 12 in]
            n517 = property on="Trap delta" class="DigNum (strict)"("Val(Sgnl)"=w824) -> ()  [unwired: 2 in, 2 out]
            n518 = disable-structure shown="Disabled" {
              frame Disabled {
                n519 = property on="Inject Pump 1" class="Bool (strict)"("Val(Sgnl)"=TRUE ("Inject Pump 2")) -> ()  [unwired: 2 in, 2 out]
              }
              frame Enabled {
              }
            }
            n520 = local read "Shutter 2 (A)"() -> (w823:bool)
            n521 = case shown="False" w823 {
              frame False {
                n522 = property on="Shutter 2 (A)" class="Bool (strict)"("Val(Sgnl)"=TRUE ("Value (Signaling)")) -> ()  [unwired: 2 in, 2 out]
              }
              frame True {
              }
            }
          }
        }
      }
      event "Got ADig bead": Value Change {
        n523 = event-data() -> ()  [unwired: 1 in, 5 out]
        n524 = flat-sequence {
          tunnel: w830 -> [w833]
          tunnel: w829 -> [w832]
          frame #0 {
            n525 = local read "Saved stage positions"() -> (w835:dbl[][])
            n526 = property on="Inject Pump 1" class="Bool (strict)"("Val(Sgnl)"=FALSE ("Inject Pump 2")) -> ()  [unwired: 2 in, 2 out]
            n527 = local write "Stage moving"(TRUE ("Stage moving")) -> ()
            n528 = call "move to saved stage position.vi"("error in"=w832, "Stage VISA resource name in"=w833, "Position"=1, "Saved Stage Positions"=w835) -> ()  [unwired: 2 out]
          }
          frame #1 {
            n529 = local read "Shutter 1 (B)"() -> (w837:bool)
            n530 = disable-structure shown="Disabled" {
              frame Disabled {
                n531 = property on="Inject Pump 2" class="Bool (strict)"("Val(Sgnl)"=TRUE ("Inject Pump 2")) -> ()  [unwired: 2 in, 2 out]
              }
              frame Enabled {
              }
            }
            n532 = local write "Stage moving"(FALSE ("Stage moving")) -> ()
            n533 = case shown="False" w837 {
              frame False {
                n534 = property on="Shutter 1 (B)" class="Bool (strict)"("Val(Sgnl)"=TRUE ("Value (Signaling)")) -> ()  [unwired: 2 in, 2 out]
              }
              frame True {
              }
            }
            n535 = call <vilib>:"Beep.vi"() -> ()  [unwired: 12 in]
          }
        }
        n536 = local write "Got ADig bead"(FALSE ("Got ADig bead")) -> ()
      }
      event "Set Position 1", "Set Position 2", "Set Position 3", "Set Position 4", "Set Position 5": Value Change {
        n537 = event-data() -> ()  [unwired: 1 in, 5 out]
        n538 = Build Array("Set Position 1", "Set Position 2", "Set Position 3", "Set Position 4", "Set Position 5") -> (w856:bool[])
        n539 = Boolean Array To Number(Boolean array=w856) -> (number=w855:u32)
        n540 = call "Read Stage Position.vi"("error in"=w843, "VISA resource name in"=w844) -> ("Current Position"=w841:cluster{dbl, dbl, dbl}, "error out"=→"Stage error":errorcluster)  [unwired: 1 in, 1 out]
        n541 = Logarithm Base 2(1:w855) -> (0:w849:dbl)
        n542 = Cluster To Array(cluster=w841) -> (array=w851:dbl[])
        n543 = Increment(x=w849) -> (x+1=w852:dbl)
        n544 = Build Array (concatenate)(w852, w851) -> (w850:dbl[])
        n545 = Replace Array Subset(array="Saved stage positions", new element=w850, index (row)=w849) -> (w853:dbl[][])  [unwired: 1 in]
        n546 = local write "Saved stage positions"(w853) -> ()
      }
      event "Move to Position 2", "Move to Position 4", "Move to Position 3", "Move to Position 5", "Move to Position 1": Value Change {
        n547 = event-data() -> ()  [unwired: 1 in, 5 out]
        n548 = Build Array("Move to Position 1", "Move to Position 2", "Move to Position 3", "Move to Position 4", "Move to Position 5") -> (w866:bool[])
        n549 = Boolean Array To Number(Boolean array=w866) -> (number=w865:u32)
        n550 = Logarithm Base 2(1:w865) -> (0:w864:dbl)
        n551 = flat-sequence {
          tunnel: w864 -> [w871]
          tunnel: w863 -> [w870]
          tunnel: w862 -> [w869]
          frame #0 {
            n552 = local read "Saved stage positions"() -> (w872:dbl[][])
            n553 = Increment(x=w871) -> (x+1=w868:dbl)
            n554 = call "move to saved stage position.vi"("error in"=w869, "Stage VISA resource name in"=w870, "Position"=w868, "Saved Stage Positions"=w872) -> ()  [unwired: 2 out]
            "Stage moving" <- TRUE ("Stage moving")
          }
          frame #1 {
            n555 = call <vilib>:"Beep.vi"() -> ()  [unwired: 12 in]
            n556 = local write "Stage moving"(FALSE ("Stage moving")) -> ()
          }
        }
      }
      event "Dip": Value Change {
        n557 = event-data() -> ()  [unwired: 1 in, 5 out]
        n558 = local write "Dip"(FALSE ("Dip")) -> ()
        n559 = flat-sequence {
          tunnel: w883 -> [w885]
          tunnel: w882 -> [w884]
          tunnel: [w886] -> w880
          tunnel: [w885] -> w878
          tunnel: [w884] -> w876
          tunnel: [w894] -> w881
          tunnel: w880 -> [w894]
          tunnel: [w893] -> w879
          tunnel: w878 -> [w893]
          tunnel: [w892] -> w877
          tunnel: w876 -> [w892]
          tunnel: w881 -> [w911]
          tunnel: w879 -> [w910]
          tunnel: w877 -> [w909]
          frame #0 {
            n560 = local read "Saved stage positions"() -> (w886:dbl[][])
            n561 = local write "Stage moving"(TRUE) -> ()
            n562 = call "move to saved stage position.vi"("error in"=w884, "Stage VISA resource name in"=w885, "Position"="Dip position", "Saved Stage Positions"=w886) -> ()  [unwired: 2 out]
          }
          frame #1 {
            n563 = node-c288() -> (w891:T12)  [unwired: 4 in]
            n564 = timed-loop {
              timing: w891 -> [_]
              timing-out: [_] -> w890
              i -> [w902]
              stop <- w898 stop-if-true
              n565 = node-c288() -> ()  [unwired: 1 in, 1 out]
              n566 = Greater Or Equal?(x=w902, y="Dip duration") -> (x >= y?=w897:bool)
              n567 = Or(x=w897, y="Cancel dwell") -> (x .or. y?=w895:bool)
              n568 = Not(x="Pause dwell") -> (.not. x?=w899:bool)
              n569 = node-c288() -> ()  [unwired: 1 in, 1 out]
              n570 = And(x=w899, y=w895) -> (x .and. y?=w898:bool)
              "Dip time" <- w902
            }
            n571 = local write "Stage moving"(FALSE ("Stage moving")) -> ()
            n572 = node-c288(w890) -> ()  [unwired: 1 out]
          }
          frame #2 {
            n573 = local write "Cancel dwell"(FALSE ("Cancel dwell")) -> ()
            n574 = call "move to saved stage position.vi"("error in"=w909, "Stage VISA resource name in"=w910, "Position"="Return position", "Saved Stage Positions"=w911) -> ()  [unwired: 2 out]
          }
          frame #3 {
            n575 = local write "Stage moving"(FALSE ("Stage moving")) -> ()
          }
        }
      }
      event "Force FB script": Value Change {
        n576 = event-data() -> ()  [unwired: 1 in, 5 out]
        n577 = flat-sequence {
          frame #0 {
            n578 = disable-structure shown="Disabled" {
              frame Disabled {
                n579 = local read "# Samples/channel"() -> (w915:i32)
                n580 = local write "# Samples/channel (in)"(w915) -> ()
              }
              frame Enabled {
              }
            }
            n581 = local write "Force FB script"(FALSE ("Force FB script")) -> ()
            n582 = property on="Trap delta" class="DigNum (strict)"("Val(Sgnl)"="Start trap delta (V)") -> ()  [unwired: 2 in, 2 out]
          }
          frame #1 {
            n583 = Wait (ms)(milliseconds to wait=u32 500) -> ()  [unwired: 1 out]
          }
          frame #2 {
            n584 = property on="Set reading to\nsetpoint" class="Bool (strict)"("Val(Sgnl)"=TRUE ("Value (Signaling)")) -> ()  [unwired: 2 in, 2 out]
          }
          frame #3 {
            n585 = Wait (ms)(milliseconds to wait=u32 300) -> ()  [unwired: 1 out]
          }
          frame #4 {
            n586 = local write "Force Feedback"(TRUE ("Force Feedback")) -> ()
            n587 = property on="Tabs" class="TabCtl (strict)"("Val(Sgnl)"=T3."Force Feedback" ("Value (Signaling)")) -> ()  [unwired: 2 in, 2 out]
          }
          frame #5 {
            n588 = property on="Save Data" class="Bool (strict)"("Val(Sgnl)"=TRUE ("Value (Signaling)")) -> ()  [unwired: 2 in, 2 out]
          }
          frame #6 {
            n589 = Multiply(x="Wait before dip (s)", y=1000) -> (x*y=w922:dbl)
            n590 = Wait (ms)(milliseconds to wait=w922) -> ()  [unwired: 1 out]
          }
          frame #7 {
            n591 = case shown="True" "Start dipping after?" {
              selector: "Start dipping after?" -> [_ w927]
              frame False {
              }
              frame True {
                n592 = property on="Dip" class="Bool (strict)"("Val(Sgnl)"=w927) -> ()  [unwired: 2 in, 2 out]
              }
            }
            n593 = property on="Remove offsets" class="Bool (strict)"("Val(Sgnl)"=TRUE ("Value (Signaling)")) -> ()  [unwired: 2 in, 2 out]
          }
        }
      }
      event "Move 0": Value Change {
        n594 = event-data() -> ()  [unwired: 1 in, 5 out]
        n595 = local write "Move 0"(FALSE) -> ()
        n596 = call "HalfWavePlate.vi"("Degrees"="\"Degrees\" 0", "Motor"=0) -> ()  [unwired: 1 in]
      }
      event "Move 1": Value Change {
        n597 = event-data() -> ()  [unwired: 1 in, 5 out]
        n598 = local write "Move 1"(FALSE) -> ()
        n599 = call "HalfWavePlate.vi"("Degrees"="\"Degrees\" 1", "Motor"=1) -> ()  [unwired: 1 in]
      }
      event "Stop": Value Change {
        n600 = event-data() -> ()  [unwired: 1 in, 5 out]
        n601 = local read "Stop"() -> (w934:bool)
      }
    }
    n602 = node-c288() -> ()  [unwired: 1 in, 1 out]
  }
  n603 = call <vilib>:"Simple Error Handler.vi"("error in (no error)"=w105) -> ()  [unwired: 4 in, 5 out]
  n604 = node-c288(2 ("Processor")) -> (w75:T12)  [unwired: 3 in]
  n605 = node-c288(2 ("Processor")) -> (w27:T12)  [unwired: 3 in]
  n606 = timed-loop {
    timing: w75 -> [_]
    timing-out: [_] -> w74
    stop <- w937 stop-if-true
    n607 = node-c288() -> ()  [unwired: 1 in, 1 out]
    n608 = case shown="\"Current Saved Data\"" "Tab Control" {
      frame "Control" {
        n609 = case shown="True" "Start" {
          frame False {
          }
          frame True {
            w950 = T15 3 items=["no dialog", "OK message", "continue or stop message", "OK message + warnings", "continue/stop + warnings"] ("type of dialog (OK msg:1)")
            n610 = call "InitializeAcquireFF.vi"("DAQ Rate"="DAQ Rate", "Averaging Number"="Averaging Number", "Sampling Rate"="Sampling Rate") -> ("error out"=w944:errorcluster, "task out"=w943:refnum<k21>, "Final Sampling Rate"=→"Final Sampling Rate":dbl)  [unwired: 4 in, 2 out]
            n611 = while {
              tunnel: [w962] -> w949
              tunnel: [w961] -> w942
              tunnel: "Averaging Number" -> [w960]
              tunnel: w944 -> [w959]
              tunnel: w943 -> [w957]
              stop <- w958 continue-if-true
              n612 = call "Acquire2_QPD.vi"("task/channels in"=w957, "Save Data?"=FALSE ("Take Data?"), "Averaging Number"=w960, "error in"=w959) -> ("PSD 1"=→"PSD 1":cluster{dbl[], dbl[]}, "PSD 1 Sum"=→"PSD 1 Sum":dbl, "PSD 2"=→"PSD 2":cluster{dbl[], dbl[]}, "PSD 2 Sum"=→"PSD 2 Sum":dbl, "task out"=w962:refnum<k21>, "error out"=w961:errorcluster)  [unwired: 14 in, 4 out]
              n613 = local read "Start"() -> (w958:bool)
            }
            n614 = call <vilib>:"DAQmx Clear Task.vi"("task in"=w949, "error in"=w942) -> ("error out"=w951:errorcluster)  [unwired: 13 in]
            n615 = call <vilib>:"Simple Error Handler.vi"("type of dialog (OK msg:1)"=w950, "error in (no error)"=w951) -> ()  [unwired: 3 in, 5 out]
          }
        }
      }
      frame "Current Saved Data" {
      }
      frame "Data Acquisition" {
      }
      frame "Raw QPD Data" {
      }
    }
    n616 = local read "Stop"() -> (w937:bool)
    n617 = node-c288() -> ()  [unwired: 1 in, 1 out]
  }
  n618 = timed-loop {
    timing: w27 -> [_]
    timing-out: [_] -> w26
    stop <- w963 stop-if-true
    n619 = node-c288() -> ()  [unwired: 1 in, 1 out]
    n620 = event shown="[0] \"Pause Mouse/Mirror Connection\": Value Change" {
      selector: _ -> [_ _]
      dyn-events: _ -> [_ _]
      timeout: _ -> [_ _]
      tunnel: [w1056 _] -> w964
      tunnel: [_ w1057] -> w963
      event "Pause Mouse/Mirror Connection": Value Change {
        n621 = event-data() -> ("NewVal"=w1056:bool)  [unwired: 1 in]
      }
      event "Stop": Value Change {
        n622 = event-data() -> ("NewVal"=w1057:bool)  [unwired: 1 in]
      }
    }
    n623 = case shown="True" w964 {
      frame False {
      }
      frame True {
        n624 = call "InitializeMouseControl.vi"() -> ("error out 2"=w973:errorcluster, "task out"=w974:refnum<k21>, "error out"=w976:errorcluster, "device ID"=w975:refnum<k1>)  [unwired: 8 in]
        n625 = while {
          tunnel: w976 -> [w988]
          tunnel: w975 -> [w987]
          tunnel: w974 -> [w986]
          tunnel: w973 -> [w985]
          tunnel: [w984] -> w971
          tunnel: [w983] -> w970
          tunnel: [w982] -> w967
          tunnel: [w981] -> w968
          stop <- w980 stop-if-true
          n626 = case shown="True" "Use Mouse to Move Trap?" {
            tunnel: w987 -> [w995 w1018]
            tunnel: w988 -> [w994 w1017]
            tunnel: w986 -> [w993 w1016]
            tunnel: w985 -> [w992 w1015]
            tunnel: [w995 w1014] -> w982
            tunnel: [w994 w1013] -> w981
            tunnel: [w993 w1012] -> w984
            tunnel: [w992 w1011] -> w983
            frame False {
              (unwired) FALSE ("button 1")
            }
            frame True {
              w1006 = 0.0 ("y")
              w1008 = 10
              n627 = local read "Deflection"() -> (w1019:T4)
              n628 = call-poly <vilib>:"Acquire Input Data.vi"("device ID"=w1018, "error in (no error)"=w1017) -> ("device ID"=w1014:refnum<k1>, "button info"=w1032:T16, "error out"=w1013:errorcluster)  [unwired: 14 in, 1 out]
              n629 = Unbundle By Name(w1019) -> ("Horizontal"=w1021:i32, "Vertical"=w1020:i32)
              n630 = local read "Saved voltage"() -> (w997:cluster{dbl, dbl})
              n631 = Divide(x=w1021, y=30) -> (x/y=w1024:dbl)
              n632 = Divide(x=w1020, y=-20) -> (x/y=w1025:dbl)
              n633 = Unbundle By Name(w1032) -> ("button 1"=w1010:bool, "button 2"=w1026:bool)
              n634 = Bundle(w1024, w1025) -> (w1002:cluster{dbl, dbl})  [unwired: 1 in]
              n635 = local write "Reference Voltage"(w1002) -> ()
              n636 = Add(x=w1002, y=w997) -> (x+y=w1030:cluster{dbl, dbl})
              n637 = case shown="True" w1010 {
                frame False {
                  n638 = stacked-sequence {
                    frame #0 {
                      n639 = local write "CoordinatesMousePressed"(T4 {"Horizontal"=0, "Vertical"=0} ("Coords when pressed")) -> ()
                      n640 = local write "Deflection"(T4 {"Horizontal"=0, "Vertical"=0} ("deflaction")) -> ()
                    }
                  }
                }
                frame True {
                  n641 = local read "CoordinatesMousePressed"() -> (w1055:T4)
                  n642 = local read "Real Coordinates"() -> (w1054:cluster{"Horizontal":i32, "Vertical":i32})
                  n643 = Subtract(x=w1054, y=w1055) -> (x-y=w1053:T4)
                  n644 = local write "Deflection"(w1053) -> ()
                }
              }
              n645 = Unbundle(w1030) -> (w1007:dbl, w998:dbl)
              n646 = case shown="True" w1026 {
                frame False {
                }
                frame True {
                  n647 = local read "Reference Voltage"() -> (w1036:cluster{dbl, dbl})
                  n648 = local read "Saved voltage"() -> (w1034:cluster{dbl, dbl})
                  n649 = Add(x=w1036, y=w1034) -> (x+y=→"Saved voltage":cluster{dbl, dbl})
                  n650 = local read "Real Coordinates"() -> (w1035:cluster{"Horizontal":i32, "Vertical":i32})
                  n651 = local write "CoordinatesMousePressed"(w1035) -> ()
                }
              }
              n652 = Less?(x=w1007, y=w1008) -> (x < y?=w1005:bool)
              n653 = Greater?(x=w1007, y=w1006) -> (0:w1004:bool)
              n654 = Greater?(x=w998, y=w1006) -> (0:w1000:bool)
              n655 = Less?(x=w998, y=w1008) -> (x < y?=w1001:bool)
              n656 = And(x=w1000, y=w1001) -> (x .and. y?=w999:bool)
              n657 = And(x=w1005, y=w1004) -> (x .and. y?=w1003:bool)
              n658 = case shown="False" w999 {
                tunnel: [w1046 w1050] -> w1009
                tunnel: w998 -> [w1044 w1050]
                frame False {
                  n659 = Greater?(x=w1044, y=10.0) -> (0:w1047:bool)
                  n660 = case shown="True" w1047 {
                    tunnel: [0.0 10.0] -> w1046
                    frame False {
                    }
                    frame True {
                    }
                  }
                }
                frame True {
                }
              }
              n661 = case shown="False" w1003 {
                tunnel: w1007 -> [w1038 w1043]
                tunnel: [w1039 w1043] -> w1031
                frame False {
                  n662 = Greater?(x=w1038, y=10.0) -> (0:w1040:bool)
                  n663 = case shown="True" w1040 {
                    tunnel: [0.0 10.0] -> w1039
                    frame False {
                    }
                    frame True {
                    }
                  }
                }
                frame True {
                }
              }
              n664 = Bundle(w1031, w1009) -> (w996:cluster{dbl, dbl})  [unwired: 1 in]
              n665 = Cluster To Array(cluster=w996) -> (array=w1027:dbl[])
              n666 = call-poly <vilib>:"DAQmx Write.vi"("task/channels in"=w1016, "data"=w1027, "error in"=w1015) -> ("task out"=w1029:refnum<k21>, "error out"=w1028:errorcluster)  [unwired: 10 in, 1 out]
              n667 = call <vilib>:"DAQmx Is Task Done.vi"("task/channels in"=w1029, "error in"=w1028) -> ("task out"=w1012:refnum<k21>, "error out"=w1011:errorcluster)  [unwired: 11 in, 1 out]
            }
          }
          n668 = event shown="[0] \"Pane\": Mouse Move" {
            selector: _ -> [_ _ _]
            dyn-events: _ -> [_ _ _]
            timeout: _ -> [_ _ _]
            event Mouse Move {
              n669 = event-data() -> ("Coords"=w990:T4)  [unwired: 1 in]
              n670 = local write "Real Coordinates"(w990) -> ()
            }
            event Mouse Down {
              n671 = event-data() -> ("Coords"=w991:T4)  [unwired: 1 in]
              n672 = local write "CoordinatesMousePressed"(w991) -> ()
            }
            event "Pause Mouse/Mirror Connection": Value Change {
              n673 = event-data() -> ()  [unwired: 1 in, 3 out]
            }
          }
          n674 = local read "Stop"() -> (w977:bool)
          n675 = Not(x="Pause Mouse/Mirror Connection") -> (.not. x?=w978:bool)
          n676 = Or(x=w978, y=w977) -> (x .or. y?=w980:bool)
        }
        n677 = call <vilib>:"DAQmx Clear Task.vi"("task in"=w971, "error in"=w970) -> ("error out"=w972:errorcluster)  [unwired: 13 in]
        n678 = call <vilib>:"Simple Error Handler.vi"("error in (no error)"=w972) -> ()  [unwired: 4 in, 5 out]
        n679 = call-poly <vilib>:"Close Input Device.vi"("error in (no error)"=w968, "device ID"=w967) -> ("error out"=w969:errorcluster)  [unwired: 8 in]
        n680 = call <vilib>:"Simple Error Handler.vi"("error in (no error)"=w969) -> ()  [unwired: 4 in, 5 out]
      }
    }
    n681 = node-c288() -> ()  [unwired: 1 in, 1 out]
  }
  n682 = call-poly <vilib>:"DAQmx Create Virtual Channel.vi"("lines"=w92) -> ("task out"=w91:refnum<k21>)  [unwired: 13 in, 1 out]
  n683 = call-poly <vilib>:"DAQmx Create Virtual Channel.vi"("lines"=w95) -> ("task out"=w94:refnum<k21>)  [unwired: 13 in, 1 out]
  n684 = node-c288(i64 100 ("Period")) -> (w89:T12)  [unwired: 3 in]
  n685 = timed-loop {
    tunnel: w91 -> [w1060]
    tunnel: [w1059] -> w90
    tunnel: w94 -> [w1062]
    tunnel: [w1061] -> w93
    timing: w89 -> [_]
    timing-out: [_] -> w88
    stop <- w1058 stop-if-true
    n686 = node-c288() -> ()  [unwired: 1 in, 1 out]
    n687 = event shown="[1] \"Shutter 2 (A)\": Value Change" {
      selector: _ -> [_ _ _]
      dyn-events: _ -> [_ _ _]
      timeout: _ -> [_ _ _]
      tunnel: w1062 -> [w1066 _ _]
      tunnel: [w1065 _ _] -> w1061
      tunnel: w1060 -> [_ w1086 _]
      tunnel: [_ w1084 _] -> w1059
      tunnel: [_ _ w1103] -> w1058
      event "Shutter 1 (B)": Value Change {
        n688 = event-data() -> ()  [unwired: 1 in, 1 out]
        n689 = flat-sequence {
          tunnel: [w1072] -> w1069
          tunnel: w1066 -> [w1071]
          tunnel: [w1076] -> w1068
          tunnel: [w1079] -> w1067
          tunnel: w1069 -> [w1074]
          tunnel: w1068 -> [w1083]
          tunnel: w1067 -> [w1081]
          tunnel: [w1080] -> w1065
          frame #0 {
            n690 = call-poly <vilib>:"DAQmx Write.vi"("task/channels in"=w1071, "data"=FALSE) -> ("task out"=w1072:refnum<k21>)  [unwired: 11 in, 2 out]
            n691 = Wait (ms)(milliseconds to wait=100) -> ()  [unwired: 1 out]
          }
          frame #1 {
            n692 = Or(x="Shutter 1 (B)", y=TRUE) -> (x .or. y?=w1076:bool)
            n693 = call-poly <vilib>:"DAQmx Write.vi"("task/channels in"=w1074, "data"=w1076) -> ("task out"=w1079:refnum<k21>)  [unwired: 11 in, 2 out]
            n694 = Wait (ms)(milliseconds to wait=100) -> ()  [unwired: 1 out]
          }
          frame #2 {
            n695 = Not(x=w1083) -> (.not. x?=w1082:bool)
            n696 = call-poly <vilib>:"DAQmx Write.vi"("task/channels in"=w1081, "data"=w1082) -> ("task out"=w1080:refnum<k21>)  [unwired: 11 in, 2 out]
          }
        }
      }
      event "Shutter 2 (A)": Value Change {
        n697 = event-data() -> ()  [unwired: 1 in, 1 out]
        n698 = flat-sequence {
          tunnel: w1086 -> [w1091]
          tunnel: [w1090] -> w1085
          tunnel: [w1095] -> w1088
          tunnel: [w1098] -> w1087
          tunnel: w1085 -> [w1093]
          tunnel: w1088 -> [w1102]
          tunnel: w1087 -> [w1100]
          tunnel: [w1099] -> w1084
          frame #0 {
            n699 = call-poly <vilib>:"DAQmx Write.vi"("task/channels in"=w1091, "data"=FALSE) -> ("task out"=w1090:refnum<k21>)  [unwired: 11 in, 2 out]
            n700 = Wait (ms)(milliseconds to wait=100) -> ()  [unwired: 1 out]
          }
          frame #1 {
            n701 = Or(x="Shutter 2 (A)", y=TRUE) -> (x .or. y?=w1095:bool)
            n702 = call-poly <vilib>:"DAQmx Write.vi"("task/channels in"=w1093, "data"=w1095) -> ("task out"=w1098:refnum<k21>)  [unwired: 11 in, 2 out]
            n703 = Wait (ms)(milliseconds to wait=100) -> ()  [unwired: 1 out]
          }
          frame #2 {
            n704 = Not(x=w1102) -> (.not. x?=w1101:bool)
            n705 = call-poly <vilib>:"DAQmx Write.vi"("task/channels in"=w1100, "data"=w1101) -> ("task out"=w1099:refnum<k21>)  [unwired: 11 in, 2 out]
          }
        }
      }
      event "Stop": Value Change {
        n706 = event-data() -> ("NewVal"=w1103:bool)  [unwired: 1 in, 5 out]
      }
    }
    n707 = node-c288() -> ()  [unwired: 1 in, 1 out]
  }
  n708 = node-c288(w88) -> ()  [unwired: 1 out]
  n709 = node-c288(w74) -> ()  [unwired: 1 out]
  n710 = call <vilib>:"DAQmx Clear Task.vi"("task in"=w90) -> ()  [unwired: 14 in, 1 out]
  n711 = call <vilib>:"DAQmx Clear Task.vi"("task in"=w93) -> ()  [unwired: 14 in, 1 out]
  n712 = node-c288(w26) -> ()  [unwired: 1 out]
  n713 = node-c288(w22) -> ()  [unwired: 1 out]
  n714 = disable-structure shown="Enabled" {
    frame Disabled {
      n715 = node-c288(2 ("Processor")) -> (w1107:T12)  [unwired: 3 in]
      n716 = timed-loop "Pump Control" {
        timing: w1107 -> [_]
        timing-out: [_] -> w1106
        tunnel: refnum<visa-resource-name> "COM6" ("VISA resource name") -> [w1109]
        stop <- w1108 stop-if-true
        n717 = node-c288() -> ()  [unwired: 1 in, 1 out]
        n718 = event shown="[4] \"Inject Pump 1\": Value Change" {
          selector: _ -> [_ _ _ _ _ _ _ _ _]
          dyn-events: _ -> [_ _ _ _ _ _ _ _ _]
          timeout: _ -> [_ _ _ _ _ _ _ _ _]
          tunnel: w1109 -> [w1117 w1213 _ w1289 w1417 w1560 w1605 w1663 w1722]
          tunnel: [_ _ w1288 _ _ _ _ _ _] -> w1108
          event "Flush Pump 1": Value Change {
            w1118 = "\r"
            n719 = event-data() -> ()  [unwired: 1 in, 5 out]
            n720 = call-poly "VISA Configure Serial Port"("VISA resource name"=w1117) -> ("VISA resource name out"=w1131:refnum<visa-resource-name>, "error out"=w1132:errorcluster)  [unwired: 13 in]
            n721 = local read "Write Wait"() -> (w1110:i32)
            n722 = Concatenate Strings("enter pump1", w1118) -> (w1119:string)
            n723 = flat-sequence {
              tunnel: w1132 -> [w1151]
              tunnel: w1131 -> [w1153]
              tunnel: [w1152] -> w1148
              tunnel: [w1150] -> w1147
              tunnel: w1119 -> [w1149]
              tunnel: w1148 -> [w1156]
              tunnel: [w1156] -> w1146
              tunnel: w1147 -> [w1155]
              tunnel: [w1155] -> w1145
              tunnel: w1110 -> [w1154]
              tunnel: [w1161] -> w1144
              tunnel: w1124 -> [w1160]
              tunnel: [w1157] -> w1143
              tunnel: w1146 -> [w1159]
              tunnel: w1145 -> [w1158]
              tunnel: w1144 -> [w1164]
              tunnel: [w1164] -> w1142
              tunnel: [w1163] -> w1141
              tunnel: w1143 -> [w1163]
              tunnel: w1110 -> [w1162]
              tunnel: w1142 -> [w1169]
              tunnel: [w1168] -> w1140
              tunnel: w1127 -> [w1167]
              tunnel: w1141 -> [w1166]
              tunnel: [w1165] -> w1139
              tunnel: w1140 -> [w1172]
              tunnel: [w1172] -> w1138
              tunnel: [w1171] -> w1137
              tunnel: w1139 -> [w1171]
              tunnel: w1110 -> [w1170]
              tunnel: w1138 -> [w1177]
              tunnel: [w1176] -> w1136
              tunnel: w1130 -> [w1175]
              tunnel: w1137 -> [w1174]
              tunnel: [w1173] -> w1135
              tunnel: [w1180] -> w1134
              tunnel: w1136 -> [w1180]
              tunnel: [w1179] -> w1133
              tunnel: w1135 -> [w1179]
              tunnel: w1110 -> [w1178]
              tunnel: w1134 -> [w1185]
              tunnel: w1133 -> [w1182]
              tunnel: [w1184] -> w1113
              tunnel: [w1183] -> w1111
              tunnel: [w1190] -> w1114
              tunnel: w1113 -> [w1190]
              tunnel: [w1189] -> w1112
              tunnel: w1111 -> [w1189]
              tunnel: w1110 -> [w1188]
              tunnel: w1114 -> [w1192]
              tunnel: w1112 -> [w1191]
              frame #0 {
                n724 = VISA Write(VISA resource name=w1153, write buffer=w1149, error in (no error)=w1151) -> (VISA resource name out=w1152:refnum<visa-resource-name>, error out=w1150:errorcluster)  [unwired: 1 out]
              }
              frame #1 {
                n725 = Wait (ms)(milliseconds to wait=w1154) -> ()  [unwired: 1 out]
              }
              frame #2 {
                n726 = VISA Write(VISA resource name=w1159, write buffer=w1160, error in (no error)=w1158) -> (VISA resource name out=w1161:refnum<visa-resource-name>, error out=w1157:errorcluster)  [unwired: 1 out]
              }
              frame #3 {
                n727 = Wait (ms)(milliseconds to wait=w1162) -> ()  [unwired: 1 out]
              }
              frame #4 {
                n728 = VISA Write(VISA resource name=w1169, write buffer=w1167, error in (no error)=w1166) -> (VISA resource name out=w1168:refnum<visa-resource-name>, error out=w1165:errorcluster)  [unwired: 1 out]
              }
              frame #5 {
                n729 = Wait (ms)(milliseconds to wait=w1170) -> ()  [unwired: 1 out]
              }
              frame #6 {
                n730 = VISA Write(VISA resource name=w1177, write buffer=w1175, error in (no error)=w1174) -> (VISA resource name out=w1176:refnum<visa-resource-name>, error out=w1173:errorcluster)  [unwired: 1 out]
              }
              frame #7 {
                n731 = Wait (ms)(milliseconds to wait=w1178) -> ()  [unwired: 1 out]
              }
              frame #8 {
                n732 = Concatenate Strings("start ", "\r") -> (w1181:string)
                n733 = VISA Write(VISA resource name=w1185, write buffer=w1181, error in (no error)=w1182) -> (VISA resource name out=w1184:refnum<visa-resource-name>, error out=w1183:errorcluster)  [unwired: 1 out]
              }
              frame #9 {
                n734 = Wait (ms)(milliseconds to wait=w1188) -> ()  [unwired: 1 out]
              }
              frame #10 {
                n735 = local write "Flush Pump 1"(FALSE ("Flush Pump 1")) -> ()
                n736 = Concatenate Strings("enter main ", "\r") -> (w1196:string)
                n737 = VISA Write(VISA resource name=w1192, write buffer=w1196, error in (no error)=w1191) -> (VISA resource name out=w1195:refnum<visa-resource-name>, error out=w1194:errorcluster)  [unwired: 1 out]
                n738 = VISA Close(VISA resource name=w1195, error in (no error)=w1194) -> ()  [unwired: 1 out]
              }
            }
            n739 = Concatenate Strings("set units 4 ", w1118) -> (w1124:string)
            n740 = Multiply(x="Flush\nRate (ul/min)", y=60) -> (x*y=w1122:dbl)
            n741 = Number To Decimal String(number=w1122) -> (decimal integer string=w1125:string)  [unwired: 1 in]
            n742 = Concatenate Strings("set rate ", w1125, w1118) -> (w1127:string)
            n743 = Number To Decimal String(number="Flush\nVolume (ul)") -> (decimal integer string=w1129:string)  [unwired: 1 in]
            n744 = Concatenate Strings("set volume ", w1129, w1118) -> (w1130:string)
          }
          event "Flush Pump 2": Value Change {
            w1204 = "\r"
            n745 = event-data() -> ()  [unwired: 1 in, 5 out]
            n746 = call-poly "VISA Configure Serial Port"("VISA resource name"=w1213) -> ("VISA resource name out"=w1224:refnum<visa-resource-name>, "error out"=w1225:errorcluster)  [unwired: 13 in]
            n747 = local read "Write Wait"() -> (w1199:i32)
            n748 = Concatenate Strings("enter pump2", w1204) -> (w1205:string)
            n749 = flat-sequence {
              tunnel: w1225 -> [w1240]
              tunnel: w1224 -> [w1242]
              tunnel: [w1241] -> w1210
              tunnel: [w1239] -> w1208
              tunnel: w1205 -> [w1238]
              tunnel: w1210 -> [w1245]
              tunnel: [w1245] -> w1209
              tunnel: w1208 -> [w1244]
              tunnel: [w1244] -> w1207
              tunnel: w1199 -> [w1243]
              tunnel: [w1250] -> w1237
              tunnel: w1217 -> [w1249]
              tunnel: [w1246] -> w1236
              tunnel: w1209 -> [w1248]
              tunnel: w1207 -> [w1247]
              tunnel: w1237 -> [w1253]
              tunnel: [w1253] -> w1235
              tunnel: [w1252] -> w1234
              tunnel: w1236 -> [w1252]
              tunnel: w1199 -> [w1251]
              tunnel: w1235 -> [w1258]
              tunnel: [w1257] -> w1233
              tunnel: w1220 -> [w1256]
              tunnel: w1234 -> [w1255]
              tunnel: [w1254] -> w1232
              tunnel: w1233 -> [w1261]
              tunnel: [w1261] -> w1231
              tunnel: [w1260] -> w1230
              tunnel: w1232 -> [w1260]
              tunnel: w1199 -> [w1259]
              tunnel: w1231 -> [w1266]
              tunnel: [w1265] -> w1229
              tunnel: w1223 -> [w1264]
              tunnel: w1230 -> [w1263]
              tunnel: [w1262] -> w1228
              tunnel: [w1269] -> w1227
              tunnel: w1229 -> [w1269]
              tunnel: [w1268] -> w1226
              tunnel: w1228 -> [w1268]
              tunnel: w1199 -> [w1267]
              tunnel: w1227 -> [w1276]
              tunnel: w1226 -> [w1275]
              tunnel: [w1271] -> w1203
              tunnel: [w1270] -> w1201
              tunnel: w1203 -> [w1279]
              tunnel: [w1279] -> w1202
              tunnel: w1201 -> [w1278]
              tunnel: [w1278] -> w1200
              tunnel: w1199 -> [w1277]
              tunnel: w1202 -> [w1283]
              tunnel: w1200 -> [w1282]
              frame #0 {
                n750 = VISA Write(VISA resource name=w1242, write buffer=w1238, error in (no error)=w1240) -> (VISA resource name out=w1241:refnum<visa-resource-name>, error out=w1239:errorcluster)  [unwired: 1 out]
              }
              frame #1 {
                n751 = Wait (ms)(milliseconds to wait=w1243) -> ()  [unwired: 1 out]
              }
              frame #2 {
                n752 = VISA Write(VISA resource name=w1248, write buffer=w1249, error in (no error)=w1247) -> (VISA resource name out=w1250:refnum<visa-resource-name>, error out=w1246:errorcluster)  [unwired: 1 out]
              }
              frame #3 {
                n753 = Wait (ms)(milliseconds to wait=w1251) -> ()  [unwired: 1 out]
              }
              frame #4 {
                n754 = VISA Write(VISA resource name=w1258, write buffer=w1256, error in (no error)=w1255) -> (VISA resource name out=w1257:refnum<visa-resource-name>, error out=w1254:errorcluster)  [unwired: 1 out]
              }
              frame #5 {
                n755 = Wait (ms)(milliseconds to wait=w1259) -> ()  [unwired: 1 out]
              }
              frame #6 {
                n756 = VISA Write(VISA resource name=w1266, write buffer=w1264, error in (no error)=w1263) -> (VISA resource name out=w1265:refnum<visa-resource-name>, error out=w1262:errorcluster)  [unwired: 1 out]
              }
              frame #7 {
                n757 = Wait (ms)(milliseconds to wait=w1267) -> ()  [unwired: 1 out]
              }
              frame #8 {
                n758 = Concatenate Strings("start ", "\r") -> (w1274:string)
                n759 = VISA Write(VISA resource name=w1276, write buffer=w1274, error in (no error)=w1275) -> (VISA resource name out=w1271:refnum<visa-resource-name>, error out=w1270:errorcluster)  [unwired: 1 out]
              }
              frame #9 {
                n760 = Wait (ms)(milliseconds to wait=w1277) -> ()  [unwired: 1 out]
              }
              frame #10 {
                n761 = local write "Flush Pump 2"(FALSE ("Flush Pump 1")) -> ()
                n762 = Concatenate Strings("enter main ", "\r") -> (w1284:string)
                n763 = VISA Write(VISA resource name=w1283, write buffer=w1284, error in (no error)=w1282) -> (VISA resource name out=w1281:refnum<visa-resource-name>, error out=w1280:errorcluster)  [unwired: 1 out]
                n764 = VISA Close(VISA resource name=w1281, error in (no error)=w1280) -> ()  [unwired: 1 out]
              }
            }
            n765 = Concatenate Strings("set units 4 ", w1204) -> (w1217:string)
            n766 = Multiply(x="Flush \nRate (ul/min)  2", y=60) -> (x*y=w1215:dbl)
            n767 = Number To Decimal String(number=w1215) -> (decimal integer string=w1218:string)  [unwired: 1 in]
            n768 = Concatenate Strings("set rate ", w1218, w1204) -> (w1220:string)
            n769 = Number To Decimal String(number="Flush\nVolume (ul)  2") -> (decimal integer string=w1222:string)  [unwired: 1 in]
            n770 = Concatenate Strings("set volume ", w1222, w1204) -> (w1223:string)
          }
          event "Stop": Value Change {
            n771 = event-data() -> ()  [unwired: 1 in, 5 out]
            n772 = local read "Stop"() -> (w1288:bool)
          }
          event "Inject Pump 2": Value Change {
            n773 = event-data() -> ()  [unwired: 1 in, 5 out]
            n774 = case shown="True" "Inject Pump 2" {
              tunnel: w1289 -> [w1292 w1334]
              frame False {
                n775 = local read "Write Wait"() -> (w1291:i32)
                n776 = call-poly "VISA Configure Serial Port"("VISA resource name"=w1292) -> ("VISA resource name out"=w1296:refnum<visa-resource-name>, "error out"=w1297:errorcluster)  [unwired: 13 in]
                n777 = Concatenate Strings("enter pump2", "\r") -> (w1294:string)
                n778 = flat-sequence {
                  tunnel: w1297 -> [w1308]
                  tunnel: w1296 -> [w1310]
                  tunnel: [w1309] -> w1305
                  tunnel: [w1307] -> w1304
                  tunnel: w1294 -> [w1306]
                  tunnel: w1305 -> [w1313]
                  tunnel: w1304 -> [w1312]
                  tunnel: [w1313] -> w1303
                  tunnel: [w1312] -> w1302
                  tunnel: w1291 -> [w1311]
                  tunnel: [w1317] -> w1301
                  tunnel: [w1316] -> w1300
                  tunnel: w1303 -> [w1315]
                  tunnel: w1302 -> [w1314]
                  tunnel: w1301 -> [w1323]
                  tunnel: [w1323] -> w1299
                  tunnel: w1300 -> [w1322]
                  tunnel: [w1322] -> w1298
                  tunnel: w1291 -> [w1321]
                  tunnel: w1299 -> [w1327]
                  tunnel: w1298 -> [w1326]
                  frame #0 {
                    n779 = VISA Write(VISA resource name=w1310, write buffer=w1306, error in (no error)=w1308) -> (VISA resource name out=w1309:refnum<visa-resource-name>, error out=w1307:errorcluster)  [unwired: 1 out]
                  }
                  frame #1 {
                    n780 = Wait (ms)(milliseconds to wait=w1311) -> ()  [unwired: 1 out]
                  }
                  frame #2 {
                    n781 = Concatenate Strings("stop ", "\r") -> (w1320:string)
                    n782 = VISA Write(VISA resource name=w1315, write buffer=w1320, error in (no error)=w1314) -> (VISA resource name out=w1317:refnum<visa-resource-name>, error out=w1316:errorcluster)  [unwired: 1 out]
                  }
                  frame #3 {
                    n783 = Wait (ms)(milliseconds to wait=w1321) -> ()  [unwired: 1 out]
                  }
                  frame #4 {
                    n784 = Concatenate Strings("enter main ", "\r") -> (w1328:string)
                    n785 = VISA Write(VISA resource name=w1327, write buffer=w1328, error in (no error)=w1326) -> (VISA resource name out=w1325:refnum<visa-resource-name>, error out=w1324:errorcluster)  [unwired: 1 out]
                    n786 = VISA Close(VISA resource name=w1325, error in (no error)=w1324) -> ()  [unwired: 1 out]
                  }
                }
              }
              frame True {
                w1347 = "\r"
                n787 = call-poly "VISA Configure Serial Port"("VISA resource name"=w1334) -> ("VISA resource name out"=w1336:refnum<visa-resource-name>, "error out"=w1335:errorcluster)  [unwired: 13 in]
                n788 = local read "Write Wait"() -> (w1331:i32)
                n789 = Concatenate Strings("enter pump2", w1347) -> (w1346:string)
                n790 = flat-sequence {
                  tunnel: w1335 -> [w1370]
                  tunnel: w1336 -> [w1372]
                  tunnel: [w1371] -> w1367
                  tunnel: [w1369] -> w1366
                  tunnel: w1346 -> [w1368]
                  tunnel: w1367 -> [w1375]
                  tunnel: [w1375] -> w1365
                  tunnel: w1366 -> [w1374]
                  tunnel: [w1374] -> w1364
                  tunnel: w1331 -> [w1373]
                  tunnel: [w1380] -> w1363
                  tunnel: w1343 -> [w1379]
                  tunnel: [w1376] -> w1362
                  tunnel: w1365 -> [w1378]
                  tunnel: w1364 -> [w1377]
                  tunnel: w1363 -> [w1383]
                  tunnel: [w1383] -> w1361
                  tunnel: [w1382] -> w1360
                  tunnel: w1362 -> [w1382]
                  tunnel: w1331 -> [w1381]
                  tunnel: w1361 -> [w1388]
                  tunnel: [w1387] -> w1359
                  tunnel: w1340 -> [w1386]
                  tunnel: w1360 -> [w1385]
                  tunnel: [w1384] -> w1358
                  tunnel: w1359 -> [w1391]
                  tunnel: [w1391] -> w1357
                  tunnel: [w1390] -> w1356
                  tunnel: w1358 -> [w1390]
                  tunnel: w1331 -> [w1389]
                  tunnel: w1357 -> [w1396]
                  tunnel: [w1395] -> w1355
                  tunnel: w1337 -> [w1394]
                  tunnel: w1356 -> [w1393]
                  tunnel: [w1392] -> w1354
                  tunnel: [w1399] -> w1353
                  tunnel: w1355 -> [w1399]
                  tunnel: [w1398] -> w1352
                  tunnel: w1354 -> [w1398]
                  tunnel: w1331 -> [w1397]
                  tunnel: w1353 -> [w1406]
                  tunnel: w1352 -> [w1405]
                  tunnel: [w1401] -> w1351
                  tunnel: [w1400] -> w1350
                  tunnel: w1351 -> [w1409]
                  tunnel: [w1409] -> w1349
                  tunnel: w1350 -> [w1408]
                  tunnel: [w1408] -> w1348
                  tunnel: w1331 -> [w1407]
                  tunnel: w1349 -> [w1413]
                  tunnel: w1348 -> [w1412]
                  frame #0 {
                    n791 = VISA Write(VISA resource name=w1372, write buffer=w1368, error in (no error)=w1370) -> (VISA resource name out=w1371:refnum<visa-resource-name>, error out=w1369:errorcluster)  [unwired: 1 out]
                  }
                  frame #1 {
                    n792 = Wait (ms)(milliseconds to wait=w1373) -> ()  [unwired: 1 out]
                  }
                  frame #2 {
                    n793 = VISA Write(VISA resource name=w1378, write buffer=w1379, error in (no error)=w1377) -> (VISA resource name out=w1380:refnum<visa-resource-name>, error out=w1376:errorcluster)  [unwired: 1 out]
                  }
                  frame #3 {
                    n794 = Wait (ms)(milliseconds to wait=w1381) -> ()  [unwired: 1 out]
                  }
                  frame #4 {
                    n795 = VISA Write(VISA resource name=w1388, write buffer=w1386, error in (no error)=w1385) -> (VISA resource name out=w1387:refnum<visa-resource-name>, error out=w1384:errorcluster)  [unwired: 1 out]
                  }
                  frame #5 {
                    n796 = Wait (ms)(milliseconds to wait=w1389) -> ()  [unwired: 1 out]
                  }
                  frame #6 {
                    n797 = VISA Write(VISA resource name=w1396, write buffer=w1394, error in (no error)=w1393) -> (VISA resource name out=w1395:refnum<visa-resource-name>, error out=w1392:errorcluster)  [unwired: 1 out]
                  }
                  frame #7 {
                    n798 = Wait (ms)(milliseconds to wait=w1397) -> ()  [unwired: 1 out]
                  }
                  frame #8 {
                    n799 = Concatenate Strings("start ", "\r") -> (w1404:string)
                    n800 = VISA Write(VISA resource name=w1406, write buffer=w1404, error in (no error)=w1405) -> (VISA resource name out=w1401:refnum<visa-resource-name>, error out=w1400:errorcluster)  [unwired: 1 out]
                  }
                  frame #9 {
                    n801 = Wait (ms)(milliseconds to wait=w1407) -> ()  [unwired: 1 out]
                  }
                  frame #10 {
                    n802 = Concatenate Strings("enter main ", "\r") -> (w1414:string)
                    n803 = VISA Write(VISA resource name=w1413, write buffer=w1414, error in (no error)=w1412) -> (VISA resource name out=w1411:refnum<visa-resource-name>, error out=w1410:errorcluster)  [unwired: 1 out]
                    n804 = VISA Close(VISA resource name=w1411, error in (no error)=w1410) -> ()  [unwired: 1 out]
                  }
                }
                n805 = local read "Normal \nRate (ul/hr)  2"() -> (w1332:dbl)
                n806 = Concatenate Strings("set units 4 ", w1347) -> (w1343:string)
                n807 = local read "Normal \nVolume (ul) 2"() -> (w1333:dbl)
                n808 = Number To Decimal String(number=w1332) -> (decimal integer string=w1342:string)  [unwired: 1 in]
                n809 = Concatenate Strings("set rate ", w1342, w1347) -> (w1340:string)
                n810 = Number To Decimal String(number=w1333) -> (decimal integer string=w1338:string)  [unwired: 1 in]
                n811 = Concatenate Strings("set volume ", w1338, w1347) -> (w1337:string)
              }
            }
          }
          event "Inject Pump 1": Value Change {
            n812 = event-data() -> ()  [unwired: 1 in, 5 out]
            n813 = case shown="True" "Inject Pump 1" {
              tunnel: w1417 -> [w1420 w1462]
              frame False {
                n814 = local read "Write Wait"() -> (w1419:i32)
                n815 = call-poly "VISA Configure Serial Port"("VISA resource name"=w1420) -> ("VISA resource name out"=w1424:refnum<visa-resource-name>, "error out"=w1425:errorcluster)  [unwired: 13 in]
                n816 = Concatenate Strings("enter pump1", "\r") -> (w1422:string)
                n817 = flat-sequence {
                  tunnel: w1425 -> [w1436]
                  tunnel: w1424 -> [w1438]
                  tunnel: [w1437] -> w1433
                  tunnel: [w1435] -> w1432
                  tunnel: w1422 -> [w1434]
                  tunnel: w1433 -> [w1441]
                  tunnel: w1432 -> [w1440]
                  tunnel: [w1441] -> w1431
                  tunnel: [w1440] -> w1430
                  tunnel: w1419 -> [w1439]
                  tunnel: [w1445] -> w1429
                  tunnel: [w1444] -> w1428
                  tunnel: w1431 -> [w1443]
                  tunnel: w1430 -> [w1442]
                  tunnel: w1429 -> [w1451]
                  tunnel: [w1451] -> w1427
                  tunnel: w1428 -> [w1450]
                  tunnel: [w1450] -> w1426
                  tunnel: w1419 -> [w1449]
                  tunnel: w1427 -> [w1455]
                  tunnel: w1426 -> [w1454]
                  frame #0 {
                    n818 = VISA Write(VISA resource name=w1438, write buffer=w1434, error in (no error)=w1436) -> (VISA resource name out=w1437:refnum<visa-resource-name>, error out=w1435:errorcluster)  [unwired: 1 out]
                  }
                  frame #1 {
                    n819 = Wait (ms)(milliseconds to wait=w1439) -> ()  [unwired: 1 out]
                  }
                  frame #2 {
                    n820 = Concatenate Strings("stop ", "\r") -> (w1448:string)
                    n821 = VISA Write(VISA resource name=w1443, write buffer=w1448, error in (no error)=w1442) -> (VISA resource name out=w1445:refnum<visa-resource-name>, error out=w1444:errorcluster)  [unwired: 1 out]
                  }
                  frame #3 {
                    n822 = Wait (ms)(milliseconds to wait=w1449) -> ()  [unwired: 1 out]
                  }
                  frame #4 {
                    n823 = Concatenate Strings("enter main ", "\r") -> (w1456:string)
                    n824 = VISA Write(VISA resource name=w1455, write buffer=w1456, error in (no error)=w1454) -> (VISA resource name out=w1453:refnum<visa-resource-name>, error out=w1452:errorcluster)  [unwired: 1 out]
                    n825 = VISA Close(VISA resource name=w1453, error in (no error)=w1452) -> ()  [unwired: 1 out]
                  }
                }
              }
              frame True {
                w1475 = "\r"
                n826 = call-poly "VISA Configure Serial Port"("VISA resource name"=w1462) -> ("VISA resource name out"=w1464:refnum<visa-resource-name>, "error out"=w1463:errorcluster)  [unwired: 13 in]
                n827 = local read "Write Wait"() -> (w1459:i32)
                n828 = flat-sequence {
                  tunnel: w1463 -> [w1498]
                  tunnel: w1464 -> [w1500]
                  tunnel: [w1499] -> w1495
                  tunnel: [w1497] -> w1494
                  tunnel: w1474 -> [w1496]
                  tunnel: w1495 -> [w1503]
                  tunnel: [w1503] -> w1493
                  tunnel: w1494 -> [w1502]
                  tunnel: [w1502] -> w1492
                  tunnel: w1459 -> [w1501]
                  tunnel: [w1508] -> w1491
                  tunnel: w1471 -> [w1507]
                  tunnel: [w1504] -> w1490
                  tunnel: w1493 -> [w1506]
                  tunnel: w1492 -> [w1505]
                  tunnel: w1491 -> [w1511]
                  tunnel: [w1511] -> w1489
                  tunnel: [w1510] -> w1488
                  tunnel: w1490 -> [w1510]
                  tunnel: w1459 -> [w1509]
                  tunnel: w1489 -> [w1516]
                  tunnel: [w1515] -> w1487
                  tunnel: w1468 -> [w1514]
                  tunnel: w1488 -> [w1513]
                  tunnel: [w1512] -> w1486
                  tunnel: w1487 -> [w1519]
                  tunnel: [w1519] -> w1485
                  tunnel: [w1518] -> w1484
                  tunnel: w1486 -> [w1518]
                  tunnel: w1459 -> [w1517]
                  tunnel: w1485 -> [w1524]
                  tunnel: [w1523] -> w1483
                  tunnel: w1465 -> [w1522]
                  tunnel: w1484 -> [w1521]
                  tunnel: [w1520] -> w1482
                  tunnel: [w1527] -> w1481
                  tunnel: w1483 -> [w1527]
                  tunnel: [w1526] -> w1480
                  tunnel: w1482 -> [w1526]
                  tunnel: w1459 -> [w1525]
                  tunnel: w1481 -> [w1534]
                  tunnel: w1480 -> [w1533]
                  tunnel: [w1529] -> w1479
                  tunnel: [w1528] -> w1478
                  tunnel: w1479 -> [w1537]
                  tunnel: [w1537] -> w1477
                  tunnel: w1478 -> [w1536]
                  tunnel: [w1536] -> w1476
                  tunnel: w1459 -> [w1535]
                  tunnel: w1477 -> [w1541]
                  tunnel: w1476 -> [w1540]
                  frame #0 {
                    n829 = VISA Write(VISA resource name=w1500, write buffer=w1496, error in (no error)=w1498) -> (VISA resource name out=w1499:refnum<visa-resource-name>, error out=w1497:errorcluster)  [unwired: 1 out]
                  }
                  frame #1 {
                    n830 = Wait (ms)(milliseconds to wait=w1501) -> ()  [unwired: 1 out]
                  }
                  frame #2 {
                    n831 = VISA Write(VISA resource name=w1506, write buffer=w1507, error in (no error)=w1505) -> (VISA resource name out=w1508:refnum<visa-resource-name>, error out=w1504:errorcluster)  [unwired: 1 out]
                  }
                  frame #3 {
                    n832 = Wait (ms)(milliseconds to wait=w1509) -> ()  [unwired: 1 out]
                  }
                  frame #4 {
                    n833 = VISA Write(VISA resource name=w1516, write buffer=w1514, error in (no error)=w1513) -> (VISA resource name out=w1515:refnum<visa-resource-name>, error out=w1512:errorcluster)  [unwired: 1 out]
                  }
                  frame #5 {
                    n834 = Wait (ms)(milliseconds to wait=w1517) -> ()  [unwired: 1 out]
                  }
                  frame #6 {
                    n835 = VISA Write(VISA resource name=w1524, write buffer=w1522, error in (no error)=w1521) -> (VISA resource name out=w1523:refnum<visa-resource-name>, error out=w1520:errorcluster)  [unwired: 1 out]
                  }
                  frame #7 {
                    n836 = Wait (ms)(milliseconds to wait=w1525) -> ()  [unwired: 1 out]
                  }
                  frame #8 {
                    n837 = Concatenate Strings("start ", "\r") -> (w1532:string)
                    n838 = VISA Write(VISA resource name=w1534, write buffer=w1532, error in (no error)=w1533) -> (VISA resource name out=w1529:refnum<visa-resource-name>, error out=w1528:errorcluster)  [unwired: 1 out]
                  }
                  frame #9 {
                    n839 = Wait (ms)(milliseconds to wait=w1535) -> ()  [unwired: 1 out]
                  }
                  frame #10 {
                    n840 = Concatenate Strings("enter main ", "\r") -> (w1542:string)
                    n841 = VISA Write(VISA resource name=w1541, write buffer=w1542, error in (no error)=w1540) -> (VISA resource name out=w1539:refnum<visa-resource-name>, error out=w1538:errorcluster)  [unwired: 1 out]
                    n842 = VISA Close(VISA resource name=w1539, error in (no error)=w1538) -> ()  [unwired: 1 out]
                  }
                }
                n843 = Concatenate Strings("enter pump1", w1475) -> (w1474:string)
                n844 = local read "Normal \nRate (ul/hr)"() -> (w1460:dbl)
                n845 = Concatenate Strings("set units 4 ", w1475) -> (w1471:string)
                n846 = local read "Normal \nVolume (ul)"() -> (w1461:dbl)
                n847 = Number To Decimal String(number=w1460) -> (decimal integer string=w1470:string)  [unwired: 1 in]
                n848 = Concatenate Strings("set rate ", w1470, w1475) -> (w1468:string)
                n849 = Number To Decimal String(number=w1461) -> (decimal integer string=w1466:string)  [unwired: 1 in]
                n850 = Concatenate Strings("set volume ", w1466, w1475) -> (w1465:string)
              }
            }
          }
          event "Normal \nVolume (ul)": Value Change {
            n851 = event-data() -> ()  [unwired: 1 in, 5 out]
            n852 = call-poly "VISA Configure Serial Port"("VISA resource name"=w1560) -> ("VISA resource name out"=w1562:refnum<visa-resource-name>, "error out"=w1561:errorcluster)  [unwired: 13 in]
            n853 = local read "Write Wait"() -> (w1545:i32)
            n854 = Concatenate Strings("enter pump1", "\r") -> (w1564:string)
            n855 = flat-sequence {
              tunnel: w1561 -> [w1574]
              tunnel: w1562 -> [w1576]
              tunnel: [w1575] -> w1554
              tunnel: [w1573] -> w1553
              tunnel: w1564 -> [w1572]
              tunnel: w1554 -> [w1579]
              tunnel: [w1579] -> w1552
              tunnel: w1553 -> [w1578]
              tunnel: [w1578] -> w1550
              tunnel: w1545 -> [w1577]
              tunnel: w1552 -> [w1583]
              tunnel: [w1584] -> w1551
              tunnel: w1550 -> [w1582]
              tunnel: [w1581] -> w1549
              tunnel: w1546 -> [w1580]
              tunnel: w1551 -> [w1587]
              tunnel: w1549 -> [w1586]
              tunnel: [w1587] -> w1571
              tunnel: [w1586] -> w1570
              tunnel: w1545 -> [w1585]
              tunnel: [w1592] -> w1569
              tunnel: [w1591] -> w1568
              tunnel: w1571 -> [w1590]
              tunnel: w1570 -> [w1589]
              tunnel: w1555 -> [w1588]
              tunnel: w1569 -> [w1595]
              tunnel: [w1595] -> w1567
              tunnel: w1568 -> [w1594]
              tunnel: [w1594] -> w1566
              tunnel: w1545 -> [w1593]
              tunnel: w1567 -> [w1599]
              tunnel: w1566 -> [w1598]
              frame #0 {
                n856 = VISA Write(VISA resource name=w1576, write buffer=w1572, error in (no error)=w1574) -> (VISA resource name out=w1575:refnum<visa-resource-name>, error out=w1573:errorcluster)  [unwired: 1 out]
              }
              frame #1 {
                n857 = Wait (ms)(milliseconds to wait=w1577) -> ()  [unwired: 1 out]
              }
              frame #2 {
                n858 = VISA Write(VISA resource name=w1583, write buffer=w1580, error in (no error)=w1582) -> (VISA resource name out=w1584:refnum<visa-resource-name>, error out=w1581:errorcluster)  [unwired: 1 out]
              }
              frame #3 {
                n859 = Wait (ms)(milliseconds to wait=w1585) -> ()  [unwired: 1 out]
              }
              frame #4 {
                n860 = VISA Write(VISA resource name=w1590, write buffer=w1588, error in (no error)=w1589) -> (VISA resource name out=w1592:refnum<visa-resource-name>, error out=w1591:errorcluster)  [unwired: 1 out]
              }
              frame #5 {
                n861 = Wait (ms)(milliseconds to wait=w1593) -> ()  [unwired: 1 out]
              }
              frame #6 {
                n862 = Concatenate Strings("enter main ", "\r") -> (w1600:string)
                n863 = VISA Write(VISA resource name=w1599, write buffer=w1600, error in (no error)=w1598) -> (VISA resource name out=w1597:refnum<visa-resource-name>, error out=w1596:errorcluster)  [unwired: 1 out]
                n864 = VISA Close(VISA resource name=w1597, error in (no error)=w1596) -> ()  [unwired: 1 out]
              }
            }
            n865 = Concatenate Strings("set units 4", "\r") -> (w1546:string)
            n866 = Number To Decimal String(number="Normal \nVolume (ul)") -> (decimal integer string=w1557:string)  [unwired: 1 in]
            n867 = Concatenate Strings("set volume", w1557, "\r") -> (w1555:string)
          }
          event "Normal \nRate (ul/hr)": Value Change {
            n868 = event-data() -> ()  [unwired: 1 in, 5 out]
            n869 = call-poly "VISA Configure Serial Port"("VISA resource name"=w1605) -> ("VISA resource name out"=w1613:refnum<visa-resource-name>, "error out"=w1612:errorcluster)  [unwired: 13 in]
            n870 = local read "Write Wait"() -> (w1603:i32)
            n871 = Concatenate Strings("enter pump1", "\r") -> (w1615:string)
            n872 = flat-sequence {
              tunnel: w1612 -> [w1632]
              tunnel: w1613 -> [w1634]
              tunnel: [w1633] -> w1628
              tunnel: [w1631] -> w1627
              tunnel: w1615 -> [w1630]
              tunnel: w1628 -> [w1637]
              tunnel: [w1637] -> w1626
              tunnel: w1627 -> [w1636]
              tunnel: [w1636] -> w1625
              tunnel: w1603 -> [w1635]
              tunnel: w1626 -> [w1641]
              tunnel: [w1642] -> w1624
              tunnel: w1625 -> [w1640]
              tunnel: [w1639] -> w1623
              tunnel: w1606 -> [w1638]
              tunnel: w1624 -> [w1645]
              tunnel: w1623 -> [w1644]
              tunnel: [w1645] -> w1622
              tunnel: [w1644] -> w1621
              tunnel: w1603 -> [w1643]
              tunnel: [w1650] -> w1620
              tunnel: [w1649] -> w1619
              tunnel: w1622 -> [w1648]
              tunnel: w1621 -> [w1647]
              tunnel: w1609 -> [w1646]
              tunnel: w1620 -> [w1653]
              tunnel: [w1653] -> w1618
              tunnel: w1619 -> [w1652]
              tunnel: [w1652] -> w1617
              tunnel: w1603 -> [w1651]
              tunnel: w1618 -> [w1657]
              tunnel: w1617 -> [w1656]
              frame #0 {
                n873 = VISA Write(VISA resource name=w1634, write buffer=w1630, error in (no error)=w1632) -> (VISA resource name out=w1633:refnum<visa-resource-name>, error out=w1631:errorcluster)  [unwired: 1 out]
              }
              frame #1 {
                n874 = Wait (ms)(milliseconds to wait=w1635) -> ()  [unwired: 1 out]
              }
              frame #2 {
                n875 = VISA Write(VISA resource name=w1641, write buffer=w1638, error in (no error)=w1640) -> (VISA resource name out=w1642:refnum<visa-resource-name>, error out=w1639:errorcluster)  [unwired: 1 out]
              }
              frame #3 {
                n876 = Wait (ms)(milliseconds to wait=w1643) -> ()  [unwired: 1 out]
              }
              frame #4 {
                n877 = VISA Write(VISA resource name=w1648, write buffer=w1646, error in (no error)=w1647) -> (VISA resource name out=w1650:refnum<visa-resource-name>, error out=w1649:errorcluster)  [unwired: 1 out]
              }
              frame #5 {
                n878 = Wait (ms)(milliseconds to wait=w1651) -> ()  [unwired: 1 out]
              }
              frame #6 {
                n879 = Concatenate Strings("enter main ", "\r") -> (w1658:string)
                n880 = VISA Write(VISA resource name=w1657, write buffer=w1658, error in (no error)=w1656) -> (VISA resource name out=w1655:refnum<visa-resource-name>, error out=w1654:errorcluster)  [unwired: 1 out]
                n881 = VISA Close(VISA resource name=w1655, error in (no error)=w1654) -> ()  [unwired: 1 out]
              }
            }
            n882 = Concatenate Strings("set units 4", "\r") -> (w1606:string)
            n883 = Number To Decimal String(number="Normal \nRate (ul/hr)") -> (decimal integer string=w1604:string)  [unwired: 1 in]
            n884 = Concatenate Strings("set rate", w1604, "\r") -> (w1609:string)
          }
          event "Normal \nRate (ul/hr)  2": Value Change {
            n885 = event-data() -> ()  [unwired: 1 in, 5 out]
            n886 = call-poly "VISA Configure Serial Port"("VISA resource name"=w1663) -> ("VISA resource name out"=w1671:refnum<visa-resource-name>, "error out"=w1670:errorcluster)  [unwired: 13 in]
            n887 = local read "Write Wait"() -> (w1661:i32)
            n888 = Concatenate Strings("enter pump2", "\r") -> (w1673:string)
            n889 = flat-sequence {
              tunnel: w1670 -> [w1690]
              tunnel: w1671 -> [w1692]
              tunnel: [w1691] -> w1686
              tunnel: [w1689] -> w1685
              tunnel: w1673 -> [w1688]
              tunnel: w1686 -> [w1695]
              tunnel: [w1695] -> w1684
              tunnel: w1685 -> [w1694]
              tunnel: [w1694] -> w1683
              tunnel: w1661 -> [w1693]
              tunnel: w1684 -> [w1699]
              tunnel: [w1700] -> w1682
              tunnel: w1683 -> [w1698]
              tunnel: [w1697] -> w1681
              tunnel: w1664 -> [w1696]
              tunnel: w1682 -> [w1703]
              tunnel: w1681 -> [w1702]
              tunnel: [w1703] -> w1680
              tunnel: [w1702] -> w1679
              tunnel: w1661 -> [w1701]
              tunnel: [w1708] -> w1678
              tunnel: [w1707] -> w1677
              tunnel: w1680 -> [w1706]
              tunnel: w1679 -> [w1705]
              tunnel: w1667 -> [w1704]
              tunnel: w1678 -> [w1711]
              tunnel: [w1711] -> w1676
              tunnel: w1677 -> [w1710]
              tunnel: [w1710] -> w1675
              tunnel: w1661 -> [w1709]
              tunnel: w1676 -> [w1715]
              tunnel: w1675 -> [w1714]
              frame #0 {
                n890 = VISA Write(VISA resource name=w1692, write buffer=w1688, error in (no error)=w1690) -> (VISA resource name out=w1691:refnum<visa-resource-name>, error out=w1689:errorcluster)  [unwired: 1 out]
              }
              frame #1 {
                n891 = Wait (ms)(milliseconds to wait=w1693) -> ()  [unwired: 1 out]
              }
              frame #2 {
                n892 = VISA Write(VISA resource name=w1699, write buffer=w1696, error in (no error)=w1698) -> (VISA resource name out=w1700:refnum<visa-resource-name>, error out=w1697:errorcluster)  [unwired: 1 out]
              }
              frame #3 {
                n893 = Wait (ms)(milliseconds to wait=w1701) -> ()  [unwired: 1 out]
              }
              frame #4 {
                n894 = VISA Write(VISA resource name=w1706, write buffer=w1704, error in (no error)=w1705) -> (VISA resource name out=w1708:refnum<visa-resource-name>, error out=w1707:errorcluster)  [unwired: 1 out]
              }
              frame #5 {
                n895 = Wait (ms)(milliseconds to wait=w1709) -> ()  [unwired: 1 out]
              }
              frame #6 {
                n896 = Concatenate Strings("enter main ", "\r") -> (w1716:string)
                n897 = VISA Write(VISA resource name=w1715, write buffer=w1716, error in (no error)=w1714) -> (VISA resource name out=w1713:refnum<visa-resource-name>, error out=w1712:errorcluster)  [unwired: 1 out]
                n898 = VISA Close(VISA resource name=w1713, error in (no error)=w1712) -> ()  [unwired: 1 out]
              }
            }
            n899 = Concatenate Strings("set units 4", "\r") -> (w1664:string)
            n900 = Number To Decimal String(number="Normal \nRate (ul/hr)  2") -> (decimal integer string=w1662:string)  [unwired: 1 in]
            n901 = Concatenate Strings("set rate", w1662, "\r") -> (w1667:string)
          }
          event "Normal \nVolume (ul) 2": Value Change {
            n902 = event-data() -> ()  [unwired: 1 in, 5 out]
            n903 = call-poly "VISA Configure Serial Port"("VISA resource name"=w1722) -> ("VISA resource name out"=w1726:refnum<visa-resource-name>, "error out"=w1727:errorcluster)  [unwired: 13 in]
            n904 = local read "Write Wait"() -> (w1719:i32)
            n905 = Concatenate Strings("enter pump2", "\r") -> (w1724:string)
            n906 = flat-sequence {
              tunnel: w1727 -> [w1748]
              tunnel: w1726 -> [w1750]
              tunnel: [w1749] -> w1745
              tunnel: [w1747] -> w1744
              tunnel: w1724 -> [w1746]
              tunnel: w1745 -> [w1753]
              tunnel: [w1753] -> w1743
              tunnel: w1744 -> [w1752]
              tunnel: [w1752] -> w1742
              tunnel: w1719 -> [w1751]
              tunnel: w1743 -> [w1757]
              tunnel: [w1758] -> w1741
              tunnel: w1742 -> [w1756]
              tunnel: [w1755] -> w1740
              tunnel: w1733 -> [w1754]
              tunnel: w1741 -> [w1761]
              tunnel: w1740 -> [w1760]
              tunnel: [w1761] -> w1739
              tunnel: [w1760] -> w1738
              tunnel: w1719 -> [w1759]
              tunnel: [w1766] -> w1737
              tunnel: [w1765] -> w1736
              tunnel: w1739 -> [w1764]
              tunnel: w1738 -> [w1763]
              tunnel: w1730 -> [w1762]
              tunnel: w1737 -> [w1769]
              tunnel: [w1769] -> w1735
              tunnel: w1736 -> [w1768]
              tunnel: [w1768] -> w1734
              tunnel: w1719 -> [w1767]
              tunnel: w1735 -> [w1773]
              tunnel: w1734 -> [w1772]
              frame #0 {
                n907 = VISA Write(VISA resource name=w1750, write buffer=w1746, error in (no error)=w1748) -> (VISA resource name out=w1749:refnum<visa-resource-name>, error out=w1747:errorcluster)  [unwired: 1 out]
              }
              frame #1 {
                n908 = Wait (ms)(milliseconds to wait=w1751) -> ()  [unwired: 1 out]
              }
              frame #2 {
                n909 = VISA Write(VISA resource name=w1757, write buffer=w1754, error in (no error)=w1756) -> (VISA resource name out=w1758:refnum<visa-resource-name>, error out=w1755:errorcluster)  [unwired: 1 out]
              }
              frame #3 {
                n910 = Wait (ms)(milliseconds to wait=w1759) -> ()  [unwired: 1 out]
              }
              frame #4 {
                n911 = VISA Write(VISA resource name=w1764, write buffer=w1762, error in (no error)=w1763) -> (VISA resource name out=w1766:refnum<visa-resource-name>, error out=w1765:errorcluster)  [unwired: 1 out]
              }
              frame #5 {
                n912 = Wait (ms)(milliseconds to wait=w1767) -> ()  [unwired: 1 out]
              }
              frame #6 {
                n913 = Concatenate Strings("enter main ", "\r") -> (w1774:string)
                n914 = VISA Write(VISA resource name=w1773, write buffer=w1774, error in (no error)=w1772) -> (VISA resource name out=w1771:refnum<visa-resource-name>, error out=w1770:errorcluster)  [unwired: 1 out]
                n915 = VISA Close(VISA resource name=w1771, error in (no error)=w1770) -> ()  [unwired: 1 out]
              }
            }
            n916 = Concatenate Strings("set units 4", "\r") -> (w1733:string)
            n917 = Number To Decimal String(number="Normal \nVolume (ul) 2") -> (decimal integer string=w1720:string)  [unwired: 1 in]
            n918 = Concatenate Strings("set volume", w1720, "\r") -> (w1730:string)
          }
        }
        n919 = node-c288() -> ()  [unwired: 1 in, 1 out]
      }
      n920 = node-c288(w1106) -> ()  [unwired: 1 out]
    }
    frame Enabled {
      n921 = node-c288(2 ("Processor")) -> (w1786:T12)  [unwired: 3 in]
      n922 = timed-loop "Pump Control" {
        timing: w1786 -> [_]
        timing-out: [_] -> w1785
        tunnel: refnum<visa-resource-name> "COM5" ("VISA resource name") -> [w1788]
        stop <- w1787 stop-if-true
        n923 = node-c288() -> ()  [unwired: 1 in, 1 out]
        n924 = event shown="[2] \"Inject Sample\": Value Change" {
          selector: _ -> [_ _ _ _ _]
          dyn-events: _ -> [_ _ _ _ _]
          timeout: _ -> [_ _ _ _ _]
          tunnel: w1788 -> [w1794 _ w1868 w1895 w1900]
          tunnel: [_ w1866 _ _ _] -> w1787
          event "Flush Sample": Value Change {
            n925 = event-data() -> ()  [unwired: 1 in, 5 out]
            n926 = local read "Write Wait"() -> (w1808:i32)
            n927 = flat-sequence {
              tunnel: [w1832] -> w1828
              tunnel: [w1831] -> w1827
              tunnel: "CLD" -> [w1830]
              tunnel: w1794 -> [w1829]
              tunnel: w1828 -> [w1835]
              tunnel: [w1835] -> w1826
              tunnel: w1827 -> [w1834]
              tunnel: [w1834] -> w1825
              tunnel: w1808 -> [w1833]
              tunnel: [w1840] -> w1824
              tunnel: [w1837] -> w1823
              tunnel: w1826 -> [w1839]
              tunnel: w1825 -> [w1838]
              tunnel: "MODVOL" -> [w1836]
              tunnel: w1824 -> [w1843]
              tunnel: [w1843] -> w1822
              tunnel: [w1842] -> w1821
              tunnel: w1823 -> [w1842]
              tunnel: w1808 -> [w1841]
              tunnel: w1822 -> [w1848]
              tunnel: [w1847] -> w1820
              tunnel: w1810 -> [w1846]
              tunnel: w1821 -> [w1845]
              tunnel: [w1844] -> w1819
              tunnel: w1820 -> [w1851]
              tunnel: [w1851] -> w1818
              tunnel: [w1850] -> w1817
              tunnel: w1819 -> [w1850]
              tunnel: w1808 -> [w1849]
              tunnel: w1818 -> [w1856]
              tunnel: [w1855] -> w1816
              tunnel: w1812 -> [w1854]
              tunnel: w1817 -> [w1853]
              tunnel: [w1852] -> w1815
              tunnel: [w1859] -> w1813
              tunnel: w1816 -> [w1859]
              tunnel: [w1858] -> w1814
              tunnel: w1815 -> [w1858]
              tunnel: w1808 -> [w1857]
              tunnel: w1814 -> [w1864]
              tunnel: w1813 -> [w1865]
              tunnel: [w1863] -> w1803
              tunnel: "RUN " -> [w1862]
              frame #0 {
                n928 = call "Write to pump 2.vi"("String to write"=w1830, "VISA resource name"=w1829) -> ("error out"=w1831:errorcluster, "VISA resource name out"=w1832:refnum<visa-resource-name>)  [unwired: 8 in]
              }
              frame #1 {
                n929 = Wait (ms)(milliseconds to wait=w1833) -> ()  [unwired: 1 out]
              }
              frame #2 {
                n930 = call "Write to pump 2.vi"("error in (no error)"=w1838, "String to write"=w1836, "VISA resource name"=w1839) -> ("error out"=w1837:errorcluster, "VISA resource name out"=w1840:refnum<visa-resource-name>)  [unwired: 7 in]
              }
              frame #3 {
                n931 = Wait (ms)(milliseconds to wait=w1841) -> ()  [unwired: 1 out]
              }
              frame #4 {
                n932 = call "Write to pump 2.vi"("error in (no error)"=w1845, "String to write"=w1846, "VISA resource name"=w1848) -> ("error out"=w1844:errorcluster, "VISA resource name out"=w1847:refnum<visa-resource-name>)  [unwired: 7 in]
              }
              frame #5 {
                n933 = Wait (ms)(milliseconds to wait=w1849) -> ()  [unwired: 1 out]
              }
              frame #6 {
                n934 = call "Write to pump 2.vi"("error in (no error)"=w1853, "String to write"=w1854, "VISA resource name"=w1856) -> ("error out"=w1852:errorcluster, "VISA resource name out"=w1855:refnum<visa-resource-name>)  [unwired: 7 in]
              }
              frame #7 {
                n935 = Wait (ms)(milliseconds to wait=w1857) -> ()  [unwired: 1 out]
              }
              frame #8 {
                w1861 = TRUE ("Inject Pump 3")
                n936 = Tick Count (ms)() -> (millisecond timer value=→"Flush Sample Start Time":u32)
                n937 = call "Write to pump 2.vi"("error in (no error)"=w1864, "String to write"=w1862, "VISA resource name"=w1865) -> ("error out"=w1863:errorcluster)  [unwired: 7 in, 1 out]
                n938 = local write "Inject Sample"(w1861) -> ()
                "Flushing Sample" <- w1861
              }
            }
            n939 = Number To Fractional String(number="Flush \nRate (ul/min)  3") -> (F-format string=w1796:string)  [unwired: 3 in]
            n940 = String Subset(string=w1796, length (rest)=6 ("length (rest)")) -> (substring=w1795:string)  [unwired: 1 in]
            n941 = Concatenate Strings("RAT", w1795, "UM") -> (w1810:string)
            n942 = Divide(x="Flush\nVolume (ul)  3", y=1000.0) -> (x/y=w1801:dbl)
            n943 = Number To Fractional String(number=w1801) -> (F-format string=w1800:string)  [unwired: 3 in]
            n944 = Divide(x="Flush\nVolume (ul)  3", y="Flush \nRate (ul/min)  3") -> (x/y=w1791:dbl)
            n945 = Multiply(x=w1791, y=60.0) -> (x*y=→"Sample flush time (s)":dbl)
            n946 = String Subset(string=w1800, length (rest)=6 ("length (rest)")) -> (substring=w1799:string)  [unwired: 1 in]
            n947 = Concatenate Strings("TGT", w1799) -> (w1812:string)
            "error out" <- w1803
          }
          event "Stop": Value Change {
            n948 = event-data() -> ()  [unwired: 1 in, 5 out]
            n949 = local read "Stop"() -> (w1866:bool)
          }
          event "Inject Sample": Value Change {
            n950 = event-data() -> ()  [unwired: 1 in, 5 out]
            n951 = case shown="True" "Inject Sample" {
              tunnel: w1868 -> [w1870 w1871]
              frame False {
                n952 = call "Write to pump 2.vi"("String to write"="STP", "VISA resource name"=w1870) -> ()  [unwired: 8 in, 2 out]
              }
              frame True {
                n953 = local read "Normal \nRate (ul/hr)  3"() -> (w1872:dbl)
                n954 = Number To Fractional String(number=w1872) -> (F-format string=w1875:string)  [unwired: 3 in]
                n955 = String Subset(string=w1875, length (rest)=6 ("length (rest)")) -> (substring=w1873:string)  [unwired: 1 in]
                n956 = flat-sequence {
                  tunnel: "RUN " -> [w1887]
                  tunnel: [w1889] -> _
                  tunnel: [w1888] -> _
                  tunnel: w1871 -> [w1886]
                  frame #0 {
                    n957 = call "Write to pump 2.vi"("String to write"=w1887, "VISA resource name"=w1886) -> ("error out"=w1888:errorcluster, "VISA resource name out"=w1889:refnum<visa-resource-name>)  [unwired: 8 in]
                  }
                }
                n958 = Concatenate Strings("RAT", w1873, "UH" ("string")) -> ()  [unwired: 1 out]
                n959 = local read "Normal \nVolume (ul) 3"() -> (w1881:dbl)
                n960 = Divide(x=w1881, y=1000.0) -> (x/y=w1876:dbl)
                n961 = Number To Fractional String(number=w1876) -> (F-format string=w1879:string)  [unwired: 3 in]
                n962 = String Subset(string=w1879, length (rest)=6 ("length (rest)")) -> (substring=w1877:string)  [unwired: 1 in]
                n963 = Concatenate Strings("TGT", w1877) -> ()  [unwired: 1 out]
              }
            }
          }
          event "Normal \nRate (ul/hr)  3": Value Change {
            n964 = event-data() -> ()  [unwired: 1 in, 5 out]
            n965 = Number To Fractional String(number="Normal \nRate (ul/hr)  3") -> (F-format string=w1893:string)  [unwired: 3 in]
            n966 = String Subset(string=w1893, length (rest)=6 ("length (rest)")) -> (substring=w1891:string)  [unwired: 1 in]
            n967 = Concatenate Strings("RAT", w1891, "UH") -> (w1894:string)
            n968 = call "Write to pump 2.vi"("String to write"=w1894, "VISA resource name"=w1895) -> ()  [unwired: 8 in, 2 out]
          }
          event "Clear Volume": Value Change {
            n969 = event-data() -> ()  [unwired: 1 in, 5 out]
            n970 = Divide(x="Normal \nVolume (ul) 3", y=1000.0) -> (x/y=w1913:dbl)
            n971 = Number To Fractional String(number=w1913) -> (F-format string=w1916:string)  [unwired: 3 in]
            n972 = String Subset(string=w1916, length (rest)=6 ("length (rest)")) -> (substring=w1914:string)  [unwired: 1 in]
            n973 = flat-sequence {
              tunnel: [w1923] -> w1911
              tunnel: [w1922] -> w1910
              tunnel: w1900 -> [w1921]
              tunnel: w1899 -> [w1920]
              tunnel: [w1925] -> w1908
              tunnel: [w1924] -> w1909
              tunnel: w1905 -> [w1926]
              tunnel: w1911 -> [w1925]
              tunnel: w1910 -> [w1924]
              tunnel: w1909 -> [w1930]
              tunnel: w1908 -> [w1931]
              tunnel: [w1929] -> _
              tunnel: [w1928] -> _
              tunnel: w1898 -> [w1927]
              frame #0 {
                n974 = call "Write to pump 2.vi"("String to write"=w1920, "VISA resource name"=w1921) -> ("error out"=w1922:errorcluster, "VISA resource name out"=w1923:refnum<visa-resource-name>)  [unwired: 8 in]
              }
              frame #1 {
                n975 = Wait (ms)(milliseconds to wait=w1926) -> ()  [unwired: 1 out]
              }
              frame #2 {
                n976 = call "Write to pump 2.vi"("error in (no error)"=w1930, "String to write"=w1927, "VISA resource name"=w1931) -> ("error out"=w1928:errorcluster, "VISA resource name out"=w1929:refnum<visa-resource-name>)  [unwired: 7 in]
              }
            }
            n977 = local read "Write Wait"() -> (w1905:i32)
            n978 = Concatenate Strings("TGT", w1914) -> (w1899:string)
            n979 = local read "Normal \nRate (ul/hr)  3"() -> (w1901:dbl)
            n980 = local write "Clear Volume"(FALSE ("Clear Volume")) -> ()
            n981 = Number To Fractional String(number=w1901) -> (F-format string=w1904:string)  [unwired: 3 in]
            n982 = String Subset(string=w1904, length (rest)=6 ("length (rest)")) -> (substring=w1902:string)  [unwired: 1 in]
            n983 = Concatenate Strings("RAT", w1902, "UH" ("string")) -> (w1898:string)
          }
        }
        n984 = node-c288() -> ()  [unwired: 1 in, 1 out]
      }
      n985 = node-c288(w1785) -> ()  [unwired: 1 out]
    }
  }
  n986 = local write "Tether"(FALSE ("Tether")) -> ()
  n987 = local read "Path"() -> (w81:path)
  n988 = node-c288(i64 50 ("Period"), 2 ("Processor")) -> (w87:T12)  [unwired: 2 in]
  n989 = VISA Close(VISA resource name=w19) -> (error out=w104:errorcluster)  [unwired: 1 in]
  n990 = timed-loop {
    timing: w87 -> [_]
    timing-out: [_] -> w86
    tunnel: w81 -> [w1939]
    stop <- w1938 stop-if-true
    n991 = node-c288() -> ()  [unwired: 1 in, 1 out]
    n992 = event shown="[5] \"Raster scan\": Value Change" {
      selector: _ -> [_ _ _ _ _ _ _ _ _]
      dyn-events: _ -> [_ _ _ _ _ _ _ _ _]
      timeout: _ -> [_ _ _ _ _ _ _ _ _]
      tunnel: w1939 -> [_ w1943 _ _ _ _ _ _ _]
      tunnel: [_ _ w1963 _ _ _ _ _ _] -> w1938
      event Timeout {
        n993 = event-data() -> ()  [unwired: 1 in, 2 out]
      }
      event "Read Cal": Value Change {
        n994 = event-data() -> ()  [unwired: 1 in, 6 out]
        n995 = Path To String(path=w1943) -> (string=w1942:string)
        n996 = Format Date/Time String(time format string (%c)="%y%m%d") -> (date/time string=w1944:string)  [unwired: 2 in]
        n997 = Concatenate Strings(w1942, "\\" ("string"), w1944, "\\" ("string"), "current.cal") -> (w1962:string)
        n998 = String To Path(string=w1962) -> (path=w1961:path)
        n999 = Open/Create/Replace File(file path (use dialog)=w1961, operation (0:open)=T9."open", access (0:read/write)=enum16{"read/write", "read-only", "write-only"}."read-only") -> (refnum out=w1957:refnum<file>, error out=w1958:errorcluster)  [unwired: 3 in, 1 out]
        n1000 = Deny Access(4:w1958, 7:w1957) -> (0:w1956:errorcluster, 3:w1955:refnum<file>)  [unwired: 1 in]
        n1001 = Read from Binary File(5:0.0, 8:w1956, 9:T10."big-endian, network order" ("byte order (0:big-endian, network order)"), 10:12 ("count"), 11:w1955) -> (0:w1951:errorcluster, 2:w1949:dbl[], 3:w1952:refnum<file>)  [unwired: 1 in, 1 out]
        n1002 = Array To Cluster(array=w1949) -> (cluster=→"Cal values":T17)
        n1003 = Close File(refnum=w1952, error in=w1951) -> ()  [unwired: 2 out]
        n1004 = local write "Read Cal"(FALSE ("Read Cal")) -> ()
      }
      event "Stop": Value Change {
        n1005 = event-data() -> ("NewVal"=w1963:bool)  [unwired: 1 in, 5 out]
      }
      event "Trap position": Value Change {
        # "Need to rotate so X and Y don't get mixed up."
        n1006 = event-data() -> ()  [unwired: 1 in, 6 out]
        n1007 = local read "Mirror task"() -> (w1964:refnum<k21>)
        n1008 = Cluster To Array(cluster="Trap position") -> (array=w1967:dbl[])
        n1009 = Rotate 1D Array(1:w1967, 2:1 ("n")) -> (0:w1965:dbl[])
        n1010 = call-poly <vilib>:"DAQmx Write.vi"("task/channels in"=w1964, "data"=w1965) -> ("task out"=w1970:refnum<k21>, "error out"=w1969:errorcluster)  [unwired: 11 in, 1 out]
        n1011 = call <vilib>:"DAQmx Stop Task.vi"("task/channels in"=w1970, "error in"=w1969) -> ("error out"=w1968:errorcluster)  [unwired: 12 in, 1 out]
        n1012 = call <vilib>:"Simple Error Handler.vi"("error in (no error)"=w1968) -> ()  [unwired: 4 in, 5 out]
      }
      event "Trap delta": Value Change {
        n1013 = event-data() -> ()  [unwired: 1 in, 6 out]
        n1014 = local read "Pulling direction"() -> (w1973:bool)
        n1015 = local read "Fixed Y"() -> (w1977:dbl)
        n1016 = local read "Fixed X"() -> (w1976:dbl)
        n1017 = Select(t=w1977, s=w1973, f=w1976) -> (s? t:f=w1975:dbl)
        n1018 = Add(x="Trap delta", y=w1975) -> (x+y=w1972:dbl)
        n1019 = case shown="True" w1973 {
          tunnel: w1972 -> [w1978 w1979]
          frame False {
            n1020 = property on="X" class="DigNum (strict)"("Val(Sgnl)"=w1978) -> ()  [unwired: 2 in, 2 out]
          }
          frame True {
            n1021 = property on="Y" class="DigNum (strict)"("Val(Sgnl)"=w1979) -> ()  [unwired: 2 in, 2 out]
          }
        }
      }
      event "Raster scan": Value Change {
        w2012 = T15 1 items=["no dialog", "OK message", "continue or stop message", "OK message + warnings", "continue/stop + warnings"] ("type of dialog (OK msg:1)")
        w1996 = 0.0 ("minimum value")
        w1995 = 10.0 ("maximum value")
        # "Grab offset in pulling\ndirection and add to \ndelta values"
        # "Send offset in direction\nof not-pulling to DAQ"
        n1022 = event-data() -> ()  [unwired: 1 in, 6 out]
        n1023 = local read "Min delta"() -> (w2001:dbl)
        n1024 = local read "Max delta"() -> (w1998:dbl)
        n1025 = call-poly <vilib>:"DAQmx Create Virtual Channel.vi"("maximum value"=w1995, "minimum value"=w1996, "physical channels"=tag "Dev1/ao0") -> ("task out"=w2017:refnum<k21>, "error out"=w2016:errorcluster)  [unwired: 11 in]
        n1026 = local read "Fixed Y"() -> (w2005:dbl)
        n1027 = local read "Fixed X"() -> (w2006:dbl)
        n1028 = local read "Conv Y (nm/V)"() -> (w1991:dbl)
        n1029 = local read "Conv X (nm/V)"() -> (w1993:dbl)
        n1030 = local read "Speed (ms)"() -> (w1983:i32)
        n1031 = Subtract(x=w1998, y=w2001) -> (x-y=w1989:dbl)
        n1032 = Divide(x=w1983, y=2) -> (x/y=w1981:dbl)
        n1033 = Select(t=w2006, s="Pulling direction", f=w2005) -> (s? t:f=w2008:dbl)
        n1034 = Select(t=w2005, s="Pulling direction", f=w2006) -> (s? t:f=w2002:dbl)
        n1035 = Select(t=w1991, s="Pulling direction", f=w1993) -> (s? t:f=w1990:dbl)
        n1036 = Divide(x=w1989, y=w1981) -> (x/y=w1988:dbl)
        n1037 = call-poly <vilib>:"DAQmx Create Virtual Channel.vi"("task in"=w2017, "maximum value"=w1995, "minimum value"=w1996, "physical channels"=tag "Dev1/ao1", "error in"=w2016) -> ("task out"=w2011:refnum<k21>, "error out"=w2010:errorcluster)  [unwired: 9 in]
        n1038 = Multiply(x=w1989, y=w1990) -> (x*y=w1986:dbl)
        "Scan Range (nm)" <- w1986
        n1039 = Add(x=w2002, y=w1998) -> (x+y=w2004:dbl)
        n1040 = Divide(x=w1981, y=1000) -> (x/y=w1985:dbl)
        n1041 = Add(x=w2002, y=w2001) -> (x+y=w2003:dbl)
        n1042 = Divide(x=w1986, y=w1985) -> (x/y=→"Scan Speed (nm/s)":dbl)
        n1043 = node-c288(i64 1 ("Period")) -> (w2021:T12)  [unwired: 3 in]
        n1044 = timed-loop {
          tunnel: "Pulling direction" -> [w2041]
          tunnel: w1988 -> [w2037]
          tunnel: w2003 -> [w2040]
          tunnel: w2008 -> [w2029]
          tunnel: w2011 -> [w2039]
          tunnel: w2010 -> [w2038]
          tunnel: w2004 -> [w2036]
          tunnel: [w2033] -> w2015
          tunnel: [w2032] -> w2014
          tunnel: [w2027] -> w2000
          timing: w2021 -> [_]
          timing-out: [_] -> w2020
          tunnel: w1981 -> [w2028]
          tunnel: "Trap delta\nafter" -> [w2024]
          tunnel: [w2024] -> w2007
          i -> [w2031]
          stop <- w2027 stop-if-true
          n1045 = node-c288() -> ()  [unwired: 1 in, 1 out]
          n1046 = flat-sequence {
            tunnel: [w2050] -> w2035
            tunnel: [w2049] -> w2034
            tunnel: w2041 -> [w2048]
            tunnel: w2037 -> [w2055]
            tunnel: w2040 -> [w2054]
            tunnel: w2029 -> [w2053]
            tunnel: w2039 -> [w2052]
            tunnel: w2038 -> [w2051]
            tunnel: w2028 -> [w2047]
            tunnel: w2037 -> [w2086]
            tunnel: w2036 -> [w2085]
            tunnel: w2035 -> [w2092]
            tunnel: w2034 -> [w2091]
            tunnel: [w2090] -> w2033
            tunnel: [w2089] -> w2032
            tunnel: w2029 -> [w2087]
            frame #0 {
              n1047 = node-c288(i64 1 ("Period")) -> (w2046:T12)  [unwired: 3 in]
              n1048 = timed-loop {
                tunnel: w2055 -> [w2075]
                tunnel: w2054 -> [w2073]
                tunnel: w2053 -> [w2058]
                tunnel: w2052 -> [w2072]
                tunnel: w2051 -> [w2071]
                tunnel: [w2065] -> w2050
                tunnel: [w2066] -> w2049
                tunnel: w2048 -> [w2069]
                tunnel: w2047 -> [w2067]
                timing: w2046 -> [_]
                timing-out: [_] -> w2045
                i -> [w2063]
                stop <- w2068 stop-if-true
                n1049 = node-c288() -> ()  [unwired: 1 in, 1 out]
                n1050 = Multiply(x=w2075, y=w2063) -> (x*y=w2074:dbl)
                n1051 = Add(x=w2073, y=w2074) -> (x+y=w2059:dbl)
                n1052 = local read "Stop saving"() -> (w2056:bool)
                n1053 = local read "Stop raster"() -> (w2057:bool)
                n1054 = Build Array(w2058, w2059) -> (w2060:dbl[])
                n1055 = Build Array(w2059, w2058) -> (w2062:dbl[])
                n1056 = Greater Or Equal?(x=w2063, y=w2067) -> (x >= y?=w2064:bool)
                n1057 = Select(t=w2060, s=w2069, f=w2062) -> (s? t:f=w2061:dbl[])
                n1058 = Compound Arithmetic op=OR(w2064, w2057, w2056) -> (w2068:bool)
                n1059 = call-poly <vilib>:"DAQmx Write.vi"("task/channels in"=w2072, "auto start"=TRUE, "data"=w2061, "error in"=w2071) -> ("task out"=w2065:refnum<k21>, "error out"=w2066:errorcluster)  [unwired: 9 in, 1 out]
                n1060 = node-c288() -> ()  [unwired: 1 in, 1 out]
              }
              n1061 = node-c288(w2045) -> ()  [unwired: 1 out]
            }
            frame #1 {
              n1062 = local read "Pulling direction"() -> (w2088:bool)
              n1063 = node-c288(i64 1 ("Period")) -> (w2084:T12)  [unwired: 3 in]
              n1064 = timed-loop {
                tunnel: w2086 -> [w2103]
                tunnel: w2085 -> [w2106]
                tunnel: w2087 -> [w2097]
                tunnel: w2092 -> [w2115]
                tunnel: w2091 -> [w2107]
                tunnel: [w2099] -> w2090
                tunnel: [w2109] -> w2089
                tunnel: w2088 -> [w2111]
                timing: w2084 -> [_]
                timing-out: [_] -> w2083
                i -> [w2104]
                stop <- w2105 stop-if-true
                n1065 = node-c288() -> ()  [unwired: 1 in, 1 out]
                n1066 = Multiply(x=w2103, y=w2104) -> (x*y=w2102:dbl)
                n1067 = Subtract(x=w2106, y=w2102) -> (x-y=w2101:dbl)
                n1068 = Build Array(w2097, w2101) -> (w2110:dbl[])
                n1069 = local read "Speed (ms)"() -> (w2094:i32)
                n1070 = Build Array(w2101, w2097) -> (w2100:dbl[])
                n1071 = Select(t=w2110, s=w2111, f=w2100) -> (s? t:f=w2098:dbl[])
                n1072 = Divide(x=w2094, y=2) -> (x/y=w2093:dbl)
                n1073 = local read "Stop raster"() -> (w2113:bool)
                n1074 = local read "Stop saving"() -> (w2096:bool)
                n1075 = Decrement(x=w2093) -> (x-1=w2108:dbl)
                n1076 = call-poly <vilib>:"DAQmx Write.vi"("task/channels in"=w2115, "auto start"=TRUE, "data"=w2098, "error in"=w2107) -> ("task out"=w2099:refnum<k21>, "error out"=w2109:errorcluster)  [unwired: 9 in, 1 out]
                n1077 = Greater Or Equal?(x=w2104, y=w2108) -> (x >= y?=w2114:bool)
                n1078 = node-c288() -> ()  [unwired: 1 in, 1 out]
                n1079 = Compound Arithmetic op=OR(w2114, w2113, w2096) -> (w2105:bool)
              }
              n1080 = node-c288(w2083) -> ()  [unwired: 1 out]
            }
          }
          n1081 = local read "# scans"() -> (w2023:i32)
          n1082 = local read "Stop saving"() -> (w2022:bool)
          n1083 = Decrement(x=w2023) -> (x-1=w2025:i32)
          n1084 = Greater Or Equal?(x=w2031, y=w2025) -> (x >= y?=w2030:bool)
          n1085 = Compound Arithmetic op=OR(w2030, "Stop raster", w2022) -> (w2027:bool)
          n1086 = node-c288() -> ()  [unwired: 1 in, 1 out]
        }
        n1087 = node-c288(w2020) -> ()  [unwired: 1 out]
        n1088 = call <vilib>:"DAQmx Clear Task.vi"("task in"=w2015, "error in"=w2014) -> ("error out"=w2013:errorcluster)  [unwired: 13 in]
        n1089 = Not(x=w2000) -> (.not. x?=w2009:bool)
        n1090 = Not(x=w2000) -> (.not. x?=w1999:bool)
        n1091 = property on="Trap delta" class="DigNum (strict)"("Val(Sgnl)"=w2007) -> ()  [unwired: 2 in, 2 out]
        n1092 = call <vilib>:"Simple Error Handler.vi"("type of dialog (OK msg:1)"=w2012, "error in (no error)"=w2013) -> ()  [unwired: 3 in, 5 out]
        n1093 = local write "Stop raster"(w2009) -> ()
        n1094 = property on="Stop saving" class="Bool (strict)"("Val(Sgnl)"=w2000) -> ()  [unwired: 2 in, 2 out]
        n1095 = local write "Raster scanning..."(w1999) -> ()
        "Raster scanning..." <- TRUE ("Raster scanning...")
      }
      event "Fish": Value Change {
        n1096 = event-data() -> ()  [unwired: 1 in, 6 out]
        n1097 = local read "Fish"() -> (w2126:bool)
        n1098 = case shown="True" w2126 {
          frame False {
          }
          frame True {
            w2135 = 0.0 ("minimum value")
            w2136 = 10.0 ("maximum value")
            # "Grab offset in pulling\ndirection and add to \ndelta values"
            n1099 = call-poly <vilib>:"DAQmx Create Virtual Channel.vi"("maximum value"=w2136, "minimum value"=w2135, "physical channels"=tag "Dev1/ao0") -> ("task out"=w2140:refnum<k21>, "error out"=w2139:errorcluster)  [unwired: 11 in]
            n1100 = call-poly <vilib>:"DAQmx Create Virtual Channel.vi"("task in"=w2140, "maximum value"=w2136, "minimum value"=w2135, "physical channels"=tag "Dev1/ao1", "error in"=w2139) -> ("task out"=w2134:refnum<k21>, "error out"=w2133:errorcluster)  [unwired: 9 in]
            n1101 = node-c288(i64 1 ("Period")) -> (w2142:T12)  [unwired: 3 in]
            n1102 = timed-loop {
              timing: w2142 -> [_]
              timing-out: [_] -> w2141
              tunnel: w2134 -> [w2191]
              tunnel: w2133 -> [w2190]
              tunnel: [w2189] -> w2129
              tunnel: [w2188] -> w2128
              tunnel: [w2156] -> w2131
              tunnel: [w2170] -> w2127
              i -> [w2174]
              stop <- w2170 stop-if-true
              # "Send offset in direction\nof not-pulling to DAQ"
              n1103 = node-c288() -> ()  [unwired: 1 in, 1 out]
              n1104 = local read "Pulling direction"() -> (w2158:bool)
              n1105 = local read "Fixed Y"() -> (w2160:dbl)
              n1106 = local read "Fixed X"() -> (w2161:dbl)
              n1107 = Select(t=w2160, s=w2158, f=w2161) -> (s? t:f=w2162:dbl)
              n1108 = Add(x=w2162, y="Max fish\ndelta (V)") -> (x+y=w2164:dbl)
              n1109 = Subtract(x="Max fish\ndelta (V)", y="Min fish\ndelta (V)") -> (x-y=w2166:dbl)
              n1110 = Select(t=w2161, s=w2158, f=w2160) -> (s? t:f=w2159:dbl)
              n1111 = Divide(x=w2166, y="Fish Speed (ms)") -> (x/y=w2167:dbl)
              n1112 = flat-sequence {
                tunnel: w2158 -> [w2210]
                tunnel: w2159 -> [w2209]
                tunnel: w2191 -> [w2208]
                tunnel: w2190 -> [w2207]
                tunnel: w2167 -> [w2206]
                tunnel: w2164 -> [w2205]
                tunnel: "Fish Speed (ms)" -> [w2200]
                tunnel: [w2204] -> w2187
                tunnel: [w2203] -> w2186
                tunnel: [w2202] -> w2185
                tunnel: [w2201] -> w2184
                tunnel: [w2194] -> w2173
                tunnel: [w2193] -> w2157
                tunnel: [w2192] -> w2154
                tunnel: [w2257] -> w2183
                tunnel: w2187 -> [w2257]
                tunnel: [w2256] -> w2182
                tunnel: w2186 -> [w2256]
                tunnel: [w2255] -> w2181
                tunnel: w2185 -> [w2255]
                tunnel: [w2254] -> w2180
                tunnel: w2184 -> [w2254]
                tunnel: w2173 -> [w2253]
                tunnel: [w2253] -> w2172
                tunnel: w2157 -> [w2252]
                tunnel: [w2251] -> w2155
                tunnel: w2154 -> [w2251]
                tunnel: w2183 -> [w2268]
                tunnel: w2182 -> [w2267]
                tunnel: w2181 -> [w2266]
                tunnel: w2180 -> [w2265]
                tunnel: w2169 -> [w2264]
                tunnel: [w2263] -> w2189
                tunnel: [w2262] -> w2188
                tunnel: w2172 -> [w2261]
                tunnel: [w2260] -> w2156
                tunnel: w2155 -> [w2259]
                frame #0 {
                  n1113 = local read "Mean force (pN)"() -> (w2199:dbl)
                  n1114 = local read "Cutoff force (pN)"() -> (w2198:dbl)
                  n1115 = Less Or Equal?(x=w2199, y=w2198) -> (x <= y?=w2196:bool)
                  n1116 = And(x="Fish", y=w2196) -> (x .and. y?=w2197:bool)
                  n1117 = case shown="True" w2197 {
                    selector: w2197 -> [w2212 _]
                    tunnel: w2210 -> [w2215 w2231]
                    tunnel: w2209 -> [_ w2230]
                    tunnel: w2208 -> [w2217 w2229]
                    tunnel: w2207 -> [w2216 w2228]
                    tunnel: w2206 -> [w2214 w2227]
                    tunnel: w2205 -> [w2213 w2226]
                    tunnel: [w2217 w2225] -> w2204
                    tunnel: [w2216 w2224] -> w2203
                    tunnel: [w2215 w2223] -> w2202
                    tunnel: [w2213 w2222] -> w2192
                    tunnel: [w2214 w2221] -> w2201
                    tunnel: w2200 -> [_ w2220]
                    tunnel: [w2212 w2219] -> w2194
                    tunnel: [FALSE w2218] -> w2193
                    frame False {
                    }
                    frame True {
                      n1118 = while {
                        tunnel: w2231 -> [w2240]
                        tunnel: w2230 -> [w2239]
                        tunnel: w2229 -> [w2247]
                        tunnel: w2228 -> [w2246]
                        tunnel: w2227 -> [w2238]
                        tunnel: w2226 -> [w2244]
                        tunnel: [w2242] -> w2225
                        tunnel: [w2241] -> w2224
                        tunnel: [w2240] -> w2223
                        tunnel: [w2239] -> w2222
                        tunnel: [w2238] -> w2221
                        tunnel: w2220 -> [w2237]
                        tunnel: [w2232] -> w2219
                        tunnel: [w2232] -> w2218
                        i -> [w2236]
                        stop <- w2233 stop-if-true
                        n1119 = Multiply(x=w2238, y=w2236) -> (x*y=w2245:dbl)
                        n1120 = Subtract(x=w2244, y=w2245) -> (x-y=w2243:dbl)
                        n1121 = Build Array(w2239, w2243) -> (w2250:dbl[])
                        n1122 = Build Array(w2243, w2239) -> (w2249:dbl[])
                        n1123 = Greater Or Equal?(x=w2236, y=w2237) -> (x >= y?=w2232:bool)
                        n1124 = Select(t=w2250, s=w2240, f=w2249) -> (s? t:f=w2248:dbl[])
                        n1125 = local read "Fish"() -> (w2234:bool)
                        n1126 = Not(x=w2234) -> (.not. x?=w2235:bool)
                        n1127 = call-poly <vilib>:"DAQmx Write.vi"("task/channels in"=w2247, "data"=w2248, "error in"=w2246) -> ("task out"=w2242:refnum<k21>, "error out"=w2241:errorcluster)  [unwired: 10 in, 1 out]
                        n1128 = Compound Arithmetic op=OR(w2232, w2235) -> (w2233:bool)
                      }
                    }
                  }
                }
                frame #1 {
                  n1129 = case shown="True" w2252 {
                    frame False {
                    }
                    frame True {
                      n1130 = Wait (ms)(milliseconds to wait="Wait (ms)") -> ()  [unwired: 1 out]
                    }
                  }
                }
                frame #2 {
                  n1131 = case shown="True" w2261 {
                    tunnel: w2268 -> [w2271 w2280]
                    tunnel: w2267 -> [w2270 w2279]
                    tunnel: w2266 -> [_ w2278]
                    tunnel: w2265 -> [_ w2277]
                    tunnel: w2264 -> [_ w2276]
                    tunnel: [w2271 w2275] -> w2263
                    tunnel: [w2270 w2274] -> w2262
                    tunnel: [FALSE w2273] -> w2260
                    tunnel: w2259 -> [_ w2272]
                    frame False {
                    }
                    frame True {
                      n1132 = while {
                        tunnel: w2280 -> [w2308]
                        tunnel: w2279 -> [w2307]
                        tunnel: w2278 -> [w2290]
                        tunnel: w2277 -> [w2305]
                        tunnel: w2276 -> [w2304]
                        tunnel: [w2300] -> w2275
                        tunnel: [w2299] -> w2274
                        tunnel: [w2286] -> w2273
                        tunnel: w2272 -> [w2282]
                        i -> [w2291]
                        stop <- w2296 stop-if-true
                        # "If tether formed,\nimmediately change\nto new delta."
                        n1133 = local read "Fixed Y"() -> (w2281:dbl)
                        n1134 = local read "Fixed X"() -> (w2289:dbl)
                        n1135 = local read "Cutoff force (pN)"() -> (w2292:dbl)
                        n1136 = Multiply(x=w2305, y=w2291) -> (x*y=w2306:dbl)
                        n1137 = local read "Mean force (pN)"() -> (w2293:dbl)
                        n1138 = Add(x=w2304, y=w2306) -> (x+y=w2284:dbl)
                        n1139 = Select(t=w2281, s=w2290, f=w2289) -> (s? t:f=w2288:dbl)
                        n1140 = Greater?(x=w2293, y=w2292) -> (0:w2286:bool)
                        n1141 = Add(x=w2288, y="Delta after tether") -> (x+y=w2285:dbl)
                        n1142 = Select(t=w2285, s=w2286, f=w2284) -> (s? t:f=w2283:dbl)
                        n1143 = local read "Fish Speed (ms)"() -> (w2298:i32)
                        n1144 = Build Array(w2282, w2283) -> (w2303:dbl[])
                        n1145 = Build Array(w2283, w2282) -> (w2302:dbl[])
                        n1146 = Select(t=w2303, s=w2290, f=w2302) -> (s? t:f=w2301:dbl[])
                        n1147 = local read "Fish"() -> (w2295:bool)
                        n1148 = Greater Or Equal?(x=w2291, y=w2298) -> (x >= y?=w2297:bool)
                        n1149 = Not(x=w2295) -> (.not. x?=w2294:bool)
                        n1150 = call-poly <vilib>:"DAQmx Write.vi"("task/channels in"=w2308, "data"=w2301, "error in"=w2307) -> ("task out"=w2300:refnum<k21>, "error out"=w2299:errorcluster)  [unwired: 10 in, 1 out]
                        n1151 = Compound Arithmetic op=OR(w2297, w2294, w2286) -> (w2296:bool)
                      }
                    }
                  }
                }
              }
              n1152 = Add(x=w2162, y="Min fish\ndelta (V)") -> (x+y=w2169:dbl)
              n1153 = Decrement(x="# attempts") -> (x-1=w2178:dbl)
              n1154 = Greater Or Equal?(x=w2174, y=w2178) -> (x >= y?=w2177:bool)
              n1155 = local read "Mean force (pN)"() -> (w2176:dbl)
              n1156 = Greater?(x=w2176, y="Cutoff force (pN)") -> (0:w2171:bool)
              n1157 = Compound Arithmetic op=OR(w2156, w2171, w2177) -> (w2170:bool)
              n1158 = case shown="True" w2156 {
                frame False {
                }
                frame True {
                  n1159 = call <vilib>:"Beep.vi"() -> ()  [unwired: 12 in]
                }
              }
              n1160 = node-c288() -> ()  [unwired: 1 in, 1 out]
              "Tether" <- w2156
              "Attempt #" <- w2174
            }
            n1161 = node-c288(w2141) -> ()  [unwired: 1 out]
            n1162 = flat-sequence {
              tunnel: w2131 -> [w2149]
              tunnel: [w2149] -> w2130
              tunnel: w2129 -> [w2146]
              tunnel: w2128 -> [w2145]
              tunnel: w2127 -> [w2144]
              tunnel: w2130 -> [w2151]
              frame #0 {
                w2148 = T15 1 items=["no dialog", "OK message", "continue or stop message", "OK message + warnings", "continue/stop + warnings"] ("type of dialog (OK msg:1)")
                n1163 = call <vilib>:"DAQmx Clear Task.vi"("task in"=w2146, "error in"=w2145) -> ("error out"=w2147:errorcluster)  [unwired: 13 in]
                n1164 = Not(x=w2144) -> (.not. x?=w2143:bool)
                n1165 = local write "Fish"(w2143) -> ()
                n1166 = call <vilib>:"Simple Error Handler.vi"("type of dialog (OK msg:1)"=w2148, "error in (no error)"=w2147) -> ()  [unwired: 3 in, 5 out]
              }
              frame #1 {
                n1167 = And(x=w2151, y="Raster after\n tether?") -> (x .and. y?=w2152:bool)
                n1168 = case shown="True" w2152 {
                  selector: w2152 -> [_ w2153]
                  frame False {
                  }
                  frame True {
                    n1169 = property on="Raster scan" class="Bool (strict)"("Val(Sgnl)"=w2153) -> ()  [unwired: 2 in, 2 out]
                  }
                }
              }
            }
          }
        }
      }
      event "Load param": Value Change {
        n1170 = event-data() -> ()  [unwired: 1 in, 6 out]
        n1171 = property on="Scan Parameters" class="Arr (strict)"() -> ("Index Values"=w2324:u32[])  [unwired: 2 in, 2 out]
        n1172 = Index Array(array=w2324, index=0) -> (element=w2321:u32)
        n1173 = Index Array(array="Scan Parameters", index=w2321) -> (element=w2320:T18)
        n1174 = Unbundle(w2320) -> ("Max delta 2"=w2319:dbl, "Min delta 2"=w2315:dbl, "Speed (ms) 2"=w2318:i32, "# scans 2"=w2317:i32)  [unwired: 1 out]
        n1175 = property on="Max delta" class="DigNum (strict)"("Val(Sgnl)"=w2319) -> ()  [unwired: 2 in, 2 out]
        n1176 = local write "Load param"(FALSE ("Load param")) -> ()
        n1177 = property on="# scans" class="DigNum (strict)"("Val(Sgnl)"=w2317) -> ()  [unwired: 2 in, 2 out]
        n1178 = property on="Speed (ms)" class="DigNum (strict)"("Val(Sgnl)"=w2318) -> ()  [unwired: 2 in, 2 out]
        n1179 = property on="Min delta" class="DigNum (strict)"("Val(Sgnl)"=w2315) -> ()  [unwired: 2 in, 2 out]
      }
      event "Averaging Number": Value Change {
        n1180 = event-data() -> ()  [unwired: 1 in, 6 out]
        n1181 = local read "# Samples/channel (in)"() -> (w2328:i32)
        n1182 = local read "Averaging Number"() -> (w2326:i32)
        n1183 = Quotient & Remainder(x=w2328, y=w2326) -> (floor(x/y)=w2327:i32)  [unwired: 1 out]
        n1184 = Multiply(x=w2327, y=w2326) -> (x*y=w2325:i32)
        n1185 = local write "# Samples/channel (in)"(w2325) -> ()
      }
    }
    n1186 = node-c288() -> ()  [unwired: 1 in, 1 out]
  }
  n1187 = call <vilib>:"Simple Error Handler.vi"("error in (no error)"=w104) -> ()  [unwired: 4 in, 5 out]
  n1188 = node-c288() -> (w84:T12)  [unwired: 4 in]
  n1189 = timed-loop {
    timing: w84 -> [_]
    timing-out: [_] -> w83
    stop <- w2331 stop-if-true
    n1190 = node-c288() -> ()  [unwired: 1 in, 1 out]
    n1191 = event shown="[1] \"Stop\": Value Change" {
      selector: _ -> [_ _]
      dyn-events: _ -> [_ _]
      timeout: _ -> [_ _]
      tunnel: [_ "Stop"] -> w2331
      event Timeout {
        n1192 = event-data() -> ()  [unwired: 1 in, 2 out]
      }
      event "Stop": Value Change {
        n1193 = event-data() -> ()  [unwired: 1 in, 4 out]
      }
    }
    n1194 = node-c288() -> ()  [unwired: 1 in, 1 out]
  }
  n1195 = case shown="True" w73 {
    tunnel: w78 -> [_ w2337]
    tunnel: w77 -> [_ w2336]
    tunnel: w76 -> [_ w2335]
    frame False {
    }
    frame True {
      w2339 = T15 3 items=["no dialog", "OK message", "continue or stop message", "OK message + warnings", "continue/stop + warnings"] ("type of dialog (OK msg:1)")
      w2338 = T15 3 items=["no dialog", "OK message", "continue or stop message", "OK message + warnings", "continue/stop + warnings"] ("type of dialog (OK msg:1)")
      n1196 = call <vilib>:"DAQmx Clear Task.vi"("task in"=w2337, "error in"=w2335) -> ("error out"=w2340:errorcluster)  [unwired: 13 in]
      n1197 = call <vilib>:"DAQmx Clear Task.vi"("task in"=w2336) -> ("error out"=w2341:errorcluster)  [unwired: 14 in]
      n1198 = call <vilib>:"Simple Error Handler.vi"("type of dialog (OK msg:1)"=w2339, "error in (no error)"=w2340) -> ()  [unwired: 3 in, 5 out]
      n1199 = call <vilib>:"Simple Error Handler.vi"("type of dialog (OK msg:1)"=w2338, "error in (no error)"=w2341) -> ()  [unwired: 3 in, 5 out]
    }
  }
  n1200 = case shown="\"Force Feedback\", Default" "?" {
    frame "Force Feedback", Default {
    }
    frame "Raster scan" {
    }
  }
  n1201 = node-c288(w83) -> ()  [unwired: 1 out]
  n1202 = node-c288(w86) -> ()  [unwired: 1 out]
  n1203 = local write "Pause Mouse/Mirror Connection"(FALSE ("Pause Mouse/Mirror Connection")) -> ()
  n1204 = local write "Stop"(FALSE ("Stop all")) -> ()
  "CoordinatesMousePressed" <- T4 {"Horizontal"=0, "Vertical"=0} ("Coords when pressed")
  "Deflection" <- T4 {"Horizontal"=0, "Vertical"=0} ("Coords when pressed")
